vi "Current_Curve_Filtering.vi"() -> ()   [LabVIEW 2009]
uses:
  <vilib>/Analysis/3filter.llb/Butterworth Filter (DBL).vi
  Instance           3 31Saved   Current_vs_Length_2_log .vi
  Instance           2 31Saved   Current_vs_Length_2_log .vi
  <vilib>/Utility/file.llb/Write To Spreadsheet File (DBL).vi
  <vilib>/Utility/file.llb/Write To Spreadsheet File (I64).vi
  <vilib>/Analysis/NI_AALBase.lvlib
panel:
  out "residual":dbl=0.32609478757655186
  in  "Residual Cutoff Value":dbl=0.45
  out "XY Graph 3":cluster{dbl[], "Array":dbl[]}[](graph)
  in  "Save  2D Hist":bool
  out "G-Line":cluster{dbl[], i32[]}(graph)
  in  "Boolean":bool
  out "Cond. Max":dbl
  out "Cond. Min":dbl
  out "2D Histogram Max Values":cluster{sgl[], dbl[]}(graph)
  out "2D_G_Bins":dbl
  in  "PZT Sensitivty nm/V":dbl=3.89
  in  "Ramping Rate V/s":dbl=20.0
  out "Colormap 2":i32[][](graph)
  out "Current Bin2 (mV)":sgl=0.01
  out "Length Bin":sgl=0.015
  in  "log bins":i32=400
  out "XY Graph 2":cluster{dbl[], "Array":dbl[]}(graph)
  out "XY Graph":cluster{dbl[], "Array":dbl[]}(graph)
  out "Conductance (Go) 2":cluster{dbl, "SRat":dbl, "Filtered X":dbl[]}(graph)
  in  "Filter Freq":i32=9000
  in  "Units":bool
  in  "Bias Applied":dbl=0.1
  in  "Amplifier":dbl=1e-08
  in  "Copy Selected":bool
  in  "Subdirectory":string="Selected_Curves"
  out "String":string="Selection Criteria"
  in  "Step Height":i32=1
  in  "Decay":dbl=0.02
  in  "Max Counts":dbl=500000.0
  in  "Length %":i32=99
  in  "MIN":dbl=-2.0
  in  "MAX":dbl=0.9
  out "Curve Selected":bool
  out "shift value":dbl format="%.3f"
  in  "Zero calibrate":bool
  out "Linear Histogram":cluster{dbl, "Step":dbl, i32[]}(graph)
  out "Peak":cluster{dbl, "Step":dbl, i32[]}(graph)
  out "single":cluster{dbl, "Step":dbl, i32[]}(graph)
  out "writing to":path
  in  "TXT DIR":path=path "D:/Research/LabView/Processed_data"
  in  "Save TXT":bool
  out "Peak Histogram":cluster{dbl, "Step":dbl, i32[]}(graph)
  in  "Mode":bool=TRUE
  out "Total files":dbl
  in  "Current":u16
  in  "NEXT":bool
  in  "LAST":bool
  out "browsed":dbl
  out "selected":u16
  in  "add":bool
  in  "sub":bool
  in  "Peak Height":dbl=20.0 min=3.0 max=20.0 step=1.0
  in  "Peak width":i8=5 min=3 max=20 step=1
  in  "?":bool
  out "DL1520L-200mv":dbl[](array[numeric])=[1.0, 1.0, 1.0, 1.0, 1.0, 1.0, 1.0, 1.0, 1.0, 1.0, 1.0, 1.0, 1.0, 1.0, 1.0, 1.0, 1.0, 1.0, 1.0, 1.0, 1.0, 1.0, 1.0, 1.0, 1.0, 1.0, 1.0, 1.0, 1.0, 1.0, 1.0, 1.0, 1.0, 1.0, 1.0, 1.0, 1.0, 1.0, 1.0, 1.0, 1.0, 1.0, 1.0, 1.0, 1.0, 1.0, 1.0, 1.0, 1.0, 1.0, 1.0, 1.0, 1.0, 1.0, 1.0, 1.0, 1.0, 1.0, 1.0, 1.0, 1.0, 1.0, 1.0, 1.0, 1.0, 1.0, 1.0, 1.0, 1.0, 1.0, 1.0, 1.0, 1.0, 1.0, 1.0, 1.0, 1.0, 1.0, 1.0, 1.0, 1.0, 1.0, 1.0, 1.0, 1.0, 1.0, 1.0, 1.0, 1.0, 1.0, 1.0, 1.0, 1.0, 1.0, 1.0, 1.0, 1.0, 1.0, 1.0, 1.0, 1.0, 1.0, 1.0, 1.0, 1.0, 1.0, 1.0, 1.0, 1.0, 1.0, 1.0, 1.0, 1.0, 1.0, 1.0, 1.0, 1.0, 1.0, 1.0, 1.0, 1.0, 1.0, 1.0, 1.0, 1.0, 1.0518399477005005, 1.158460021018982, 0.8072500228881836, 1.076930046081543, 1.254330039024353, 0.9506000280380249, 1.0841000080108643, 0.7749999761581421, 1.0876799821853638, 1.0401999950408936, 1.1665300130844116, 1.0527399778366089, 0.8430899977684021, 1.1835500001907349, 1.0195900201797485, 1.0876799821853638, 1.0097299814224243, 0.8413000106811523, 0.9891300201416016, 1.0778299570083618, 1.100219964981079, 0.9317899942398071, 1.0894700288772583, 0.7767900228500366, 1.0661799907684326, 1.1916099786758423, 0.9022200107574463, 0.9631400108337402, 1.2498500347137451, 0.8654900193214417, 1.2104300260543823, 0.6486700177192688, 1.1190400123596191, 1.1217299699783325, 1.0097299814224243, 0.8081499934196472, 1.3242100477218628, 0.8063499927520752, 1.0751399993896484, 0.8905699849128723, 1.2713500261306763, 0.8583199977874756, 1.1504000425338745, 0.9237200021743774, 0.9694200158119202, 1.023169994354248, 1.017799973487854, 0.835919976234436, 0.9443299770355225, 1.2408900260925293, 0.8027700185775757, 1.0572199821472168, 1.1324800252914429, 1.07423996925354, 0.6997399926185608, 1.3197300434112549, 0.7803699970245361, 1.0267599821090698, 0.8511499762535095, 1.1512900590896606, 0.9559800028800964, 0.9909200072288513, 0.8009799718856812, 1.239989995956421, 1.0061500072479248, 0.936269998550415, 0.9577699899673462, 0.9774799942970276, 1.0751399993896484, 0.9640399813652039, 1.102910041809082, 0.8368200063705444, 0.946120023727417, 0.9828600287437439, 1.1208300590515137, 1.0527399778366089, 0.7418500185012817, 1.1943000555038452, 0.8395000100135803, 0.9676200151443481, 1.0410900115966797, 0.9936100244522095, 1.0043599605560303, 1.0195900201797485, 0.9201400279998779, 1.094849944114685, 0.8762400150299072, 0.9004300236701965, 1.0357199907302856, 1.1674200296401978, 0.9067000150680542, 1.0384000539779663, 0.8520500063896179, 1.1127699613571167, 0.9210399985313416, 0.9273099899291992, 0.8753399848937988, 1.0357199907302856, 1.179069995880127, 0.934469997882843, 1.0034600496292114, 1.1835500001907349, 0.7095900177955627, 0.9792699813842773, 1.1163500547409058, 0.8502600193023682, 1.1270999908447266, 1.0715500116348267, 0.8314399719238281, 1.155769944190979, 0.8771299719810486, 0.9335799813270569, 1.1199400424957275, 0.8350200057029724, 0.8681700229644775, 1.0831999778747559, 0.9299899935722351, 0.9532899856567383, 1.128000020980835, 0.8054599761962891, 1.0052499771118164, 1.128000020980835, 0.9138699769973755, 1.0142099857330322, 0.9057999849319458, 1.0939500331878662, 0.7526000142097473, 1.223870038986206, 0.7741000056266785, 1.023169994354248, 1.1781699657440186, 0.8332300186157227, 0.7955999970436096, 1.07423996925354, 1.0554300546646118, 0.9443299770355225, 0.9604600071907043, 1.1217299699783325, 0.9335799813270569, 0.9586700201034546, 0.8126299977302551, 1.0213799476623535, 0.9774799942970276, 1.0034600496292114, 0.997189998626709, 0.8511499762535095, 1.280310034751892, 0.857420027256012, 1.179960012435913, 0.8887799978256226, 0.8395000100135803, 0.8395000100135803, 1.2265499830245972, 0.8932600021362305, 0.9057999849319458, 1.0401999950408936, 0.8520500063896179, 1.2059500217437744, 1.0823099613189697, 0.6755499839782715, 1.1315799951553345, 0.9201400279998779, 1.0312399864196777, 0.8162099719047546, 1.2632900476455688, 0.976580023765564, 1.016010046005249, 0.9255099892616272, 1.1226199865341187, 0.7230299711227417, 1.3636300563812256, 0.7042199969291687, 1.1351699829101562, 0.9452300071716309, 1.0061500072479248, 0.9559800028800964, 1.062600016593933, 0.8466699719429016, 1.0581200122833252, 0.9479100108146667, 0.9909200072288513, 0.7741000056266785, 1.1736899614334106, 0.8045600056648254, 1.2032599449157715, 1.158460021018982, 0.8296499848365784, 1.0124200582504272, 0.9255099892616272, 0.9936100244522095, 1.097540020942688, 0.955079972743988, 1.0849900245666504, 0.8117300271987915, 1.0491600036621094, 1.062600016593933, 0.8224800229072571, 0.9658300280570984, 1.2722500562667847, 0.809939980506897, 1.1154600381851196, 0.8072500228881836, 1.017799973487854, 1.0384000539779663, 1.0652799606323242, 1.0321300029754639, 0.8466699719429016, 1.1136599779129028, 0.9479100108146667, 1.1736899614334106, 0.8654900193214417, 1.0491600036621094, 0.908490002155304, 1.0831999778747559, 0.8887799978256226, 1.417389988899231, 0.7920200228691101, 0.9299899935722351, 1.050950050354004, 0.9210399985313416, 1.2131099700927734, 1.0554300546646118, 0.9326800107955933, 1.0410900115966797, 1.0124200582504272, 0.7723100185394287, 1.14860999584198, 0.9183499813079834, 1.258810043334961, 1.1387499570846558, 0.7615600228309631, 1.0536400079727173, 1.0912699699401855, 1.1055999994277954, 0.9864400029182434, 1.102020025253296, 0.8395000100135803, 1.0518399477005005, 1.1647299528121948, 1.0536400079727173, 1.0903700590133667, 0.898639976978302, 1.0706599950790405, 0.8798199892044067, 1.2086299657821655, 1.2175899744033813, 0.9685199856758118, 0.9299899935722351, 1.2453700304031372, 0.9183499813079834, 1.0683399438858032, 1.1099599599838257, 0.8287299871444702, 1.1348299980163574, 1.1777299642562866, 1.002619981765747, 1.064460039138794, 0.7911900281906128, 1.0801000595092773, 1.0354299545288086, 1.1541199684143066, 1.0330699682235718, 0.8758800029754639, 1.143239974975586, 1.060479998588562, 1.069390058517456, 0.988099992275238, 0.8736900091171265, 0.9702600240707397, 1.0806699991226196, 1.105430006980896, 0.9094799757003784, 1.1135200262069702, 0.7833700180053711, 1.0633599758148193, 1.1603599786758423, 0.9031000137329102, 0.9701399803161621, 1.233780026435852, 0.8961600065231323, 1.1906499862670898, 0.6593499779701233, 1.1051499843597412, 1.1458200216293335, 0.9879999756813049, 0.8049200177192688, 1.3313599824905396, 0.8278599977493286, 1.0381699800491333, 0.9175699949264526, 1.2579900026321411, 0.8616999983787537, 1.143380045890808, 0.9292100071907043, 0.9623799920082092, 1.0555200576782227, 0.9838700294494629, 0.858959972858429, 0.9398900270462036, 1.2190099954605103, 0.8296499848365784, 1.0342299938201904, 1.13742995262146, 1.0622600317001343, 0.6929500102996826, 1.3546600341796875, 0.7598299980163574, 1.0298999547958374, 0.8505499958992004, 1.1496700048446655, 0.9482600092887878, 0.9879999756813049, 0.8200399875640869, 1.221750020980835, 0.992609977722168, 0.9523800015449524, 0.9264600276947021, 1.0212299823760986, 1.0299400091171265, 1.0182199478149414, 1.0560100078582764, 0.8834599852561951, 0.9059699773788452, 0.9895399808883667, 1.1484400033950806, 1.0384600162506104, 0.7316499948501587, 1.2115099430084229, 0.8419600129127502, 0.9686800241470337, 1.0195599794387817, 1.006790041923523, 1.0077199935913086, 0.9961599707603455, 0.9295700192451477, 1.091230034828186, 0.8798800110816956, 0.879580020904541, 1.0691100358963013, 1.1512999534606934, 0.9050300121307373, 1.054460048675537, 0.8385900259017944, 1.1123000383377075, 0.9119399785995483, 0.9419999718666077, 0.8851900100708008, 1.0197900533676147, 1.2030800580978394, 0.9083799719810486, 1.001520037651062, 1.2015999555587769, 0.6734499931335449, 1.0091999769210815, 1.102139949798584, 0.844539999961853, 1.1170300245285034, 1.064460039138794, 0.840470016002655, 1.149649977684021, 0.9002000093460083, 0.9479600191116333, 1.1135799884796143, 0.8381400108337402, 0.8478099703788757, 1.1067700386047363, 0.9128299951553345, 0.959659993648529, 1.1379300355911255, 0.7703099846839905, 1.0372799634933472, 1.107100009918213, 0.9234399795532227, 1.0169399976730347, 0.9108999967575073, 1.0801399946212769, 0.7652300000190735, 1.2206100225448608, 0.7879800200462341, 0.985759973526001, 1.2073700428009033, 0.8196899890899658, 0.804069995880127, 1.0743099451065063, 1.0461499691009521, 0.969980001449585, 0.9197400212287903, 1.1764299869537354, 0.89205002784729, 1.0055299997329712, 0.7935699820518494, 0.976859986782074, 1.006100058555603, 0.9770500063896179, 1.037160038948059, 0.8456100225448608, 1.2542500495910645, 0.8690800070762634, 1.1796799898147583, 0.880840003490448, 0.8596900105476379, 0.8223699927330017, 1.2430599927902222, 0.8662499785423279, 0.9478700160980225, 0.995389997959137, 0.9024500250816345, 1.200219988822937, 1.085710048675537, 0.6602299809455872, 1.1301900148391724, 0.9190300107002258, 1.029270052909851, 0.8400899767875671, 1.2397899627685547, 0.9429399967193604, 1.075279951095581, 0.8741999864578247, 1.184149980545044, 0.698360025882721, 1.3655699491500854, 0.7038400173187256, 1.114150047302246, 0.9856600165367126, 0.9702000021934509, 0.9700400233268738, 1.0714000463485718, 0.8154500126838684, 1.068910002708435, 0.9287599921226501, 0.9945600032806396, 0.7877600193023682, 1.1730799674987793, 0.8385400176048279, 1.1815299987792969, 1.1555500030517578, 0.8173999786376953, 0.9916300177574158, 0.9548199772834778, 0.9830399751663208, 1.1294000148773193, 0.9332299828529358, 1.129930019378662, 0.7542799711227417, 1.0674200057983398, 1.0660799741744995, 0.8366600275039673, 0.9412099719047546, 1.3048499822616577, 0.773169994354248, 1.1747000217437744, 0.7867599725723267, 1.0328500270843506, 1.008679986000061, 1.0926100015640259, 0.9909200072288513, 0.8855100274085999, 1.0829600095748901, 0.9591699838638306, 1.1888200044631958, 0.8604199886322021, 1.042580008506775, 0.8842300176620483, 1.092270016670227, 0.9145799875259399, 1.4063600301742554, 0.780019998550415, 0.9580699801445007, 1.0166599750518799, 0.9434900283813477, 1.209130048751831, 1.0414999723434448, 0.9523000121116638, 1.0370899438858032, 1.0564299821853638, 0.7244799733161926, 1.1851400136947632, 0.8989599943161011, 1.2469799518585205, 1.16989004611969, 0.7621200084686279, 1.055299997329712, 1.073009967803955, 1.1236900091171265, 1.0108699798583984, 1.057569980621338, 0.8584499955177307, 1.0296599864959717, 1.1820800304412842, 1.0370500087738037, 1.086899995803833, 0.9445199966430664, 1.0530200004577637, 0.8767600059509277, 1.1927000284194946, 1.2465300559997559, 0.9571999907493591, 0.9764000177383423, 1.195989966392517, 0.9126899838447571, 1.0990899801254272, 1.0919599533081055, 0.8234300017356873, 1.1401300430297852, 1.1347800493240356, 1.0098799467086792, 1.0518100261688232, 0.781499981880188, 1.1401300430297852, 1.0295100212097168, 1.1410200595855713, 1.0250500440597534, 0.8823099732398987, 1.1267499923706055, 1.0188000202178955, 1.0482399463653564, 1.0464600324630737, 0.8724899888038635, 0.9956099987030029, 1.0625200271606445, 1.0919599533081055, 0.9313700199127197, 1.0580600500106812, 0.78507000207901, 1.0464600324630737, 1.1642199754714966, 0.9599199891090393, 0.9465399980545044, 1.2418299913406372, 0.8894400000572205, 1.2088199853897095, 0.6503599882125854, 1.043779969215393, 1.1802799701690674, 0.9527900218963623, 0.8573300242424011, 1.3248000144958496, 0.8341299891471863, 1.031290054321289, 0.9090700149536133, 1.2614599466323853, 0.8055899739265442, 1.1285300254821777, 0.9866899847984314, 0.9536799788475037, 1.084820032119751, 0.9634900093078613, 0.8662499785423279, 0.9206699728965759, 1.192770004272461, 0.8448399901390076, 0.9982799887657166, 1.1829500198364258, 1.0455700159072876, 0.717270016670227, 1.3444299697875977, 0.7707899808883667, 1.0375399589538574, 0.8109400272369385, 1.1454800367355347, 0.9358299970626831, 0.9768700003623962, 0.8457300066947937, 1.255210041999817, 1.013450026512146, 0.9197800159454346, 0.9340500235557556, 1.0170199871063232, 0.9804400205612183, 1.0232599973678589, 1.0446699857711792, 0.9206699728965759, 0.9162099957466125, 0.9643800258636475, 1.1918699741363525, 1.0081000328063965, 0.7395700216293335, 1.1802799701690674, 0.8189700245857239, 0.9527900218963623, 1.0366400480270386, 1.0455700159072876, 1.0179100036621094, 1.0000699758529663, 0.9019299745559692, 1.1267499923706055, 0.8484100103378296, 0.8510800004005432, 1.0642999410629272, 1.1553000211715698, 0.9117500185966492, 1.09552001953125, 0.8368099927902222, 1.1178300380706787, 0.9028300046920776, 0.92781001329422, 0.8644700050354004, 1.0009599924087524, 1.1767100095748901, 0.9304800033569336, 1.0196900367736816, 1.2079299688339233, 0.690500020980835, 1.0321799516677856, 1.0839300155639648, 0.8260999917984009, 1.0883899927139282, 1.0616199970245361, 0.8430500030517578, 1.1829500198364258, 0.9206699728965759, 0.9179900288581848, 1.1651099920272827, 0.8082600235939026, 0.852869987487793, 1.0732200145721436, 0.8831999897956848, 0.9706299901008606, 1.1722500324249268, 0.7743600010871887, 1.0286200046539307, 1.09552001953125, 0.9679499864578247, 0.9938200116157532, 0.8760600090026855, 1.0544899702072144, 0.7440299987792969, 1.2873300313949585, 0.7922000288963318, 0.9938200116157532, 1.16867995262146, 0.830560028553009, 0.8484100103378296, 1.013450026512146, 1.0411100387573242, 0.9518899917602539, 0.9340500235557556, 1.2150700092315674, 0.8948000073432922, 1.0152299404144287, 0.7823899984359741, 0.9848999977111816, 1.0107699632644653, 0.9260200262069702, 1.0473500490188599, 0.8037999868392944, 1.3372900485992432, 0.8600000143051147, 1.192770004272461, 0.9019299745559692, 0.8270000219345093, 0.8314599990844727, 1.2284499406814575, 0.8368099927902222, 0.9153199791908264, 1.0268299579620361, 0.9206699728965759, 1.204360008239746, 1.1178300380706787, 0.6342999935150146, 1.1445900201797485, 0.9028300046920776, 0.9840099811553955, 0.835919976234436, 1.2712700366973877, 0.9857900142669678, 1.0491299629211426, 0.9090700149536133, 1.1740299463272095, 0.6922900080680847, 1.3515599966049194, 0.6717699766159058, 1.1097999811172485, 0.9902499914169312, 1.006309986114502, 0.9724100232124329, 1.0812499523162842, 0.8055899739265442, 1.067870020866394, 0.9295899868011475, 0.9857900142669678, 0.7511699795722961, 1.1704599857330322, 0.8912299871444702, 1.2061500549316406, 1.1294300556182861, 0.8385900259017944, 0.9795500040054321, 0.9643800258636475, 0.9857900142669678, 1.0642999410629272, 0.9304800033569336, 1.157080054283142, 0.7797099947929382, 1.09552001953125, 1.0660799741744995, 0.8189700245857239, 0.9492200016975403, 1.2784099578857422, 0.7707899808883667, 1.1722500324249268, 0.7725800275802612, 1.0892800092697144, 1.0107699632644653, 1.0892800092697144, 1.0081000328063965, 0.8501899838447571, 1.09552001953125, 0.9340500235557556, 1.1633299589157104, 0.8805199861526489, 1.0687600374221802, 0.8885499835014343, 1.1115800142288208, 0.9224500060081482, 1.3872499465942383, 0.7743600010871887, 0.9260200262069702, 0.9875800013542175, 0.9617099761962891, 1.2596700191497803, 1.0580600500106812, 0.9233499765396118, 1.0616199970245361, 1.0482399463653564, 0.7654399871826172, 1.1115800142288208, 0.9028300046920776, 1.2596700191497803, 1.2052600383758545, 0.7743600010871887, 1.0339699983596802, 1.0990899801254272, 1.104449987411499, 1.0339699983596802, 1.0188000202178955, 0.8323500156402588, 1.0651899576187134, 1.183840036392212, 1.0687600374221802, 1.0634100437164307, 0.9572499990463257, 1.0553799867630005, 0.8510800004005432, 1.166890025138855, 1.2543200254440308, 1.0027400255203247, 0.9777600169181824, 1.2338000535964966, 0.8787400126457214, 1.0004299879074097, 1.0473099946975708, 0.8730499744415283, 1.1065800189971924, 1.1543400287628174, 1.0278500318527222, 1.0384700298309326, 0.7819499969482422, 1.0747300386428833, 1.0570399761199951, 1.1286900043487549, 1.0402300357818604, 0.8774799704551697, 1.1746900081634521, 1.0322699546813965, 1.0375800132751465, 0.9995499849319458, 0.8394399881362915, 0.9862800240516663, 1.095960021018982, 1.0676599740982056, 0.9376299977302551, 1.0835800170898438, 0.8164399862289429, 1.0092799663543701, 1.1764600276947021, 0.9243599772453308, 0.9287800192832947, 1.2631399631500244, 0.8704000115394592, 1.204759955406189, 0.6474900245666504, 1.089769959449768, 1.1348799467086792, 0.979200005531311, 0.8385599851608276, 1.292330026626587, 0.8535900115966797, 1.0022000074386597, 0.9323199987411499, 1.257830023765564, 0.8182100057601929, 1.1693799495697021, 0.9279000163078308, 0.9508900046348572, 1.0641200542449951, 0.9836199879646301, 0.863319993019104, 0.9013599753379822, 1.2472200393676758, 0.784600019454956, 1.0535000562667847, 1.1454999446868896, 1.0526200532913208, 0.6864100098609924, 1.3498300313949585, 0.7739800214767456, 1.011929988861084, 0.9004799723625183, 1.1233799457550049, 0.9208199977874756, 0.9977800250053406, 0.7890200018882751, 1.2649099826812744, 0.9756600260734558, 0.9340900182723999, 0.979200005531311, 0.9482399821281433, 1.094190001487732, 0.9738900065422058, 1.065000057220459, 0.858020007610321, 0.8951699733734131, 1.0322699546813965, 1.1366499662399292, 1.0313899517059326, 0.7173699736595154, 1.207419991493225, 0.856249988079071, 0.9447000026702881, 1.0499600172042847, 0.980970025062561, 0.9898200035095215, 1.0048500299453735, 0.896049976348877, 1.1348799467086792, 0.8624399900436401, 0.890749990940094, 1.063230037689209, 1.1375399827957153, 0.9349700212478638, 0.9986600279808044, 0.8748199939727783, 1.089769959449768, 0.9517800211906433, 0.9155099987983704, 0.888979971408844, 1.0437699556350708, 1.1543400287628174, 0.9376299977302551, 0.9641600251197815, 1.2295299768447876, 0.6722599864006042, 0.9615100026130676, 1.141070008277893, 0.8385599851608276, 1.1313400268554688, 1.0561599731445312, 0.8350200057029724, 1.1693799495697021, 0.863319993019104, 0.9765499830245972, 1.098620057106018, 0.850059986114502, 0.8367900252342224, 1.124269962310791, 0.8969399929046631, 0.9632800221443176, 1.1171900033950806, 0.7881399989128113, 1.011929988861084, 1.1419600248336792, 0.8872100114822388, 1.0871200561523438, 0.8659800291061401, 1.095960021018982, 0.7952100038528442, 1.1605299711227417, 0.8102499842643738, 0.9641600251197815, 1.2153799533843994, 0.8102499842643738, 0.8111400008201599, 1.0756200551986694, 1.0296200513839722, 0.9898200035095215, 0.9137399792671204, 1.1985700130462646, 0.8836699724197388, 0.9915800094604492, 0.7996399998664856, 0.9632800221443176, 1.0340399742126465, 0.9986600279808044, 0.9933500289916992, 0.8765900135040283, 1.210070013999939, 0.9146299958229065, 1.1640700101852417, 0.8863199949264526, 0.8827800154685974, 0.8137900233268738, 1.2507599592208862, 0.8624399900436401, 0.938510000705719, 1.0384700298309326, 0.8456299901008606, 1.2259900569915771, 1.0331599712371826, 0.6828799843788147, 1.1870700120925903, 0.863319993019104, 1.0526200532913208, 0.8235200047492981, 1.2560700178146362, 0.9447000026702881, 1.065000057220459, 0.9225900173187256, 1.1366499662399292, 0.7359499931335449, 1.3002899885177612, 0.7456799745559692, 1.1472699642181396, 0.9606299996376038, 1.0048500299453735, 0.938510000705719, 1.091539978981018, 0.8049399852752686, 1.0818099975585938, 0.9323199987411499, 0.9800900220870972, 0.8208699822425842, 1.1295700073242188, 0.8739399909973145, 1.1499199867248535, 1.1861900091171265, 0.8093699812889099, 1.0004299879074097, 0.9924700260162354, 0.9349700212478638, 1.1384199857711792, 0.9588599801063538, 1.098620057106018, 0.815559983253479, 1.011929988861084, 1.1056900024414062, 0.8535900115966797, 0.929669976234436, 1.2994099855422974, 0.7775200009346008, 1.1897200345993042, 0.7757499814033508, 1.0375800132751465, 1.015470027923584, 1.1171900033950806, 0.9623900055885315, 0.8712900280952454, 1.1207300424575806, 0.9323199987411499, 1.239259958267212, 0.8288300037384033, 1.0597000122070312, 0.902239978313446, 1.065000057220459, 0.9358599781990051, 1.3834400177001953, 0.8014100193977356, 0.9853900074958801, 1.0022000074386597, 0.9668200016021729, 1.2286399602890015, 1.0526200532913208, 0.904009997844696, 1.0853500366210938, 1.0420000553131104, 0.7262200117111206, 1.1932599544525146, 0.9199399948120117, 1.2693300247192383, 1.1348799467086792, 0.8022900223731995, 1.0181200504302979, 1.122499942779541, 1.1127699613571167, 1.0145800113677979, 1.0667699575424194, 0.8332499861717224, 1.0579299926757812, 1.172029972076416, 1.0623500347137451, 1.0773899555206299, 0.9588599801063538, 1.0313899517059326, 0.9119700193405151, 1.205649971961975, 1.2675700187683105, 0.9323199987411499, 0.9712399840354919, 1.2436800003051758, 0.8810200095176697, 1.0145000219345093, 1.1491299867630005, 0.798229992389679, 1.130020022392273, 1.1474000215530396, 1.0066900253295898, 1.0310100317001343, 0.7556700110435486, 1.1222100257873535, 0.9745500087738037, 1.1830099821090698, 0.9910500049591064, 0.8894299864768982, 1.1022299528121948, 1.065750002861023, 1.0570600032806396, 0.9988700151443481, 0.8373100161552429, 0.9641299843788147, 1.0631400346755981, 1.0987600088119507, 0.902459979057312, 1.0900700092315674, 0.778249979019165, 1.0822499990463257, 1.130020022392273, 0.9007200002670288, 0.9276400208473206, 1.2246999740600586, 0.9007200002670288, 1.1908199787139893, 0.6219000220298767, 1.0961500406265259, 1.152609944343567, 0.9936599731445312, 0.7773799896240234, 1.297659993171692, 0.8468700051307678, 1.0344799757003784, 0.877269983291626, 1.2559700012207031, 0.8920300006866455, 1.1256799697875977, 0.9137499928474426, 0.9224299788475037, 1.0553300380706787, 0.9832299947738647, 0.8494700193405151, 0.9163500070571899, 1.2386000156402588, 0.781719982624054, 1.0327399969100952, 1.1647700071334839, 1.017109990119934, 0.7209200263023376, 1.3254499435424805, 0.7652199864387512, 1.0118999481201172, 0.823419988155365, 1.1482599973678589, 0.9502300024032593, 0.9832299947738647, 0.8138599991798401, 1.2116700410842896, 0.991919994354248, 0.931119978427887, 0.9537000060081482, 0.9693400263786316, 1.0666199922561646, 0.9884499907493591, 1.0466400384902954, 0.8928999900817871, 0.8824800252914429, 0.9910500049591064, 1.153480052947998, 1.0006099939346313, 0.7426400184631348, 1.1847399473190308, 0.8711900115013123, 0.9372000098228455, 1.0092899799346924, 1.0006099939346313, 0.9936599731445312, 0.9927899837493896, 0.9372000098228455, 1.0683499574661255, 0.8850799798965454, 0.8850799798965454, 1.0709600448608398, 1.143049955368042, 0.8824800252914429, 1.047510027885437, 0.8659800291061401, 1.0874600410461426, 0.9172199964523315, 0.9198300242424011, 0.9015899896621704, 1.0414299964904785, 1.173449993133545, 0.9215599894523621, 0.9606500267982483, 1.2134100198745728, 0.6549100279808044, 0.9728099703788757, 1.1395800113677979, 0.8164700269699097, 1.1639000177383423, 1.0145000219345093, 0.8633700013160706, 1.155210018157959, 0.8729199767112732, 0.9797599911689758, 1.072700023651123, 0.8659800291061401, 0.8355799913406372, 1.0961500406265259, 0.9120100140571594, 0.9450200200080872, 1.168239951133728, 0.738290011882782, 1.0579299926757812, 1.081380009651184, 0.9224299788475037, 1.0231900215148926, 0.9250400066375732, 1.0718300342559814, 0.7478500008583069, 1.230780005455017, 0.7756400108337402, 0.9806299805641174, 1.2194900512695312, 0.8112499713897705, 0.8225499987602234, 1.0466400384902954, 1.0631400346755981, 0.9571800231933594, 0.9180899858474731, 1.2047200202941895, 0.8790000081062317, 1.0075500011444092, 0.7843300104141235, 0.9623900055885315, 1.0275299549102783, 0.9632599949836731, 1.0483800172805786, 0.8242800235748291, 1.295050024986267, 0.8651099801063538, 1.2012499570846558, 0.8790000081062317, 0.8295000195503235, 0.8485999703407288, 1.1830099821090698, 0.9172199964523315, 0.9450200200080872, 0.9988700151443481, 0.8972399830818176, 1.1908199787139893, 1.09961998462677, 0.6722800135612488, 1.1265499591827393, 0.9207000136375427, 1.0362199544906616, 0.8668400049209595, 1.1943000555038452, 0.9927899837493896, 1.0370899438858032, 0.9250400066375732, 1.1639000177383423, 0.6887800097465515, 1.3680200576782227, 0.7209200263023376, 1.1152600049972534, 0.9962599873542786, 0.9867100119590759, 0.9597799777984619, 1.0970200300216675, 0.8208100199699402, 1.0492500066757202, 0.9502300024032593, 0.9815000295639038, 0.817330002784729, 1.1639000177383423, 0.8190699815750122, 1.216879963874817, 1.1474000215530396, 0.8642399907112122, 0.9597799777984619, 0.9754199981689453, 0.9945300221443176, 1.1169999837875366, 0.9597799777984619, 1.1057000160217285, 0.7851999998092651, 1.074429988861084, 1.0631400346755981, 0.8520799875259399, 0.9484900236129761, 1.3341399431228638, 0.763480007648468, 1.2012499570846558, 0.7834600210189819, 1.0448999404907227, 1.0266599655151367, 1.0865999460220337, 0.9710699915885925, 0.8833500146865845, 1.1196000576019287, 1.010159969329834, 1.18996000289917, 0.8685799837112427, 1.02839994430542, 0.9015899896621704, 1.111780047416687, 0.9302499890327454, 1.419260025024414, 0.7660899758338928, 0.991919994354248, 1.0318700075149536, 0.9545699954032898, 1.2099299430847168, 1.0518499612808228, 0.9519699811935425, 1.0527199506759644, 1.0614099502563477, 0.7660899758338928, 1.1569499969482422, 0.9641299843788147, 1.2377300262451172, 1.1882200241088867, 0.763480007648468, 1.0587999820709229, 1.111780047416687, 1.1378400325775146, 1.0344799757003784, 1.0527199506759644, 0.8963800072669983, 1.037950038909912, 1.210800051689148, 1.0145000219345093, 1.1126500368118286, 0.9623900055885315, 1.069219946861267, 0.9276400208473206, 1.153480052947998, 1.3150299787521362, 0.956309974193573, 0.9884499907493591, 1.2246999740600586, 0.9154800176620483, 1.0553300380706787, 1.0, 1.0, 1.0, 1.0, 1.0, 1.0, 1.0, 1.0, 1.0, 1.0, 1.0, 1.0, 1.0, 1.0, 1.0, 1.0, 1.0, 1.0, 1.0, 1.0, 1.0, 1.0, 1.0, 1.0, 1.0, 1.0, 1.0, 1.0, 1.0, 1.0, 1.0, 1.0, 1.0, 1.0, 1.0, 1.0, 1.0, 1.0, 1.0, 1.0, 1.0, 1.0, 1.0, 1.0, 1.0, 1.0, 1.0, 1.0, 1.0, 1.0, 1.0, 1.0, 1.0, 1.0, 1.0, 1.0, 1.0, 1.0, 1.0, 1.0, 1.0, 1.0, 1.0, 1.0, 1.0, 1.0, 1.0, 1.0, 1.0, 1.0, 1.0, 1.0, 1.0, 1.0, 1.0, 1.0, 1.0, 1.0, 1.0, 1.0, 1.0, 1.0, 1.0, 1.0, 1.0, 1.0, 1.0, 1.0, 1.0, 1.0, 1.0, 1.0, 1.0, 1.0, 1.0, 1.0, 1.0, 1.0, 1.0, 1.0, 1.0, 1.0, 1.0, 1.0, 1.0, 1.0, 1.0, 1.0, 1.0, 1.0, 1.0, 1.0, 1.0, 1.0, 1.0, 1.0, 1.0, 1.0, 1.0, 1.0, 1.0, 1.0, 1.0, 1.0] format="%.4f"
  in  "NIDL Correction":T1(ring)
  out "DL1520L-2V":dbl[](array[numeric])=[1.0, 1.0, 1.1071499586105347, 0.9460300207138062, 1.142799973487854, 1.0548499822616577, 0.6798099875450134, 1.1869399547576904, 0.9574499726295471, 1.0553699731826782, 0.9193099737167358, 1.0121500492095947, 0.8809400200843811, 0.8933200240135193, 1.2142599821090698, 0.9320200085639954, 0.867389976978302, 1.04121994972229, 0.8392800092697144, 1.3207199573516846, 0.8761799931526184, 0.9614599943161011, 0.8406999707221985, 1.3237199783325195, 0.842270016670227, 0.8019999861717224, 1.0565799474716187, 0.8988800048828125, 0.9938300251960754, 0.9866300225257874, 0.9458100199699402, 1.0645899772644043, 0.9812700152397156, 0.9915500283241272, 1.047860026359558, 0.7784900069236755, 0.9436100125312805, 1.1797200441360474, 0.9229199886322021, 0.8316299915313721, 1.06072998046875, 1.0812599658966064, 0.8902999758720398, 0.992579996585846, 0.983020007610321, 0.9313600063323975, 1.0070199966430664, 0.85794997215271, 1.0585600137710571, 0.8302099704742432, 1.0535399913787842, 1.0813499689102173, 1.0289100408554077, 0.7472900152206421, 0.977429986000061, 0.9230499863624573, 1.1730200052261353, 0.938759982585907, 0.6154199838638306, 1.0446100234985352, 1.1901600360870361, 0.8682100176811218, 0.9817299842834473, 0.950410008430481, 1.0137699842453003, 0.9678400158882141, 1.1657299995422363, 1.0292799472808838, 0.7897499799728394, 0.8259699940681458, 0.8726199865341187, 1.1850299835205078, 0.9300100207328796, 1.0324499607086182, 0.8647400140762329, 0.9773200154304504, 1.0006699562072754, 0.9293299913406372, 0.8785300254821777, 1.0564700365066528, 0.9852399826049805, 0.9670900106430054, 0.9886400103569031, 0.8383399844169617, 1.0759299993515015, 0.8722000122070312, 1.1963000297546387, 0.9250400066375732, 0.7123000025749207, 1.14274001121521, 1.097190022468567, 0.8719499707221985, 0.9584500193595886, 0.9225000143051147, 1.074280023574829, 1.0170899629592896, 0.756659984588623, 1.2385200262069702, 0.7658299803733826, 1.049090027809143, 0.8378199934959412, 1.1470099687576294, 0.8785899877548218, 0.9787899851799011, 1.00246000289917, 0.8198699951171875, 1.0823800563812256, 0.9904900193214417, 1.1441099643707275, 0.8393700122833252, 0.9125199913978577, 1.0177700519561768, 1.0600700378417969, 0.8316599726676941, 1.1464899778366089, 0.8072400093078613, 0.855400025844574, 1.0888500213623047, 1.0, 1.1690200567245483, 0.7053999900817871, 0.9819300174713135, 1.173799991607666, 0.8808599710464478, 1.0376299619674683, 0.883840024471283, 0.9901099801063538, 1.1312099695205688, 0.9692599773406982, 0.9967600107192993, 0.765720009803772, 1.2453299760818481, 0.8936399817466736, 1.043470025062561, 0.9276000261306763, 1.2058199644088745, 0.8945900201797485, 1.0330699682235718, 0.8693199753761292, 1.1636600494384766, 1.1312199831008911, 0.9562699794769287, 0.8316500186920166, 0.9096199870109558, 1.2192000150680542, 1.0195599794387817, 0.9311000108718872, 1.1465500593185425, 1.0913599729537964, 0.8537700176239014, 1.3184200525283813, 0.9644500017166138, 1.0194200277328491, 0.9502500295639038, 1.0557500123977661, 1.1233799457550049, 0.8309900164604187, 1.0903799533843994, 1.1363199949264526, 0.992169976234436, 1.0392800569534302, 1.0482699871063232, 0.9170600175857544, 1.1024999618530273, 1.0506600141525269, 1.0036300420761108, 1.1565699577331543, 0.7453500032424927, 1.1898800134658813, 0.8898800015449524, 1.207360029220581, 0.9647600054740906, 0.9409199953079224, 1.1513999700546265, 1.0830199718475342, 1.3117300271987915] format="%.5f"
  out "DL1520-2V":dbl[](array[numeric])=[0.9042699933052063, 0.8751500248908997, 1.1938999891281128, 0.8774200081825256, 1.1261299848556519, 1.0424100160598755, 0.8799999952316284, 0.9431099891662598, 1.1161799430847168, 0.9157999753952026, 1.1118199825286865, 1.0853400230407715, 0.983240008354187, 0.9828400015830994, 1.0612900257110596, 0.9332299828529358, 1.1189700365066528, 0.6911799907684326, 1.215109944343567, 0.921750009059906, 1.158869981765747, 0.8488900065422058, 1.0097500085830688, 1.0497299432754517, 0.8821499943733215, 1.0121699571609497, 1.2015700340270996, 0.8813199996948242, 0.9427800178527832, 0.9210500121116638, 1.036810040473938, 0.9211099743843079, 1.117069959640503, 0.9027000069618225, 1.030769944190979, 0.8944699764251709, 1.1112699508666992, 0.7450199723243713, 1.0670100450515747, 0.9704999923706055, 1.2049299478530884, 0.7958400249481201, 1.03410005569458, 0.8904100060462952, 0.8966599702835083, 1.0761699676513672, 0.784529983997345, 1.103909969329834, 0.9223999977111816, 1.0275700092315674, 0.914080023765564, 1.137220025062561, 0.8187599778175354, 0.9508200287818909, 1.1327999830245972, 0.8613799810409546, 1.0511300563812256, 1.0065900087356567, 0.9020299911499023, 1.0810799598693848, 1.08132004737854, 0.941789984703064, 0.8384000062942505, 0.845770001411438, 1.0647200345993042, 1.0405399799346924, 0.9768400192260742, 0.9739000201225281, 0.9725599884986877, 1.0460799932479858, 0.9323800206184387, 1.0303699970245361, 0.9656699895858765, 0.9442600011825562, 1.0794600248336792, 0.8691499829292297, 0.9040200114250183, 1.1154099702835083, 0.9336199760437012, 1.0413199663162231, 1.0063899755477905, 0.8839600086212158, 0.9992200136184692, 1.046839952468872, 0.9423099756240845, 1.0822499990463257, 0.8034200072288513, 1.0724799633026123, 0.8759899735450745, 1.0159300565719604, 1.0274300575256348, 0.9268100261688232, 1.0325599908828735, 0.990809977054596, 1.055459976196289, 1.0155099630355835, 0.7494500279426575, 1.001710057258606, 0.9849399924278259, 1.1800999641418457, 1.0796300172805786, 0.6667100191116333, 1.0151100158691406, 1.0528500080108643, 0.9521200060844421, 1.0733100175857544, 0.827530026435852, 1.0128200054168701, 1.029960036277771, 0.9591400027275085, 1.1652899980545044, 0.9207000136375427, 0.8044499754905701, 1.113610029220581, 0.7488800287246704, 1.0975799560546875, 1.1240400075912476, 0.9567199945449829, 1.0032000541687012, 1.06427001953125, 0.8525999784469604, 0.9700700044631958, 1.111050009727478, 0.9768099784851074, 1.0228500366210938, 0.9063699841499329, 1.069599986076355, 1.0788899660110474, 0.9706000089645386, 1.0519499778747559, 0.891700029373169, 0.9048900008201599, 1.134719967842102, 1.0879199504852295, 1.050879955291748, 0.9625999927520752, 1.0497900247573853, 0.9986199736595154, 1.01187002658844, 1.0264999866485596, 1.024459958076477, 0.994920015335083, 0.9977800250053406, 1.0359599590301514, 1.194599986076355, 0.8797000050544739, 1.15556001663208, 1.00246000289917, 0.9833899736404419, 1.1414400339126587, 1.0202800035476685, 0.9716600179672241, 1.1013599634170532, 1.0115200281143188, 1.2046600580215454, 1.0102699995040894, 0.9785400032997131, 1.097830057144165, 1.1012699604034424, 1.2504600286483765, 1.0140299797058105, 1.193850040435791, 0.9641199707984924, 1.0962599515914917, 1.2807300090789795, 0.9269800186157227] format="%.5f"
  out "X":dbl[](array[numeric])=[0.09600000455975533, 0.10000000474974513, 0.10400000493973494, 0.10800000512972474, 0.11200000531971455, 0.11600000550970435, 0.12000000569969416, 0.12400000588968396, 0.12800000607967377, 0.13200000626966357, 0.13600000645965338, 0.14000000664964318, 0.144000006839633, 0.1480000070296228, 0.1520000072196126, 0.1560000074096024, 0.1600000075995922, 0.16400000778958201, 0.16800000797957182, 0.17200000816956162, 0.17600000835955143, 0.18000000854954123, 0.18400000873953104, 0.18800000892952085, 0.19200000911951065, 0.19600000930950046, 0.20000000949949026, 0.20400000968948007, 0.20800000987946987, 0.21200001006945968, 0.21600001025944948, 0.2200000104494393, 0.2240000106394291, 0.2280000108294189, 0.2320000110194087, 0.2360000112093985, 0.2400000113993883, 0.24400001158937812, 0.24800001177936792, 0.25200001196935773, 0.25600001215934753, 0.26000001234933734, 0.26400001253932714, 0.26800001272931695, 0.27200001291930676, 0.27600001310929656, 0.28000001329928637, 0.28400001348927617, 0.288000013679266, 0.2920000138692558, 0.2960000140592456, 0.3000000142492354, 0.3040000144392252, 0.308000014629215, 0.3120000148192048, 0.3160000150091946, 0.3200000151991844, 0.3240000153891742, 0.32800001557916403, 0.33200001576915383, 0.33600001595914364, 0.34000001614913344, 0.34400001633912325, 0.34800001652911305, 0.35200001671910286, 0.35600001690909266, 0.36000001709908247, 0.3640000172890723, 0.3680000174790621, 0.3720000176690519, 0.3760000178590417, 0.3800000180490315, 0.3840000182390213, 0.3880000184290111, 0.3920000186190009, 0.3960000188089907, 0.4000000189989805, 0.4040000191889703, 0.40800001937896013, 0.41200001956894994, 0.41600001975893974, 0.42000001994892955, 0.42400002013891935, 0.42800002032890916, 0.43200002051889896, 0.43600002070888877, 0.4400000208988786, 0.4440000210888684, 0.4480000212788582, 0.452000021468848, 0.4560000216588378, 0.4600000218488276, 0.4640000220388174, 0.4680000222288072, 0.472000022418797, 0.4760000226087868, 0.4800000227987766, 0.48400002298876643, 0.48800002317875624, 0.49200002336874604, 0.49600002355873585, 0.5000000237487257, 0.5040000239387155, 0.5080000241287053, 0.5120000243186951, 0.5160000245086849, 0.5200000246986747, 0.5240000248886645, 0.5280000250786543, 0.5320000252686441, 0.5360000254586339, 0.5400000256486237, 0.5440000258386135, 0.5480000260286033, 0.5520000262185931, 0.5560000264085829, 0.5600000265985727, 0.5640000267885625, 0.5680000269785523, 0.5720000271685421, 0.576000027358532, 0.5800000275485218, 0.5840000277385116, 0.5880000279285014, 0.5920000281184912, 0.596000028308481, 0.6000000284984708, 0.6040000286884606, 0.6080000288784504, 0.6120000290684402, 0.61600002925843, 0.6200000294484198, 0.6240000296384096, 0.6280000298283994, 0.6320000300183892, 0.636000030208379, 0.6400000303983688, 0.6440000305883586, 0.6480000307783484, 0.6520000309683383, 0.6560000311583281, 0.6600000313483179, 0.6640000315383077, 0.6680000317282975, 0.6720000319182873, 0.6760000321082771, 0.6800000322982669, 0.6840000324882567, 0.6880000326782465, 0.6920000328682363, 0.6960000330582261, 0.7000000332482159, 0.7040000334382057, 0.7080000336281955, 0.7120000338181853, 0.7160000340081751, 0.7200000341981649, 0.7240000343881547, 0.7280000345781446, 0.7320000347681344, 0.7360000349581242, 0.740000035148114, 0.7440000353381038, 0.7480000355280936, 0.7520000357180834, 0.7560000359080732, 0.760000036098063, 0.7640000362880528, 0.7680000364780426, 0.7720000366680324, 0.7760000368580222, 0.780000037048012, 0.7840000372380018, 0.7880000374279916, 0.7920000376179814, 0.7960000378079712, 0.800000037997961, 0.8040000381879508, 0.8080000383779407, 0.8120000385679305, 0.8160000387579203, 0.8200000389479101, 0.8240000391378999, 0.8280000393278897, 0.8320000395178795, 0.8360000397078693, 0.8400000398978591, 0.8440000400878489, 0.8480000402778387, 0.8520000404678285, 0.8560000406578183, 0.8600000408478081, 0.8640000410377979, 0.8680000412277877, 0.8720000414177775, 0.8760000416077673, 0.8800000417977571, 0.884000041987747, 0.8880000421777368, 0.8920000423677266, 0.8960000425577164, 0.9000000427477062, 0.904000042937696, 0.9080000431276858, 0.9120000433176756, 0.9160000435076654, 0.9200000436976552, 0.924000043887645, 0.9280000440776348, 0.9320000442676246, 0.9360000444576144, 0.9400000446476042, 0.944000044837594, 0.9480000450275838, 0.9520000452175736, 0.9560000454075634, 0.9600000455975533, 0.9640000457875431, 0.9680000459775329, 0.9720000461675227, 0.9760000463575125, 0.9800000465475023, 0.9840000467374921, 0.9880000469274819, 0.9920000471174717, 0.9960000473074615, 1.0000000474974513, 1.004000047687441, 1.008000047877431, 1.0120000480674207, 1.0160000482574105, 1.0200000484474003, 1.0240000486373901, 1.02800004882738, 1.0320000490173697, 1.0360000492073596, 1.0400000493973494, 1.0440000495873392, 1.048000049777329, 1.0520000499673188, 1.0560000501573086, 1.0600000503472984, 1.0640000505372882, 1.068000050727278, 1.0720000509172678, 1.0760000511072576, 1.0800000512972474, 1.0840000514872372, 1.088000051677227, 1.0920000518672168, 1.0960000520572066, 1.1000000522471964, 1.1040000524371862, 1.108000052627176, 1.1120000528171659, 1.1160000530071557, 1.1200000531971455, 1.1240000533871353, 1.128000053577125, 1.1320000537671149, 1.1360000539571047, 1.1400000541470945, 1.1440000543370843, 1.148000054527074, 1.152000054717064, 1.1560000549070537, 1.1600000550970435, 1.1640000552870333, 1.1680000554770231, 1.172000055667013, 1.1760000558570027, 1.1800000560469925, 1.1840000562369823, 1.1880000564269722, 1.192000056616962, 1.1960000568069518, 1.2000000569969416, 1.2040000571869314, 1.2080000573769212, 1.212000057566911, 1.2160000577569008, 1.2200000579468906, 1.2240000581368804, 1.2280000583268702, 1.23200005851686, 1.2360000587068498, 1.2400000588968396, 1.2440000590868294, 1.2480000592768192, 1.252000059466809, 1.2560000596567988, 1.2600000598467886, 1.2640000600367785, 1.2680000602267683, 1.272000060416758, 1.2760000606067479, 1.2800000607967377, 1.2840000609867275, 1.2880000611767173, 1.292000061366707, 1.296000061556697, 1.3000000617466867, 1.3040000619366765, 1.3080000621266663, 1.3120000623166561, 1.316000062506646, 1.3200000626966357, 1.3240000628866255, 1.3280000630766153, 1.3320000632666051, 1.336000063456595, 1.3400000636465847, 1.3440000638365746, 1.3480000640265644, 1.3520000642165542, 1.356000064406544, 1.3600000645965338, 1.3640000647865236, 1.3680000649765134, 1.3720000651665032, 1.376000065356493, 1.3800000655464828, 1.3840000657364726, 1.3880000659264624, 1.3920000661164522, 1.396000066306442, 1.4000000664964318, 1.4040000666864216, 1.4080000668764114, 1.4120000670664012, 1.416000067256391, 1.4200000674463809, 1.4240000676363707, 1.4280000678263605, 1.4320000680163503, 1.43600006820634, 1.4400000683963299, 1.4440000685863197, 1.4480000687763095, 1.4520000689662993, 1.456000069156289, 1.460000069346279, 1.4640000695362687, 1.4680000697262585, 1.4720000699162483, 1.4760000701062381, 1.480000070296228, 1.4840000704862177, 1.4880000706762075, 1.4920000708661973, 1.4960000710561872, 1.500000071246177, 1.5040000714361668, 1.5080000716261566, 1.5120000718161464, 1.5160000720061362, 1.520000072196126, 1.5240000723861158, 1.5280000725761056, 1.5320000727660954, 1.5360000729560852, 1.540000073146075, 1.5440000733360648, 1.5480000735260546, 1.5520000737160444, 1.5560000739060342, 1.560000074096024, 1.5640000742860138, 1.5680000744760036, 1.5720000746659935, 1.5760000748559833, 1.580000075045973, 1.5840000752359629, 1.5880000754259527, 1.5920000756159425, 1.5960000758059323, 1.600000075995922, 1.604000076185912, 1.6080000763759017, 1.6120000765658915, 1.6160000767558813, 1.6200000769458711, 1.624000077135861, 1.6280000773258507, 1.6320000775158405, 1.6360000777058303, 1.6400000778958201, 1.64400007808581, 1.6480000782757998, 1.6520000784657896, 1.6560000786557794, 1.6600000788457692, 1.664000079035759, 1.6680000792257488, 1.6720000794157386, 1.6760000796057284, 1.6800000797957182, 1.684000079985708, 1.6880000801756978, 1.6920000803656876, 1.6960000805556774, 1.7000000807456672, 1.704000080935657, 1.7080000811256468, 1.7120000813156366, 1.7160000815056264, 1.7200000816956162, 1.724000081885606, 1.7280000820755959, 1.7320000822655857, 1.7360000824555755, 1.7400000826455653, 1.744000082835555, 1.7480000830255449, 1.7520000832155347, 1.7560000834055245, 1.7600000835955143, 1.764000083785504, 1.768000083975494, 1.7720000841654837, 1.7760000843554735, 1.7800000845454633, 1.7840000847354531, 1.788000084925443, 1.7920000851154327, 1.7960000853054225, 1.8000000854954123, 1.8040000856854022, 1.808000085875392, 1.8120000860653818, 1.8160000862553716, 1.8200000864453614, 1.8240000866353512, 1.828000086825341, 1.8320000870153308, 1.8360000872053206, 1.8400000873953104, 1.8440000875853002, 1.84800008777529, 1.8520000879652798, 1.8560000881552696, 1.8600000883452594, 1.8640000885352492, 1.868000088725239, 1.8720000889152288, 1.8760000891052186, 1.8800000892952085, 1.8840000894851983, 1.888000089675188, 1.8920000898651779, 1.8960000900551677, 1.9000000902451575, 1.9040000904351473, 1.908000090625137, 1.912000090815127, 1.9160000910051167, 1.9200000911951065, 1.9240000913850963, 1.9280000915750861, 1.932000091765076, 1.9360000919550657, 1.9400000921450555, 1.9440000923350453, 1.9480000925250351, 1.952000092715025, 1.9560000929050148, 1.9600000930950046, 1.9640000932849944, 1.9680000934749842, 1.972000093664974, 1.9760000938549638, 1.9800000940449536, 1.9840000942349434, 1.9880000944249332, 1.992000094614923, 1.9960000948049128, 2.0000000949949026, 2.0040000951848924, 2.008000095374882, 2.012000095564872, 2.016000095754862, 2.0200000959448516, 2.0240000961348414, 2.0280000963248312, 2.032000096514821, 2.036000096704811, 2.0400000968948007, 2.0440000970847905, 2.0480000972747803, 2.05200009746477, 2.05600009765476, 2.0600000978447497, 2.0640000980347395, 2.0680000982247293, 2.072000098414719, 2.076000098604709, 2.0800000987946987, 2.0840000989846885, 2.0880000991746783, 2.092000099364668, 2.096000099554658, 2.1000000997446477, 2.1040000999346375, 2.1080001001246274, 2.112000100314617, 2.116000100504607, 2.1200001006945968, 2.1240001008845866, 2.1280001010745764, 2.132000101264566, 2.136000101454556, 2.140000101644546, 2.1440001018345356, 2.1480001020245254, 2.152000102214515, 2.156000102404505, 2.160000102594495, 2.1640001027844846, 2.1680001029744744, 2.1720001031644642, 2.176000103354454, 2.180000103544444, 2.1840001037344337, 2.1880001039244235, 2.1920001041144133, 2.196000104304403, 2.200000104494393, 2.2040001046843827, 2.2080001048743725, 2.2120001050643623, 2.216000105254352, 2.220000105444342, 2.2240001056343317, 2.2280001058243215, 2.2320001060143113, 2.236000106204301, 2.240000106394291, 2.2440001065842807, 2.2480001067742705, 2.2520001069642603, 2.25600010715425, 2.26000010734424, 2.2640001075342298, 2.2680001077242196, 2.2720001079142094, 2.276000108104199, 2.280000108294189, 2.284000108484179, 2.2880001086741686, 2.2920001088641584, 2.296000109054148, 2.300000109244138, 2.304000109434128, 2.3080001096241176, 2.3120001098141074, 2.3160001100040972, 2.320000110194087, 2.324000110384077, 2.3280001105740666, 2.3320001107640564, 2.3360001109540462, 2.340000111144036, 2.344000111334026, 2.3480001115240157, 2.3520001117140055, 2.3560001119039953, 2.360000112093985, 2.364000112283975, 2.3680001124739647, 2.3720001126639545, 2.3760001128539443, 2.380000113043934, 2.384000113233924, 2.3880001134239137, 2.3920001136139035, 2.3960001138038933, 2.400000113993883, 2.404000114183873, 2.4080001143738627, 2.4120001145638525, 2.4160001147538424, 2.420000114943832, 2.424000115133822, 2.4280001153238118, 2.4320001155138016, 2.4360001157037914, 2.440000115893781, 2.444000116083771, 2.448000116273761, 2.4520001164637506, 2.4560001166537404, 2.46000011684373, 2.46400011703372, 2.46800011722371, 2.4720001174136996, 2.4760001176036894, 2.4800001177936792, 2.484000117983669, 2.488000118173659, 2.4920001183636487, 2.4960001185536385, 2.5000001187436283, 2.504000118933618, 2.508000119123608, 2.5120001193135977, 2.5160001195035875, 2.5200001196935773, 2.524000119883567, 2.528000120073557, 2.5320001202635467, 2.5360001204535365, 2.5400001206435263, 2.544000120833516, 2.548000121023506, 2.5520001212134957, 2.5560001214034855, 2.5600001215934753, 2.564000121783465, 2.568000121973455, 2.5720001221634448, 2.5760001223534346, 2.5800001225434244, 2.584000122733414, 2.588000122923404, 2.592000123113394, 2.5960001233033836, 2.6000001234933734, 2.604000123683363, 2.608000123873353, 2.612000124063343, 2.6160001242533326, 2.6200001244433224, 2.6240001246333122, 2.628000124823302, 2.632000125013292, 2.6360001252032816, 2.6400001253932714, 2.6440001255832613, 2.648000125773251, 2.652000125963241, 2.6560001261532307, 2.6600001263432205, 2.6640001265332103, 2.6680001267232, 2.67200012691319, 2.6760001271031797, 2.6800001272931695, 2.6840001274831593, 2.688000127673149, 2.692000127863139, 2.6960001280531287, 2.7000001282431185, 2.7040001284331083, 2.708000128623098, 2.712000128813088, 2.7160001290030777, 2.7200001291930676, 2.7240001293830574, 2.728000129573047, 2.732000129763037, 2.7360001299530268, 2.7400001301430166, 2.7440001303330064, 2.748000130522996, 2.752000130712986, 2.756000130902976, 2.7600001310929656, 2.7640001312829554, 2.768000131472945, 2.772000131662935, 2.776000131852925, 2.7800001320429146, 2.7840001322329044, 2.7880001324228942, 2.792000132612884, 2.796000132802874, 2.8000001329928637, 2.8040001331828535, 2.8080001333728433, 2.812000133562833, 2.816000133752823, 2.8200001339428127, 2.8240001341328025, 2.8280001343227923, 2.832000134512782, 2.836000134702772, 2.8400001348927617, 2.8440001350827515, 2.8480001352727413, 2.852000135462731, 2.856000135652721, 2.8600001358427107, 2.8640001360327005, 2.8680001362226903, 2.87200013641268, 2.87600013660267, 2.8800001367926598, 2.8840001369826496, 2.8880001371726394, 2.892000137362629, 2.896000137552619, 2.900000137742609, 2.9040001379325986, 2.9080001381225884, 2.912000138312578, 2.916000138502568, 2.920000138692558, 2.9240001388825476, 2.9280001390725374, 2.9320001392625272, 2.936000139452517, 2.940000139642507, 2.9440001398324966, 2.9480001400224864, 2.9520001402124763, 2.956000140402466, 2.960000140592456, 2.9640001407824457, 2.9680001409724355, 2.9720001411624253, 2.976000141352415, 2.980000141542405, 2.9840001417323947, 2.9880001419223845, 2.9920001421123743, 2.996000142302364, 3.000000142492354, 3.0040001426823437, 3.0080001428723335, 3.0120001430623233, 3.016000143252313, 3.020000143442303, 3.0240001436322927, 3.0280001438222826, 3.0320001440122724, 3.036000144202262, 3.040000144392252, 3.0440001445822418, 3.0480001447722316, 3.0520001449622214, 3.056000145152211, 3.060000145342201, 3.064000145532191, 3.0680001457221806, 3.0720001459121704, 3.07600014610216, 3.08000014629215, 3.08400014648214, 3.0880001466721296, 3.0920001468621194, 3.0960001470521092, 3.100000147242099, 3.104000147432089, 3.1080001476220787, 3.1120001478120685, 3.1160001480020583, 3.120000148192048, 3.124000148382038, 3.1280001485720277, 3.1320001487620175, 3.1360001489520073, 3.140000149141997, 3.144000149331987, 3.1480001495219767, 3.1520001497119665, 3.1560001499019563, 3.160000150091946, 3.164000150281936, 3.1680001504719257, 3.1720001506619155, 3.1760001508519053, 3.180000151041895, 3.184000151231885, 3.1880001514218748, 3.1920001516118646, 3.1960001518018544, 3.200000151991844, 3.204000152181834, 3.208000152371824, 3.2120001525618136, 3.2160001527518034, 3.220000152941793, 3.224000153131783, 3.228000153321773, 3.2320001535117626, 3.2360001537017524, 3.2400001538917422, 3.244000154081732, 3.248000154271722, 3.2520001544617116, 3.2560001546517015, 3.2600001548416913, 3.264000155031681, 3.268000155221671, 3.2720001554116607, 3.2760001556016505, 3.2800001557916403, 3.28400015598163, 3.28800015617162, 3.2920001563616097, 3.2960001565515995, 3.3000001567415893, 3.304000156931579, 3.308000157121569, 3.3120001573115587, 3.3160001575015485, 3.3200001576915383, 3.324000157881528, 3.328000158071518, 3.3320001582615077, 3.3360001584514976, 3.3400001586414874, 3.344000158831477, 3.348000159021467, 3.3520001592114568, 3.3560001594014466, 3.3600001595914364, 3.364000159781426, 3.368000159971416, 3.372000160161406, 3.3760001603513956, 3.3800001605413854, 3.384000160731375, 3.388000160921365, 3.392000161111355, 3.3960001613013446, 3.4000001614913344, 3.4040001616813242, 3.408000161871314, 3.412000162061304, 3.4160001622512937, 3.4200001624412835, 3.4240001626312733, 3.428000162821263, 3.432000163011253, 3.4360001632012427, 3.4400001633912325, 3.4440001635812223, 3.448000163771212, 3.452000163961202, 3.4560001641511917, 3.4600001643411815, 3.4640001645311713, 3.468000164721161, 3.472000164911151, 3.4760001651011407, 3.4800001652911305, 3.4840001654811203, 3.48800016567111, 3.4920001658611, 3.4960001660510898, 3.5000001662410796, 3.5040001664310694, 3.508000166621059, 3.512000166811049, 3.516000167001039, 3.5200001671910286, 3.5240001673810184, 3.528000167571008, 3.532000167760998, 3.536000167950988, 3.5400001681409776, 3.5440001683309674, 3.5480001685209572, 3.552000168710947, 3.556000168900937, 3.5600001690909266, 3.5640001692809165, 3.5680001694709063, 3.572000169660896, 3.576000169850886, 3.5800001700408757, 3.5840001702308655, 3.5880001704208553, 3.592000170610845, 3.596000170800835, 3.6000001709908247, 3.6040001711808145, 3.6080001713708043, 3.612000171560794, 3.616000171750784, 3.6200001719407737, 3.6240001721307635, 3.6280001723207533, 3.632000172510743, 3.636000172700733, 3.6400001728907228, 3.6440001730807126, 3.6480001732707024, 3.652000173460692, 3.656000173650682, 3.6600001738406718, 3.6640001740306616, 3.6680001742206514, 3.672000174410641, 3.676000174600631, 3.680000174790621, 3.6840001749806106, 3.6880001751706004, 3.69200017536059, 3.69600017555058, 3.70000017574057, 3.7040001759305596, 3.7080001761205494, 3.7120001763105392, 3.716000176500529, 3.720000176690519, 3.7240001768805087, 3.7280001770704985, 3.7320001772604883, 3.736000177450478, 3.740000177640468, 3.7440001778304577, 3.7480001780204475, 3.7520001782104373, 3.756000178400427, 3.760000178590417, 3.7640001787804067, 3.7680001789703965, 3.7720001791603863, 3.776000179350376, 3.780000179540366, 3.7840001797303557, 3.7880001799203455, 3.7920001801103354, 3.796000180300325, 3.800000180490315, 3.8040001806803048, 3.8080001808702946, 3.8120001810602844, 3.816000181250274, 3.820000181440264, 3.824000181630254, 3.8280001818202436, 3.8320001820102334, 3.836000182200223, 3.840000182390213, 3.844000182580203, 3.8480001827701926, 3.8520001829601824, 3.8560001831501722, 3.860000183340162, 3.864000183530152, 3.8680001837201416, 3.8720001839101315, 3.8760001841001213, 3.880000184290111, 3.884000184480101, 3.8880001846700907, 3.8920001848600805, 3.8960001850500703, 3.90000018524006, 3.90400018543005, 3.9080001856200397, 3.9120001858100295, 3.9160001860000193, 3.920000186190009, 3.924000186379999, 3.9280001865699887, 3.9320001867599785, 3.9360001869499683, 3.940000187139958, 3.944000187329948, 3.9480001875199378, 3.9520001877099276, 3.9560001878999174, 3.960000188089907, 3.964000188279897, 3.968000188469887, 3.9720001886598766, 3.9760001888498664, 3.980000189039856, 3.984000189229846, 3.988000189419836, 3.9920001896098256, 3.9960001897998154, 4.000000189989805, 4.004000190179795, 4.008000190369785, 4.012000190559775, 4.016000190749764, 4.020000190939754, 4.024000191129744, 4.028000191319734, 4.032000191509724, 4.0360001916997135, 4.040000191889703, 4.044000192079693, 4.048000192269683, 4.052000192459673, 4.0560001926496625, 4.060000192839652, 4.064000193029642, 4.068000193219632, 4.072000193409622, 4.0760001935996115, 4.080000193789601, 4.084000193979591, 4.088000194169581, 4.092000194359571, 4.0960001945495605, 4.10000019473955, 4.10400019492954, 4.10800019511953, 4.11200019530952, 4.11600019549951, 4.120000195689499, 4.124000195879489, 4.128000196069479, 4.132000196259469, 4.136000196449459, 4.140000196639448, 4.144000196829438, 4.148000197019428, 4.152000197209418, 4.156000197399408, 4.160000197589397, 4.164000197779387, 4.168000197969377, 4.172000198159367, 4.176000198349357, 4.1800001985393465, 4.184000198729336, 4.188000198919326, 4.192000199109316, 4.196000199299306, 4.2000001994892955, 4.204000199679285, 4.208000199869275, 4.212000200059265, 4.216000200249255, 4.2200002004392445, 4.224000200629234, 4.228000200819224, 4.232000201009214, 4.236000201199204, 4.2400002013891935, 4.244000201579183, 4.248000201769173, 4.252000201959163, 4.256000202149153, 4.260000202339143, 4.264000202529132, 4.268000202719122, 4.272000202909112, 4.276000203099102, 4.280000203289092, 4.284000203479081, 4.288000203669071, 4.292000203859061, 4.296000204049051, 4.300000204239041, 4.30400020442903, 4.30800020461902, 4.31200020480901, 4.316000204999, 4.32000020518899, 4.3240002053789794, 4.328000205568969, 4.332000205758959, 4.336000205948949, 4.340000206138939, 4.3440002063289285, 4.348000206518918, 4.352000206708908, 4.356000206898898, 4.360000207088888, 4.3640002072788775, 4.368000207468867, 4.372000207658857, 4.376000207848847, 4.380000208038837, 4.3840002082288265, 4.388000208418816, 4.392000208608806, 4.396000208798796, 4.400000208988786, 4.4040002091787755, 4.408000209368765, 4.412000209558755, 4.416000209748745, 4.420000209938735, 4.424000210128725, 4.428000210318714, 4.432000210508704, 4.436000210698694, 4.440000210888684, 4.444000211078674, 4.448000211268663, 4.452000211458653, 4.456000211648643, 4.460000211838633, 4.464000212028623, 4.468000212218612, 4.472000212408602, 4.476000212598592, 4.480000212788582, 4.484000212978572, 4.4880002131685615, 4.492000213358551, 4.496000213548541, 4.500000213738531, 4.504000213928521, 4.5080002141185105, 4.5120002143085, 4.51600021449849, 4.52000021468848, 4.52400021487847, 4.5280002150684595, 4.532000215258449, 4.536000215448439, 4.540000215638429, 4.544000215828419, 4.5480002160184085, 4.552000216208398, 4.556000216398388, 4.560000216588378, 4.564000216778368, 4.568000216968358, 4.572000217158347, 4.576000217348337, 4.580000217538327, 4.584000217728317, 4.588000217918307, 4.592000218108296, 4.596000218298286, 4.600000218488276, 4.604000218678266, 4.608000218868256, 4.612000219058245, 4.616000219248235, 4.620000219438225, 4.624000219628215, 4.628000219818205, 4.6320002200081944, 4.636000220198184, 4.640000220388174, 4.644000220578164, 4.648000220768154, 4.6520002209581435, 4.656000221148133, 4.660000221338123, 4.664000221528113, 4.668000221718103, 4.6720002219080925, 4.676000222098082, 4.680000222288072, 4.684000222478062, 4.688000222668052, 4.6920002228580415, 4.696000223048031, 4.700000223238021, 4.704000223428011, 4.708000223618001, 4.7120002238079906, 4.71600022399798, 4.72000022418797, 4.72400022437796, 4.72800022456795, 4.73200022475794, 4.736000224947929, 4.740000225137919, 4.744000225327909, 4.748000225517899, 4.752000225707889, 4.756000225897878, 4.760000226087868, 4.764000226277858, 4.768000226467848, 4.772000226657838, 4.776000226847827, 4.780000227037817, 4.784000227227807, 4.788000227417797, 4.792000227607787, 4.7960002277977765, 4.800000227987766, 4.804000228177756, 4.808000228367746, 4.812000228557736, 4.8160002287477255, 4.820000228937715, 4.824000229127705, 4.828000229317695, 4.832000229507685, 4.8360002296976745, 4.840000229887664, 4.844000230077654, 4.848000230267644, 4.852000230457634, 4.8560002306476235, 4.860000230837613, 4.864000231027603, 4.868000231217593, 4.872000231407583, 4.876000231597573, 4.880000231787562, 4.884000231977552, 4.888000232167542, 4.892000232357532, 4.896000232547522, 4.900000232737511, 4.904000232927501, 4.908000233117491, 4.912000233307481, 4.916000233497471, 4.92000023368746, 4.92400023387745, 4.92800023406744, 4.93200023425743, 4.93600023444742, 4.9400002346374094, 4.944000234827399, 4.948000235017389, 4.952000235207379, 4.956000235397369, 4.9600002355873585, 4.964000235777348, 4.968000235967338, 4.972000236157328, 4.976000236347318, 4.9800002365373075, 4.984000236727297, 4.988000236917287, 4.992000237107277, 4.996000237297267, 5.0000002374872565, 5.004000237677246, 5.008000237867236, 5.012000238057226, 5.016000238247216, 5.0200002384372056, 5.024000238627195, 5.028000238817185, 5.032000239007175, 5.036000239197165, 5.040000239387155, 5.044000239577144, 5.048000239767134, 5.052000239957124, 5.056000240147114, 5.060000240337104, 5.064000240527093, 5.068000240717083, 5.072000240907073, 5.076000241097063, 5.080000241287053, 5.084000241477042, 5.088000241667032, 5.092000241857022, 5.096000242047012, 5.100000242237002, 5.1040002424269915, 5.108000242616981, 5.112000242806971, 5.116000242996961, 5.120000243186951, 5.1240002433769405, 5.12800024356693, 5.13200024375692, 5.13600024394691, 5.1400002441369, 5.1440002443268895, 5.148000244516879, 5.152000244706869, 5.156000244896859, 5.160000245086849, 5.1640002452768385, 5.168000245466828, 5.172000245656818, 5.176000245846808, 5.180000246036798, 5.184000246226788, 5.188000246416777, 5.192000246606767, 5.196000246796757, 5.200000246986747, 5.204000247176737, 5.208000247366726, 5.212000247556716, 5.216000247746706, 5.220000247936696, 5.224000248126686, 5.228000248316675, 5.232000248506665, 5.236000248696655, 5.240000248886645, 5.244000249076635, 5.2480002492666245, 5.252000249456614, 5.256000249646604, 5.260000249836594, 5.264000250026584, 5.2680002502165735, 5.272000250406563, 5.276000250596553, 5.280000250786543, 5.284000250976533, 5.2880002511665225, 5.292000251356512, 5.296000251546502, 5.300000251736492, 5.304000251926482, 5.3080002521164715, 5.312000252306461, 5.316000252496451, 5.320000252686441, 5.324000252876431, 5.3280002530664206, 5.33200025325641, 5.3360002534464, 5.34000025363639, 5.34400025382638, 5.34800025401637, 5.352000254206359, 5.356000254396349, 5.360000254586339, 5.364000254776329, 5.368000254966319, 5.372000255156308, 5.376000255346298, 5.380000255536288, 5.384000255726278, 5.388000255916268, 5.392000256106257, 5.396000256296247, 5.400000256486237, 5.404000256676227, 5.408000256866217, 5.4120002570562065, 5.416000257246196, 5.420000257436186, 5.424000257626176, 5.428000257816166, 5.4320002580061555, 5.436000258196145, 5.440000258386135, 5.444000258576125, 5.448000258766115, 5.4520002589561045, 5.456000259146094, 5.460000259336084, 5.464000259526074, 5.468000259716064, 5.4720002599060535, 5.476000260096043, 5.480000260286033, 5.484000260476023, 5.488000260666013, 5.492000260856003, 5.496000261045992, 5.500000261235982, 5.504000261425972, 5.508000261615962, 5.512000261805952, 5.516000261995941, 5.520000262185931, 5.524000262375921, 5.528000262565911, 5.532000262755901, 5.53600026294589, 5.54000026313588, 5.54400026332587, 5.54800026351586, 5.55200026370585, 5.5560002638958395, 5.560000264085829, 5.564000264275819, 5.568000264465809, 5.572000264655799, 5.5760002648457885, 5.580000265035778, 5.584000265225768, 5.588000265415758, 5.592000265605748, 5.5960002657957375, 5.600000265985727, 5.604000266175717, 5.608000266365707, 5.612000266555697, 5.6160002667456865, 5.620000266935676, 5.624000267125666, 5.628000267315656, 5.632000267505646, 5.636000267695636, 5.640000267885625, 5.644000268075615, 5.648000268265605, 5.652000268455595, 5.656000268645585, 5.660000268835574, 5.664000269025564, 5.668000269215554, 5.672000269405544, 5.676000269595534, 5.680000269785523, 5.684000269975513, 5.688000270165503, 5.692000270355493, 5.696000270545483, 5.700000270735472, 5.704000270925462, 5.708000271115452, 5.712000271305442, 5.716000271495432, 5.7200002716854215, 5.724000271875411, 5.728000272065401, 5.732000272255391, 5.736000272445381, 5.7400002726353705, 5.74400027282536, 5.74800027301535, 5.75200027320534, 5.75600027339533, 5.7600002735853195, 5.764000273775309, 5.768000273965299, 5.772000274155289, 5.776000274345279, 5.7800002745352685, 5.784000274725258, 5.788000274915248, 5.792000275105238, 5.796000275295228, 5.800000275485218, 5.804000275675207, 5.808000275865197, 5.812000276055187, 5.816000276245177, 5.820000276435167, 5.824000276625156, 5.828000276815146, 5.832000277005136, 5.836000277195126, 5.840000277385116, 5.844000277575105, 5.848000277765095, 5.852000277955085, 5.856000278145075, 5.860000278335065, 5.8640002785250545, 5.868000278715044, 5.872000278905034, 5.876000279095024, 5.880000279285014, 5.8840002794750035, 5.888000279664993, 5.892000279854983, 5.896000280044973, 5.900000280234963, 5.9040002804249525, 5.908000280614942, 5.912000280804932, 5.916000280994922, 5.920000281184912, 5.9240002813749015, 5.928000281564891, 5.932000281754881, 5.936000281944871, 5.940000282134861, 5.944000282324851, 5.94800028251484, 5.95200028270483, 5.95600028289482, 5.96000028308481, 5.9640002832748, 5.968000283464789, 5.972000283654779, 5.976000283844769, 5.980000284034759, 5.984000284224749, 5.988000284414738, 5.992000284604728, 5.996000284794718, 6.000000284984708, 6.004000285174698, 6.008000285364687, 6.012000285554677, 6.016000285744667, 6.020000285934657, 6.024000286124647, 6.0280002863146365, 6.032000286504626, 6.036000286694616, 6.040000286884606, 6.044000287074596, 6.0480002872645855, 6.052000287454575, 6.056000287644565, 6.060000287834555, 6.064000288024545, 6.0680002882145345, 6.072000288404524, 6.076000288594514, 6.080000288784504, 6.084000288974494, 6.0880002891644835, 6.092000289354473, 6.096000289544463, 6.100000289734453, 6.104000289924443, 6.108000290114433, 6.112000290304422, 6.116000290494412, 6.120000290684402, 6.124000290874392, 6.128000291064382, 6.132000291254371, 6.136000291444361, 6.140000291634351, 6.144000291824341, 6.148000292014331, 6.15200029220432, 6.15600029239431, 6.1600002925843, 6.16400029277429, 6.16800029296428, 6.1720002931542695, 6.176000293344259, 6.180000293534249, 6.184000293724239, 6.188000293914229, 6.1920002941042185, 6.196000294294208, 6.200000294484198, 6.204000294674188, 6.208000294864178, 6.2120002950541675, 6.216000295244157, 6.220000295434147, 6.224000295624137, 6.228000295814127, 6.2320002960041165, 6.236000296194106, 6.240000296384096, 6.244000296574086, 6.248000296764076, 6.252000296954066, 6.256000297144055, 6.260000297334045, 6.264000297524035, 6.268000297714025, 6.272000297904015, 6.276000298094004, 6.280000298283994, 6.284000298473984, 6.288000298663974, 6.292000298853964, 6.296000299043953, 6.300000299233943, 6.304000299423933, 6.308000299613923, 6.312000299803913, 6.3160002999939024, 6.320000300183892, 6.324000300373882, 6.328000300563872, 6.332000300753862, 6.3360003009438515, 6.340000301133841, 6.344000301323831, 6.348000301513821, 6.352000301703811, 6.3560003018938005, 6.36000030208379, 6.36400030227378, 6.36800030246377, 6.37200030265376, 6.3760003028437495, 6.380000303033739, 6.384000303223729, 6.388000303413719, 6.392000303603709, 6.3960003037936985, 6.400000303983688, 6.404000304173678, 6.408000304363668, 6.412000304553658, 6.416000304743648, 6.420000304933637, 6.424000305123627, 6.428000305313617, 6.432000305503607, 6.436000305693597, 6.440000305883586, 6.444000306073576, 6.448000306263566, 6.452000306453556, 6.456000306643546, 6.460000306833535, 6.464000307023525, 6.468000307213515, 6.472000307403505, 6.476000307593495, 6.4800003077834845, 6.484000307973474, 6.488000308163464, 6.492000308353454, 6.496000308543444, 6.5000003087334335, 6.504000308923423, 6.508000309113413, 6.512000309303403, 6.516000309493393, 6.5200003096833825, 6.524000309873372, 6.528000310063362, 6.532000310253352, 6.536000310443342, 6.5400003106333315, 6.544000310823321, 6.548000311013311, 6.552000311203301, 6.556000311393291, 6.560000311583281, 6.56400031177327, 6.56800031196326, 6.57200031215325, 6.57600031234324, 6.58000031253323, 6.584000312723219, 6.588000312913209, 6.592000313103199, 6.596000313293189, 6.600000313483179, 6.604000313673168, 6.608000313863158, 6.612000314053148, 6.616000314243138, 6.620000314433128, 6.6240003146231174, 6.628000314813107, 6.632000315003097, 6.636000315193087, 6.640000315383077, 6.6440003155730665, 6.648000315763056, 6.652000315953046, 6.656000316143036, 6.660000316333026, 6.6640003165230155, 6.668000316713005, 6.672000316902995, 6.676000317092985, 6.680000317282975, 6.6840003174729645, 6.688000317662954, 6.692000317852944, 6.696000318042934, 6.700000318232924, 6.7040003184229136, 6.708000318612903, 6.712000318802893, 6.716000318992883, 6.720000319182873, 6.724000319372863, 6.728000319562852, 6.732000319752842, 6.736000319942832, 6.740000320132822, 6.744000320322812, 6.748000320512801, 6.752000320702791, 6.756000320892781, 6.760000321082771, 6.764000321272761, 6.76800032146275, 6.77200032165274, 6.77600032184273, 6.78000032203272, 6.78400032222271, 6.7880003224126995, 6.792000322602689, 6.796000322792679, 6.800000322982669, 6.804000323172659, 6.8080003233626485, 6.812000323552638, 6.816000323742628, 6.820000323932618, 6.824000324122608, 6.8280003243125975, 6.832000324502587, 6.836000324692577, 6.840000324882567, 6.844000325072557, 6.8480003252625465, 6.852000325452536, 6.856000325642526, 6.860000325832516, 6.864000326022506, 6.868000326212496, 6.872000326402485, 6.876000326592475, 6.880000326782465, 6.884000326972455, 6.888000327162445, 6.892000327352434, 6.896000327542424, 6.900000327732414, 6.904000327922404, 6.908000328112394, 6.912000328302383, 6.916000328492373, 6.920000328682363, 6.924000328872353, 6.928000329062343, 6.9320003292523324, 6.936000329442322, 6.940000329632312, 6.944000329822302, 6.948000330012292, 6.9520003302022815, 6.956000330392271, 6.960000330582261, 6.964000330772251, 6.968000330962241, 6.9720003311522305, 6.97600033134222, 6.98000033153221, 6.9840003317222, 6.98800033191219, 6.9920003321021795, 6.996000332292169, 7.000000332482159, 7.004000332672149, 7.008000332862139, 7.0120003330521286, 7.016000333242118, 7.020000333432108, 7.024000333622098, 7.028000333812088, 7.032000334002078, 7.036000334192067, 7.040000334382057, 7.044000334572047, 7.048000334762037, 7.052000334952027, 7.056000335142016, 7.060000335332006, 7.064000335521996, 7.068000335711986, 7.072000335901976, 7.076000336091965, 7.080000336281955, 7.084000336471945, 7.088000336661935, 7.092000336851925, 7.0960003370419145, 7.100000337231904, 7.104000337421894, 7.108000337611884, 7.112000337801874, 7.1160003379918635, 7.120000338181853, 7.124000338371843, 7.128000338561833, 7.132000338751823, 7.1360003389418125, 7.140000339131802, 7.144000339321792, 7.148000339511782, 7.152000339701772, 7.1560003398917615, 7.160000340081751, 7.164000340271741, 7.168000340461731, 7.172000340651721, 7.176000340841711, 7.1800003410317, 7.18400034122169, 7.18800034141168, 7.19200034160167, 7.19600034179166, 7.200000341981649, 7.204000342171639, 7.208000342361629, 7.212000342551619, 7.216000342741609, 7.220000342931598, 7.224000343121588, 7.228000343311578, 7.232000343501568, 7.236000343691558, 7.2400003438815475, 7.244000344071537, 7.248000344261527, 7.252000344451517, 7.256000344641507, 7.2600003448314965, 7.264000345021486, 7.268000345211476, 7.272000345401466, 7.276000345591456, 7.2800003457814455, 7.284000345971435, 7.288000346161425, 7.292000346351415, 7.296000346541405, 7.3000003467313945, 7.304000346921384, 7.308000347111374, 7.312000347301364, 7.316000347491354, 7.3200003476813436, 7.324000347871333, 7.328000348061323, 7.332000348251313, 7.336000348441303, 7.340000348631293, 7.344000348821282, 7.348000349011272, 7.352000349201262, 7.356000349391252, 7.360000349581242, 7.364000349771231, 7.368000349961221, 7.372000350151211, 7.376000350341201, 7.380000350531191, 7.38400035072118, 7.38800035091117, 7.39200035110116, 7.39600035129115, 7.40000035148114, 7.4040003516711295, 7.408000351861119, 7.412000352051109, 7.416000352241099, 7.420000352431089, 7.4240003526210785, 7.428000352811068, 7.432000353001058, 7.436000353191048, 7.440000353381038, 7.4440003535710275, 7.448000353761017, 7.452000353951007, 7.456000354140997, 7.460000354330987, 7.4640003545209765, 7.468000354710966, 7.472000354900956, 7.476000355090946, 7.480000355280936, 7.484000355470926, 7.488000355660915, 7.492000355850905, 7.496000356040895, 7.500000356230885, 7.504000356420875, 7.508000356610864, 7.512000356800854, 7.516000356990844, 7.520000357180834, 7.524000357370824, 7.528000357560813, 7.532000357750803, 7.536000357940793, 7.540000358130783, 7.544000358320773, 7.5480003585107625, 7.552000358700752, 7.556000358890742, 7.560000359080732, 7.564000359270722, 7.5680003594607115, 7.572000359650701, 7.576000359840691, 7.580000360030681, 7.584000360220671, 7.5880003604106605, 7.59200036060065, 7.59600036079064, 7.60000036098063, 7.60400036117062, 7.6080003613606095, 7.612000361550599, 7.616000361740589, 7.620000361930579, 7.624000362120569, 7.628000362310559, 7.632000362500548, 7.636000362690538, 7.640000362880528, 7.644000363070518, 7.648000363260508, 7.652000363450497, 7.656000363640487, 7.660000363830477, 7.664000364020467, 7.668000364210457, 7.672000364400446, 7.676000364590436, 7.680000364780426, 7.684000364970416, 7.688000365160406, 7.692000365350395, 7.696000365540385, 7.700000365730375, 7.704000365920365, 7.708000366110355, 7.7120003663003445, 7.716000366490334, 7.720000366680324, 7.724000366870314, 7.728000367060304, 7.7320003672502935, 7.736000367440283, 7.740000367630273, 7.744000367820263, 7.748000368010253, 7.7520003682002425, 7.756000368390232, 7.760000368580222, 7.764000368770212, 7.768000368960202, 7.7720003691501915, 7.776000369340181, 7.780000369530171, 7.784000369720161, 7.788000369910151, 7.792000370100141, 7.79600037029013, 7.80000037048012, 7.80400037067011, 7.8080003708601, 7.81200037105009, 7.816000371240079, 7.820000371430069, 7.824000371620059, 7.828000371810049, 7.832000372000039, 7.836000372190028, 7.840000372380018, 7.844000372570008, 7.848000372759998, 7.852000372949988, 7.8560003731399775, 7.860000373329967, 7.864000373519957, 7.868000373709947, 7.872000373899937, 7.8760003740899265, 7.880000374279916, 7.884000374469906, 7.888000374659896, 7.892000374849886, 7.8960003750398755, 7.900000375229865, 7.904000375419855, 7.908000375609845, 7.912000375799835, 7.9160003759898245, 7.920000376179814, 7.924000376369804, 7.928000376559794, 7.932000376749784, 7.936000376939774, 7.940000377129763, 7.944000377319753, 7.948000377509743, 7.952000377699733, 7.956000377889723, 7.960000378079712, 7.964000378269702, 7.968000378459692, 7.972000378649682, 7.976000378839672, 7.980000379029661, 7.984000379219651, 7.988000379409641, 7.992000379599631, 7.996000379789621, 8.00000037997961, 8.0040003801696, 8.00800038035959, 8.01200038054958, 8.01600038073957, 8.02000038092956, 8.02400038111955, 8.028000381309539, 8.032000381499529, 8.036000381689519, 8.040000381879508, 8.044000382069498, 8.048000382259488, 8.052000382449478, 8.056000382639468, 8.060000382829458, 8.064000383019447, 8.068000383209437, 8.072000383399427, 8.076000383589417, 8.080000383779407, 8.084000383969396, 8.088000384159386, 8.092000384349376, 8.096000384539366, 8.100000384729356, 8.104000384919345, 8.108000385109335, 8.112000385299325, 8.116000385489315, 8.120000385679305, 8.124000385869294, 8.128000386059284, 8.132000386249274, 8.136000386439264, 8.140000386629254, 8.144000386819243, 8.148000387009233, 8.152000387199223, 8.156000387389213, 8.160000387579203, 8.164000387769192, 8.168000387959182, 8.172000388149172, 8.176000388339162, 8.180000388529152, 8.184000388719141, 8.188000388909131, 8.192000389099121, 8.196000389289111, 8.2000003894791, 8.20400038966909, 8.20800038985908, 8.21200039004907, 8.21600039023906, 8.22000039042905, 8.22400039061904, 8.22800039080903, 8.23200039099902, 8.236000391189009, 8.240000391378999, 8.244000391568989, 8.248000391758978, 8.252000391948968, 8.256000392138958, 8.260000392328948, 8.264000392518938, 8.268000392708927, 8.272000392898917, 8.276000393088907, 8.280000393278897, 8.284000393468887, 8.288000393658876, 8.292000393848866, 8.296000394038856, 8.300000394228846, 8.304000394418836, 8.308000394608825, 8.312000394798815, 8.316000394988805, 8.320000395178795, 8.324000395368785, 8.328000395558774, 8.332000395748764, 8.336000395938754, 8.340000396128744, 8.344000396318734, 8.348000396508723, 8.352000396698713, 8.356000396888703, 8.360000397078693, 8.364000397268683, 8.368000397458673, 8.372000397648662, 8.376000397838652, 8.380000398028642, 8.384000398218632, 8.388000398408622, 8.392000398598611, 8.396000398788601, 8.400000398978591, 8.40400039916858, 8.40800039935857, 8.41200039954856, 8.41600039973855, 8.42000039992854, 8.42400040011853, 8.42800040030852, 8.43200040049851, 8.4360004006885, 8.440000400878489, 8.444000401068479, 8.448000401258469, 8.452000401448458, 8.456000401638448, 8.460000401828438, 8.464000402018428, 8.468000402208418, 8.472000402398407, 8.476000402588397, 8.480000402778387, 8.484000402968377, 8.488000403158367, 8.492000403348356, 8.496000403538346, 8.500000403728336, 8.504000403918326, 8.508000404108316, 8.512000404298306, 8.516000404488295, 8.520000404678285, 8.524000404868275, 8.528000405058265, 8.532000405248255, 8.536000405438244, 8.540000405628234, 8.544000405818224, 8.548000406008214, 8.552000406198204, 8.556000406388193, 8.560000406578183, 8.564000406768173, 8.568000406958163, 8.572000407148153, 8.576000407338142, 8.580000407528132, 8.584000407718122, 8.588000407908112, 8.592000408098102, 8.596000408288091, 8.600000408478081, 8.604000408668071, 8.60800040885806, 8.61200040904805, 8.61600040923804, 8.62000040942803, 8.62400040961802, 8.62800040980801, 8.632000409998, 8.63600041018799, 8.64000041037798, 8.644000410567969, 8.648000410757959, 8.652000410947949, 8.656000411137938, 8.660000411327928, 8.664000411517918, 8.668000411707908, 8.672000411897898, 8.676000412087888, 8.680000412277877, 8.684000412467867, 8.688000412657857, 8.692000412847847, 8.696000413037837, 8.700000413227826, 8.704000413417816, 8.708000413607806, 8.712000413797796, 8.716000413987786, 8.720000414177775, 8.724000414367765, 8.728000414557755, 8.732000414747745, 8.736000414937735, 8.740000415127724, 8.744000415317714, 8.748000415507704, 8.752000415697694, 8.756000415887684, 8.760000416077673, 8.764000416267663, 8.768000416457653, 8.772000416647643, 8.776000416837633, 8.780000417027622, 8.784000417217612, 8.788000417407602, 8.792000417597592, 8.796000417787582, 8.800000417977571, 8.804000418167561, 8.808000418357551, 8.812000418547541, 8.81600041873753, 8.82000041892752, 8.82400041911751, 8.8280004193075, 8.83200041949749, 8.83600041968748, 8.84000041987747, 8.84400042006746, 8.84800042025745, 8.852000420447439, 8.856000420637429, 8.860000420827419, 8.864000421017408, 8.868000421207398, 8.872000421397388, 8.876000421587378, 8.880000421777368, 8.884000421967357, 8.888000422157347, 8.892000422347337, 8.896000422537327, 8.900000422727317, 8.904000422917306, 8.908000423107296, 8.912000423297286, 8.916000423487276, 8.920000423677266, 8.924000423867255, 8.928000424057245, 8.932000424247235, 8.936000424437225, 8.940000424627215, 8.944000424817204, 8.948000425007194, 8.952000425197184, 8.956000425387174, 8.960000425577164, 8.964000425767154, 8.968000425957143, 8.972000426147133, 8.976000426337123, 8.980000426527113, 8.984000426717103, 8.988000426907092, 8.992000427097082, 8.996000427287072, 9.000000427477062, 9.004000427667052, 9.008000427857041, 9.012000428047031, 9.016000428237021, 9.02000042842701, 9.024000428617, 9.02800042880699, 9.03200042899698, 9.03600042918697, 9.04000042937696, 9.04400042956695, 9.04800042975694, 9.05200042994693, 9.056000430136919, 9.060000430326909, 9.064000430516899, 9.068000430706888, 9.072000430896878, 9.076000431086868, 9.080000431276858, 9.084000431466848, 9.088000431656837, 9.092000431846827, 9.096000432036817, 9.100000432226807, 9.104000432416797, 9.108000432606786, 9.112000432796776, 9.116000432986766, 9.120000433176756, 9.124000433366746, 9.128000433556736, 9.132000433746725, 9.136000433936715, 9.140000434126705, 9.144000434316695, 9.148000434506685, 9.152000434696674, 9.156000434886664, 9.160000435076654, 9.164000435266644, 9.168000435456634, 9.172000435646623, 9.176000435836613, 9.180000436026603, 9.184000436216593, 9.188000436406583, 9.192000436596572, 9.196000436786562, 9.200000436976552, 9.204000437166542, 9.208000437356532, 9.212000437546521, 9.216000437736511, 9.220000437926501, 9.22400043811649, 9.22800043830648, 9.23200043849647, 9.23600043868646, 9.24000043887645, 9.24400043906644, 9.24800043925643, 9.25200043944642, 9.25600043963641, 9.260000439826399, 9.264000440016389, 9.268000440206379, 9.272000440396369, 9.276000440586358, 9.280000440776348, 9.284000440966338, 9.288000441156328, 9.292000441346318, 9.296000441536307, 9.300000441726297, 9.304000441916287, 9.308000442106277, 9.312000442296267, 9.316000442486256, 9.320000442676246, 9.324000442866236, 9.328000443056226, 9.332000443246216, 9.336000443436205, 9.340000443626195, 9.344000443816185, 9.348000444006175, 9.352000444196165, 9.356000444386154, 9.360000444576144, 9.364000444766134, 9.368000444956124, 9.372000445146114, 9.376000445336103, 9.380000445526093, 9.384000445716083, 9.388000445906073, 9.392000446096063, 9.396000446286052, 9.400000446476042, 9.404000446666032, 9.408000446856022, 9.412000447046012, 9.416000447236001, 9.420000447425991, 9.424000447615981, 9.428000447805971, 9.43200044799596, 9.43600044818595, 9.44000044837594, 9.44400044856593, 9.44800044875592, 9.45200044894591, 9.4560004491359, 9.46000044932589, 9.46400044951588, 9.468000449705869, 9.472000449895859, 9.476000450085849, 9.480000450275838, 9.484000450465828, 9.488000450655818, 9.492000450845808, 9.496000451035798, 9.500000451225787, 9.504000451415777, 9.508000451605767, 9.512000451795757, 9.516000451985747, 9.520000452175736, 9.524000452365726, 9.528000452555716, 9.532000452745706, 9.536000452935696, 9.540000453125685, 9.544000453315675, 9.548000453505665, 9.552000453695655, 9.556000453885645, 9.560000454075634, 9.564000454265624, 9.568000454455614, 9.572000454645604, 9.576000454835594, 9.580000455025584, 9.584000455215573, 9.588000455405563, 9.592000455595553, 9.596000455785543, 9.600000455975533, 9.604000456165522, 9.608000456355512, 9.612000456545502, 9.616000456735492, 9.620000456925482, 9.624000457115471, 9.628000457305461, 9.632000457495451, 9.63600045768544, 9.64000045787543, 9.64400045806542, 9.64800045825541, 9.6520004584454, 9.65600045863539, 9.66000045882538, 9.66400045901537, 9.66800045920536, 9.672000459395349, 9.676000459585339, 9.680000459775329, 9.684000459965318, 9.688000460155308, 9.692000460345298, 9.696000460535288, 9.700000460725278, 9.704000460915267, 9.708000461105257, 9.712000461295247, 9.716000461485237, 9.720000461675227, 9.724000461865216, 9.728000462055206, 9.732000462245196, 9.736000462435186, 9.740000462625176, 9.744000462815166, 9.748000463005155, 9.752000463195145, 9.756000463385135, 9.760000463575125, 9.764000463765115, 9.768000463955104, 9.772000464145094, 9.776000464335084, 9.780000464525074, 9.784000464715064, 9.788000464905053, 9.792000465095043, 9.796000465285033, 9.800000465475023, 9.804000465665013, 9.808000465855002, 9.812000466044992, 9.816000466234982, 9.820000466424972, 9.824000466614962, 9.828000466804951, 9.832000466994941, 9.836000467184931, 9.84000046737492, 9.84400046756491, 9.8480004677549, 9.85200046794489, 9.85600046813488, 9.86000046832487, 9.86400046851486, 9.86800046870485, 9.87200046889484, 9.876000469084829, 9.880000469274819, 9.884000469464809, 9.888000469654799, 9.892000469844788, 9.896000470034778, 9.900000470224768, 9.904000470414758, 9.908000470604748, 9.912000470794737, 9.916000470984727, 9.920000471174717, 9.924000471364707, 9.928000471554697, 9.932000471744686, 9.936000471934676, 9.940000472124666, 9.944000472314656, 9.948000472504646, 9.952000472694635, 9.956000472884625, 9.960000473074615, 9.964000473264605, 9.968000473454595, 9.972000473644584, 9.976000473834574, 9.980000474024564, 9.984000474214554, 9.988000474404544, 9.992000474594533, 9.996000474784523, 10.000000474974513, 10.004000475164503, 10.008000475354493, 10.012000475544482, 10.016000475734472, 10.020000475924462, 10.024000476114452, 10.028000476304442, 10.032000476494431, 10.036000476684421, 10.040000476874411, 10.044000477064401, 10.04800047725439, 10.05200047744438, 10.05600047763437, 10.06000047782436, 10.06400047801435, 10.06800047820434, 10.07200047839433, 10.07600047858432, 10.08000047877431, 10.084000478964299, 10.088000479154289, 10.092000479344279, 10.096000479534268, 10.100000479724258, 10.104000479914248, 10.108000480104238, 10.112000480294228, 10.116000480484217, 10.120000480674207, 10.124000480864197, 10.128000481054187, 10.132000481244177, 10.136000481434166, 10.140000481624156, 10.144000481814146, 10.148000482004136, 10.152000482194126, 10.156000482384115, 10.160000482574105, 10.164000482764095, 10.168000482954085, 10.172000483144075, 10.176000483334064, 10.180000483524054, 10.184000483714044, 10.188000483904034, 10.192000484094024, 10.196000484284014, 10.200000484474003, 10.204000484663993, 10.208000484853983, 10.212000485043973, 10.216000485233963, 10.220000485423952, 10.224000485613942, 10.228000485803932, 10.232000485993922, 10.236000486183912, 10.240000486373901, 10.244000486563891, 10.248000486753881, 10.25200048694387, 10.25600048713386, 10.26000048732385, 10.26400048751384, 10.26800048770383, 10.27200048789382, 10.27600048808381, 10.2800004882738, 10.28400048846379, 10.288000488653779, 10.292000488843769, 10.296000489033759, 10.300000489223748, 10.304000489413738, 10.308000489603728, 10.312000489793718, 10.316000489983708, 10.320000490173697, 10.324000490363687, 10.328000490553677, 10.332000490743667, 10.336000490933657, 10.340000491123646, 10.344000491313636, 10.348000491503626, 10.352000491693616, 10.356000491883606, 10.360000492073596, 10.364000492263585, 10.368000492453575, 10.372000492643565, 10.376000492833555, 10.380000493023545, 10.384000493213534, 10.388000493403524, 10.392000493593514, 10.396000493783504, 10.400000493973494, 10.404000494163483, 10.408000494353473, 10.412000494543463, 10.416000494733453, 10.420000494923443, 10.424000495113432, 10.428000495303422, 10.432000495493412, 10.436000495683402, 10.440000495873392, 10.444000496063381, 10.448000496253371, 10.452000496443361, 10.45600049663335, 10.46000049682334, 10.46400049701333, 10.46800049720332, 10.47200049739331, 10.4760004975833, 10.48000049777329, 10.48400049796328, 10.48800049815327, 10.492000498343259, 10.496000498533249, 10.500000498723239, 10.504000498913229, 10.508000499103218, 10.512000499293208, 10.516000499483198, 10.520000499673188, 10.524000499863178, 10.528000500053167, 10.532000500243157, 10.536000500433147, 10.540000500623137, 10.544000500813127, 10.548000501003116, 10.552000501193106, 10.556000501383096, 10.560000501573086, 10.564000501763076, 10.568000501953065, 10.572000502143055, 10.576000502333045, 10.580000502523035, 10.584000502713025, 10.588000502903014, 10.592000503093004, 10.596000503282994, 10.600000503472984, 10.604000503662974, 10.608000503852963, 10.612000504042953, 10.616000504232943, 10.620000504422933, 10.624000504612923, 10.628000504802912, 10.632000504992902, 10.636000505182892, 10.640000505372882, 10.644000505562872, 10.648000505752861, 10.652000505942851, 10.656000506132841, 10.660000506322831, 10.66400050651282, 10.66800050670281, 10.6720005068928, 10.67600050708279, 10.68000050727278, 10.68400050746277, 10.68800050765276, 10.69200050784275, 10.69600050803274, 10.700000508222729, 10.704000508412719, 10.708000508602709, 10.712000508792698, 10.716000508982688, 10.720000509172678, 10.724000509362668, 10.728000509552658, 10.732000509742647, 10.736000509932637, 10.740000510122627, 10.744000510312617, 10.748000510502607, 10.752000510692596, 10.756000510882586, 10.760000511072576, 10.764000511262566, 10.768000511452556, 10.772000511642545, 10.776000511832535, 10.780000512022525, 10.784000512212515, 10.788000512402505, 10.792000512592494, 10.796000512782484, 10.800000512972474, 10.804000513162464, 10.808000513352454, 10.812000513542444, 10.816000513732433, 10.820000513922423, 10.824000514112413, 10.828000514302403, 10.832000514492393, 10.836000514682382, 10.840000514872372, 10.844000515062362, 10.848000515252352, 10.852000515442342, 10.856000515632331, 10.860000515822321, 10.864000516012311, 10.8680005162023, 10.87200051639229, 10.87600051658228, 10.88000051677227, 10.88400051696226, 10.88800051715225, 10.89200051734224, 10.89600051753223, 10.90000051772222, 10.904000517912209, 10.908000518102199, 10.912000518292189, 10.916000518482178, 10.920000518672168, 10.924000518862158, 10.928000519052148, 10.932000519242138, 10.936000519432127, 10.940000519622117, 10.944000519812107, 10.948000520002097, 10.952000520192087, 10.956000520382077, 10.960000520572066, 10.964000520762056, 10.968000520952046, 10.972000521142036, 10.976000521332026, 10.980000521522015, 10.984000521712005, 10.988000521901995, 10.992000522091985, 10.996000522281975, 11.000000522471964, 11.004000522661954, 11.008000522851944, 11.012000523041934, 11.016000523231924, 11.020000523421913, 11.024000523611903, 11.028000523801893, 11.032000523991883, 11.036000524181873, 11.040000524371862, 11.044000524561852, 11.048000524751842, 11.052000524941832, 11.056000525131822, 11.060000525321811, 11.064000525511801, 11.068000525701791, 11.07200052589178, 11.07600052608177, 11.08000052627176, 11.08400052646175, 11.08800052665174, 11.09200052684173, 11.09600052703172, 11.10000052722171, 11.1040005274117, 11.108000527601689, 11.112000527791679, 11.116000527981669, 11.120000528171659, 11.124000528361648, 11.128000528551638, 11.132000528741628, 11.136000528931618, 11.140000529121608, 11.144000529311597, 11.148000529501587, 11.152000529691577, 11.156000529881567, 11.160000530071557, 11.164000530261546, 11.168000530451536, 11.172000530641526, 11.176000530831516, 11.180000531021506, 11.184000531211495, 11.188000531401485, 11.192000531591475, 11.196000531781465, 11.200000531971455, 11.204000532161444, 11.208000532351434, 11.212000532541424, 11.216000532731414, 11.220000532921404, 11.224000533111393, 11.228000533301383, 11.232000533491373, 11.236000533681363, 11.240000533871353, 11.244000534061342, 11.248000534251332, 11.252000534441322, 11.256000534631312, 11.260000534821302, 11.264000535011292, 11.268000535201281, 11.272000535391271, 11.276000535581261, 11.28000053577125, 11.28400053596124, 11.28800053615123, 11.29200053634122, 11.29600053653121, 11.3000005367212, 11.30400053691119, 11.30800053710118, 11.31200053729117, 11.316000537481159, 11.320000537671149, 11.324000537861139, 11.328000538051128, 11.332000538241118, 11.336000538431108, 11.340000538621098, 11.344000538811088, 11.348000539001077, 11.352000539191067, 11.356000539381057, 11.360000539571047, 11.364000539761037, 11.368000539951026, 11.372000540141016, 11.376000540331006, 11.380000540520996, 11.384000540710986, 11.388000540900975, 11.392000541090965, 11.396000541280955, 11.400000541470945, 11.404000541660935, 11.408000541850924, 11.412000542040914, 11.416000542230904, 11.420000542420894, 11.424000542610884, 11.428000542800874, 11.432000542990863, 11.436000543180853, 11.440000543370843, 11.444000543560833, 11.448000543750823, 11.452000543940812, 11.456000544130802, 11.460000544320792, 11.464000544510782, 11.468000544700772, 11.472000544890761, 11.476000545080751, 11.480000545270741, 11.48400054546073, 11.48800054565072, 11.49200054584071, 11.4960005460307, 11.50000054622069, 11.50400054641068, 11.50800054660067, 11.51200054679066, 11.51600054698065, 11.520000547170639, 11.524000547360629, 11.528000547550619, 11.532000547740608, 11.536000547930598, 11.540000548120588, 11.544000548310578, 11.548000548500568, 11.552000548690557, 11.556000548880547, 11.560000549070537, 11.564000549260527, 11.568000549450517, 11.572000549640507, 11.576000549830496, 11.580000550020486, 11.584000550210476, 11.588000550400466, 11.592000550590456, 11.596000550780445, 11.600000550970435, 11.604000551160425, 11.608000551350415, 11.612000551540405, 11.616000551730394, 11.620000551920384, 11.624000552110374, 11.628000552300364, 11.632000552490354, 11.636000552680343, 11.640000552870333, 11.644000553060323, 11.648000553250313, 11.652000553440303, 11.656000553630292, 11.660000553820282, 11.664000554010272, 11.668000554200262, 11.672000554390252, 11.676000554580241, 11.680000554770231, 11.684000554960221, 11.68800055515021, 11.6920005553402, 11.69600055553019, 11.70000055572018, 11.70400055591017, 11.70800055610016, 11.71200055629015, 11.71600055648014, 11.72000055667013, 11.724000556860119, 11.728000557050109, 11.732000557240099, 11.736000557430089, 11.740000557620078, 11.744000557810068, 11.748000558000058, 11.752000558190048, 11.756000558380038, 11.760000558570027, 11.764000558760017, 11.768000558950007, 11.772000559139997, 11.776000559329987, 11.780000559519976, 11.784000559709966, 11.788000559899956, 11.792000560089946, 11.796000560279936, 11.800000560469925, 11.804000560659915, 11.808000560849905, 11.812000561039895, 11.816000561229885, 11.820000561419874, 11.824000561609864, 11.828000561799854, 11.832000561989844, 11.836000562179834, 11.840000562369823, 11.844000562559813, 11.848000562749803, 11.852000562939793, 11.856000563129783, 11.860000563319772, 11.864000563509762, 11.868000563699752, 11.872000563889742, 11.876000564079732, 11.880000564269722, 11.884000564459711, 11.888000564649701, 11.892000564839691, 11.89600056502968, 11.90000056521967, 11.90400056540966, 11.90800056559965, 11.91200056578964, 11.91600056597963, 11.92000056616962, 11.92400056635961, 11.9280005665496, 11.932000566739589, 11.936000566929579, 11.940000567119569, 11.944000567309558, 11.948000567499548, 11.952000567689538, 11.956000567879528, 11.960000568069518, 11.964000568259507, 11.968000568449497, 11.972000568639487, 11.976000568829477, 11.980000569019467, 11.984000569209456, 11.988000569399446, 11.992000569589436, 11.996000569779426, 12.000000569969416, 12.004000570159405, 12.008000570349395, 12.012000570539385, 12.016000570729375, 12.020000570919365, 12.024000571109354, 12.028000571299344, 12.032000571489334, 12.036000571679324, 12.040000571869314, 12.044000572059304, 12.048000572249293, 12.052000572439283, 12.056000572629273, 12.060000572819263, 12.064000573009253, 12.068000573199242, 12.072000573389232, 12.076000573579222, 12.080000573769212, 12.084000573959202, 12.088000574149191, 12.092000574339181, 12.096000574529171, 12.10000057471916, 12.10400057490915, 12.10800057509914, 12.11200057528913, 12.11600057547912, 12.12000057566911, 12.1240005758591, 12.12800057604909, 12.13200057623908, 12.136000576429069, 12.140000576619059, 12.144000576809049, 12.148000576999038, 12.152000577189028, 12.156000577379018, 12.160000577569008, 12.164000577758998, 12.168000577948987, 12.172000578138977, 12.176000578328967, 12.180000578518957, 12.184000578708947, 12.188000578898937, 12.192000579088926, 12.196000579278916, 12.200000579468906, 12.204000579658896, 12.208000579848886, 12.212000580038875, 12.216000580228865, 12.220000580418855, 12.224000580608845, 12.228000580798835, 12.232000580988824, 12.236000581178814, 12.240000581368804, 12.244000581558794, 12.248000581748784, 12.252000581938773, 12.256000582128763, 12.260000582318753, 12.264000582508743, 12.268000582698733, 12.272000582888722, 12.276000583078712, 12.280000583268702, 12.284000583458692, 12.288000583648682, 12.292000583838671, 12.296000584028661, 12.300000584218651, 12.30400058440864, 12.30800058459863, 12.31200058478862, 12.31600058497861, 12.3200005851686, 12.32400058535859, 12.32800058554858, 12.33200058573857, 12.33600058592856, 12.340000586118549, 12.344000586308539, 12.348000586498529, 12.352000586688519, 12.356000586878508, 12.360000587068498, 12.364000587258488, 12.368000587448478, 12.372000587638468, 12.376000587828457, 12.380000588018447, 12.384000588208437, 12.388000588398427, 12.392000588588417, 12.396000588778406, 12.400000588968396, 12.404000589158386, 12.408000589348376, 12.412000589538366, 12.416000589728355, 12.420000589918345, 12.424000590108335, 12.428000590298325, 12.432000590488315, 12.436000590678304, 12.440000590868294, 12.444000591058284, 12.448000591248274, 12.452000591438264, 12.456000591628253, 12.460000591818243, 12.464000592008233, 12.468000592198223, 12.472000592388213, 12.476000592578202, 12.480000592768192, 12.484000592958182, 12.488000593148172, 12.492000593338162, 12.496000593528152, 12.500000593718141, 12.504000593908131, 12.508000594098121, 12.51200059428811, 12.5160005944781, 12.52000059466809, 12.52400059485808, 12.52800059504807, 12.53200059523806, 12.53600059542805, 12.54000059561804, 12.54400059580803, 12.548000595998019, 12.552000596188009, 12.556000596377999, 12.560000596567988, 12.564000596757978, 12.568000596947968, 12.572000597137958, 12.576000597327948, 12.580000597517937, 12.584000597707927, 12.588000597897917, 12.592000598087907, 12.596000598277897, 12.600000598467886, 12.604000598657876, 12.608000598847866, 12.612000599037856, 12.616000599227846, 12.620000599417835, 12.624000599607825, 12.628000599797815, 12.632000599987805, 12.636000600177795, 12.640000600367785, 12.644000600557774, 12.648000600747764, 12.652000600937754, 12.656000601127744, 12.660000601317734, 12.664000601507723, 12.668000601697713, 12.672000601887703, 12.676000602077693, 12.680000602267683, 12.684000602457672, 12.688000602647662, 12.692000602837652, 12.696000603027642, 12.700000603217632, 12.704000603407621, 12.708000603597611, 12.712000603787601, 12.71600060397759, 12.72000060416758, 12.72400060435757, 12.72800060454756, 12.73200060473755, 12.73600060492754, 12.74000060511753, 12.74400060530752, 12.74800060549751, 12.752000605687499, 12.756000605877489, 12.760000606067479, 12.764000606257468, 12.768000606447458, 12.772000606637448, 12.776000606827438, 12.780000607017428, 12.784000607207417, 12.788000607397407, 12.792000607587397, 12.796000607777387, 12.800000607967377, 12.804000608157367, 12.808000608347356, 12.812000608537346, 12.816000608727336, 12.820000608917326, 12.824000609107316, 12.828000609297305, 12.832000609487295, 12.836000609677285, 12.840000609867275, 12.844000610057265, 12.848000610247254, 12.852000610437244, 12.856000610627234, 12.860000610817224, 12.864000611007214, 12.868000611197203, 12.872000611387193, 12.876000611577183, 12.880000611767173, 12.884000611957163, 12.888000612147152, 12.892000612337142, 12.896000612527132, 12.900000612717122, 12.904000612907112, 12.908000613097101, 12.912000613287091, 12.916000613477081, 12.92000061366707, 12.92400061385706, 12.92800061404705, 12.93200061423704, 12.93600061442703, 12.94000061461702, 12.94400061480701, 12.948000614997, 12.95200061518699, 12.95600061537698, 12.960000615566969, 12.964000615756959, 12.968000615946949, 12.972000616136938, 12.976000616326928, 12.980000616516918, 12.984000616706908, 12.988000616896898, 12.992000617086887, 12.996000617276877, 13.000000617466867, 13.004000617656857, 13.008000617846847, 13.012000618036836, 13.016000618226826, 13.020000618416816, 13.024000618606806, 13.028000618796796, 13.032000618986785, 13.036000619176775, 13.040000619366765, 13.044000619556755, 13.048000619746745, 13.052000619936734, 13.056000620126724, 13.060000620316714, 13.064000620506704, 13.068000620696694, 13.072000620886683, 13.076000621076673, 13.080000621266663, 13.084000621456653, 13.088000621646643, 13.092000621836632, 13.096000622026622, 13.100000622216612, 13.104000622406602, 13.108000622596592, 13.112000622786582, 13.116000622976571, 13.120000623166561, 13.124000623356551, 13.12800062354654, 13.13200062373653, 13.13600062392652, 13.14000062411651, 13.1440006243065, 13.14800062449649, 13.15200062468648, 13.15600062487647, 13.16000062506646, 13.164000625256449, 13.168000625446439, 13.172000625636429, 13.176000625826418, 13.180000626016408, 13.184000626206398, 13.188000626396388, 13.192000626586378, 13.196000626776367, 13.200000626966357, 13.204000627156347, 13.208000627346337, 13.212000627536327, 13.216000627726316, 13.220000627916306, 13.224000628106296, 13.228000628296286, 13.232000628486276, 13.236000628676265, 13.240000628866255, 13.244000629056245, 13.248000629246235, 13.252000629436225, 13.256000629626215, 13.260000629816204, 13.264000630006194, 13.268000630196184, 13.272000630386174, 13.276000630576164, 13.280000630766153, 13.284000630956143, 13.288000631146133, 13.292000631336123, 13.296000631526113, 13.300000631716102, 13.304000631906092, 13.308000632096082, 13.312000632286072, 13.316000632476062, 13.320000632666051, 13.324000632856041, 13.328000633046031, 13.33200063323602, 13.33600063342601, 13.340000633616, 13.34400063380599, 13.34800063399598, 13.35200063418597, 13.35600063437596, 13.36000063456595, 13.36400063475594, 13.368000634945929, 13.372000635135919, 13.376000635325909, 13.380000635515898, 13.384000635705888, 13.388000635895878, 13.392000636085868, 13.396000636275858, 13.400000636465847, 13.404000636655837, 13.408000636845827, 13.412000637035817, 13.416000637225807, 13.420000637415797, 13.424000637605786, 13.428000637795776, 13.432000637985766, 13.436000638175756, 13.440000638365746, 13.444000638555735, 13.448000638745725, 13.452000638935715, 13.456000639125705, 13.460000639315695, 13.464000639505684, 13.468000639695674, 13.472000639885664, 13.476000640075654, 13.480000640265644, 13.484000640455633, 13.488000640645623, 13.492000640835613, 13.496000641025603, 13.500000641215593, 13.504000641405582, 13.508000641595572, 13.512000641785562, 13.516000641975552, 13.520000642165542, 13.524000642355531, 13.528000642545521, 13.532000642735511, 13.5360006429255, 13.54000064311549, 13.54400064330548, 13.54800064349547, 13.55200064368546, 13.55600064387545, 13.56000064406544, 13.56400064425543, 13.56800064444542, 13.57200064463541, 13.576000644825399, 13.580000645015389, 13.584000645205379, 13.588000645395368, 13.592000645585358, 13.596000645775348, 13.600000645965338] format="%.2f"
  in  "FilePattern to read":path=path "*.acq"
  in  "Stastical Parameters":T2={"Min-Count"=0.0, "Max-Count"=10.0, "Step"=0.003} {"Step" format="%.4f"; "Max-Count" format="%.3f"; "Min-Count" format="%.3f"}
  out "File":path=path "C:/0/00285B.acq"
  out "Conductance (Go)":cluster{dbl, "SRat":dbl, "Filtered X":dbl[]}(graph)
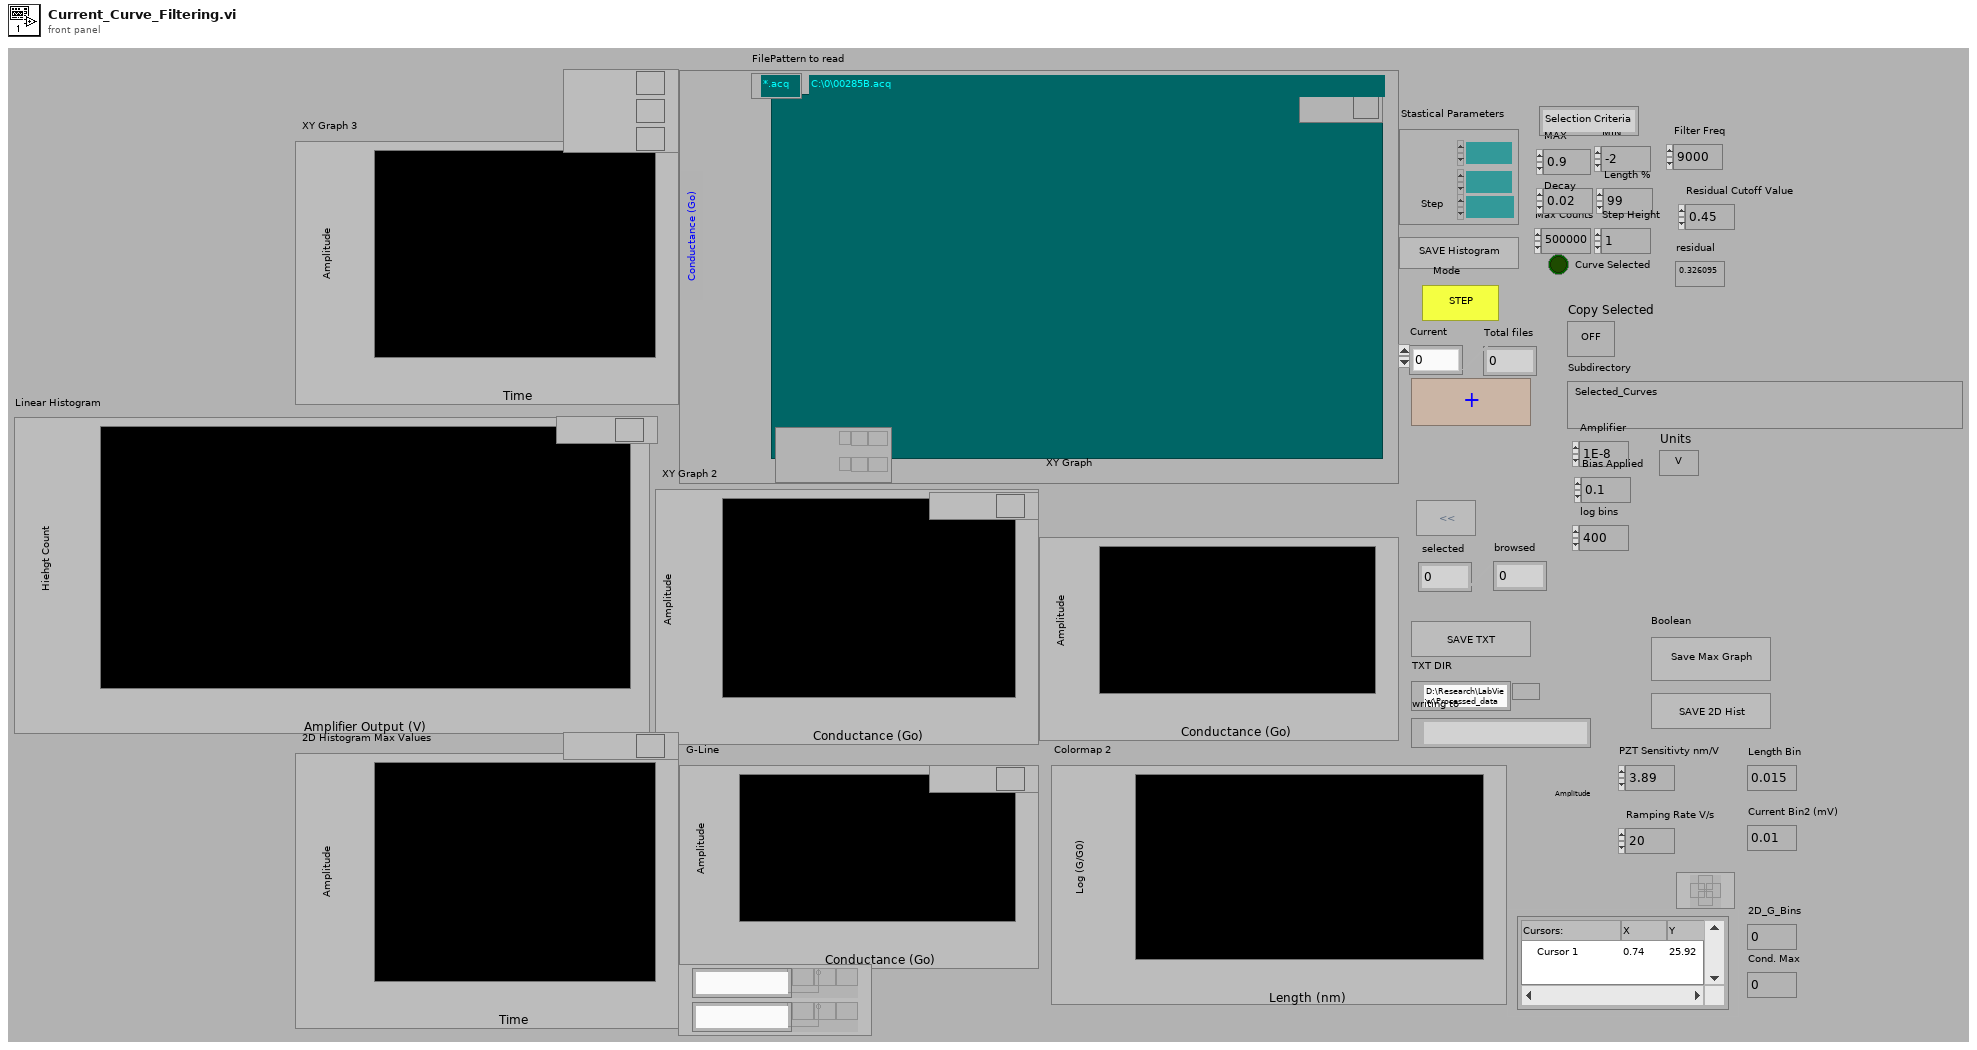
[diagram p1: front panel]
types:
  T1 = enum16{"No Correction", "DL1520-2V", "DL1520L-2V", "DL1520L-200mV"}
  T2 = cluster{"Min-Count":sgl, "Max-Count":sgl, "Step":sgl}
  T3 = cluster{"WArr":dbl[], "VDiv":dbl, "VOff":dbl, "SRat":dbl}
  T4 = cluster{"Max-Count":sgl, dbl, "Step":dbl, dbl, dbl, dbl}
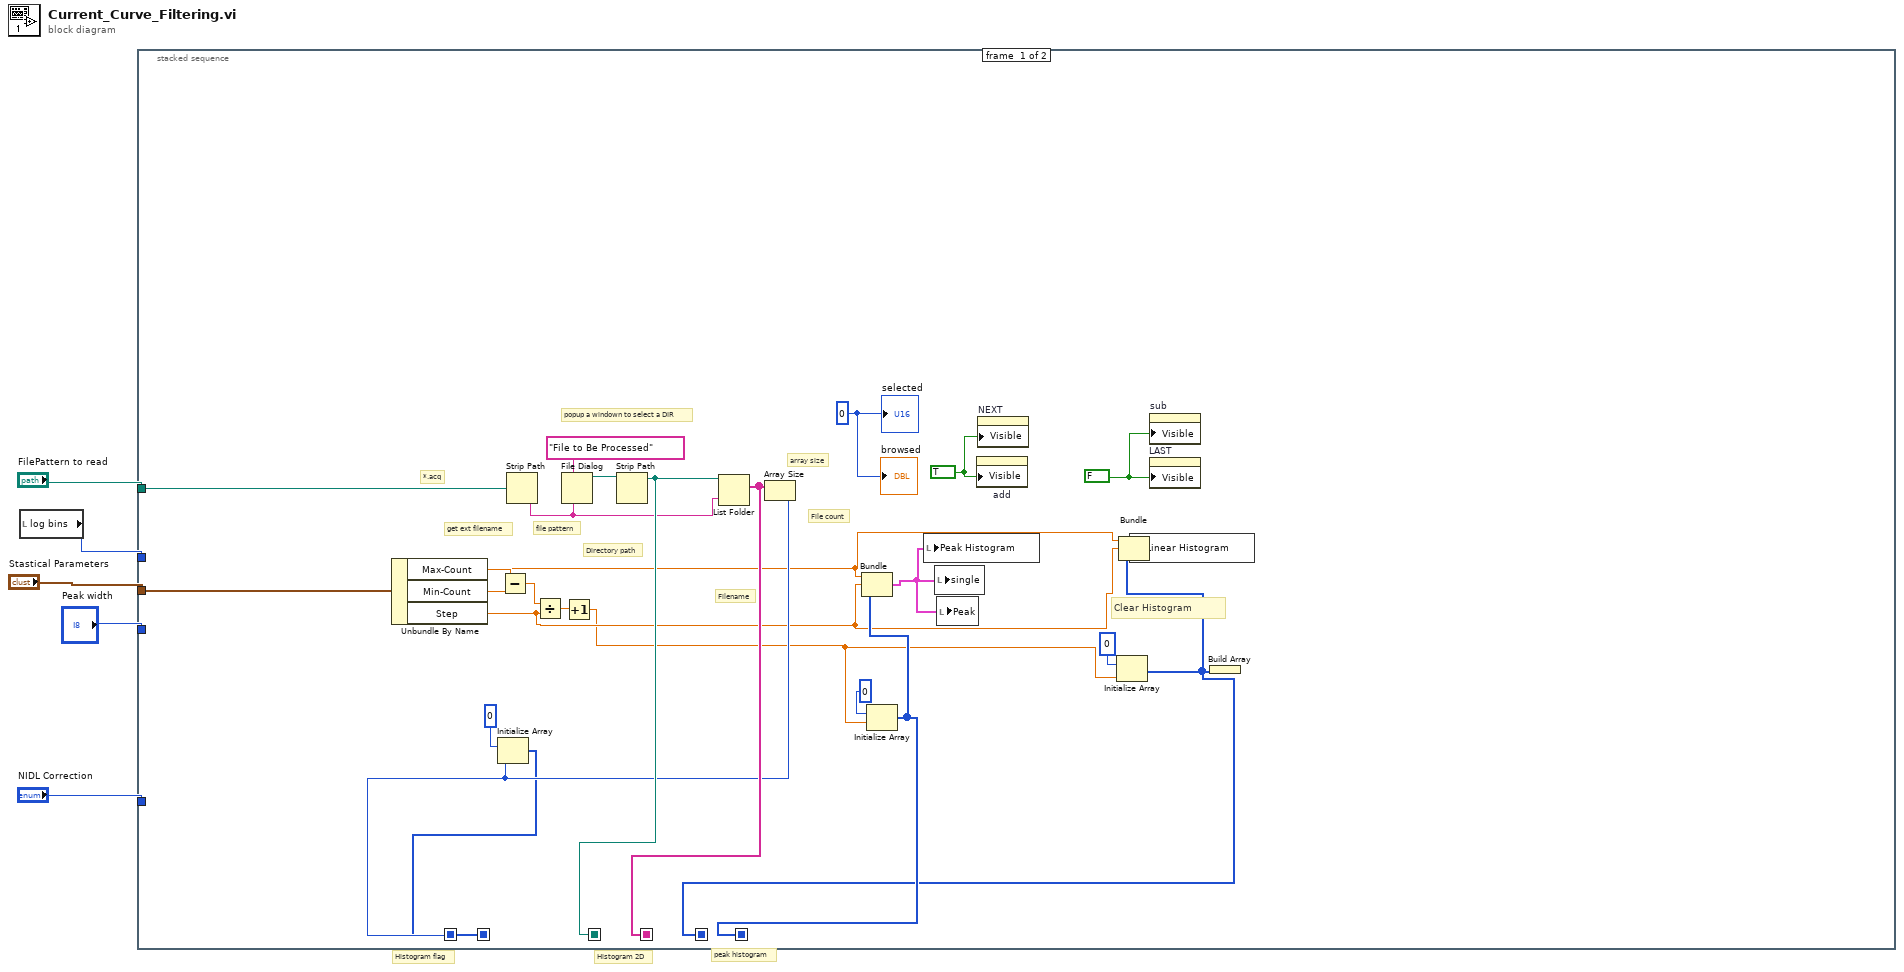
[diagram p0: block diagram]
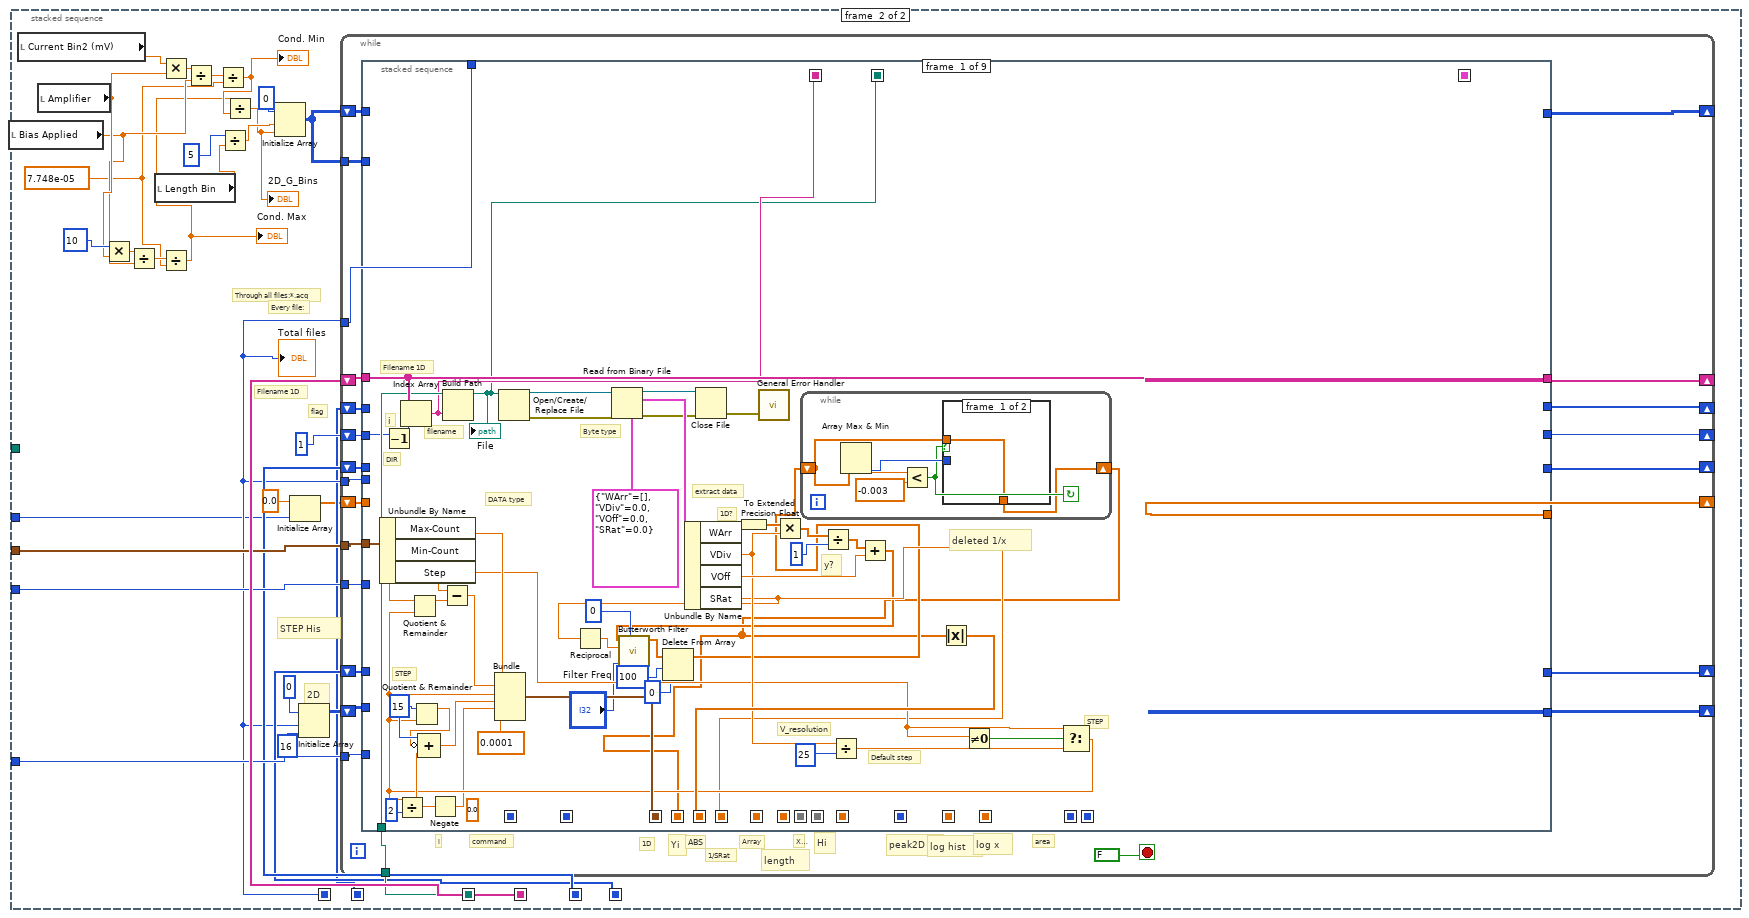
[diagram p2: hidden frame]
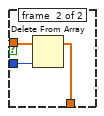
[diagram p3: hidden frame]
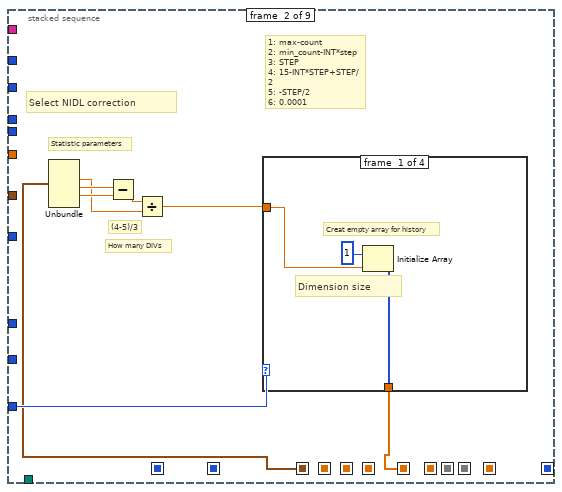
[diagram p4: hidden frame]
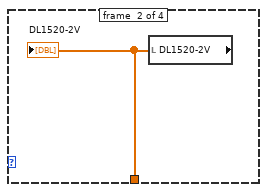
[diagram p5: hidden frame]
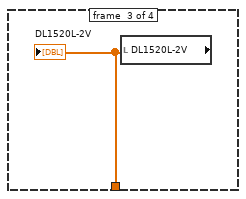
[diagram p6: hidden frame]
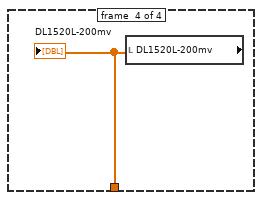
[diagram p7: hidden frame]
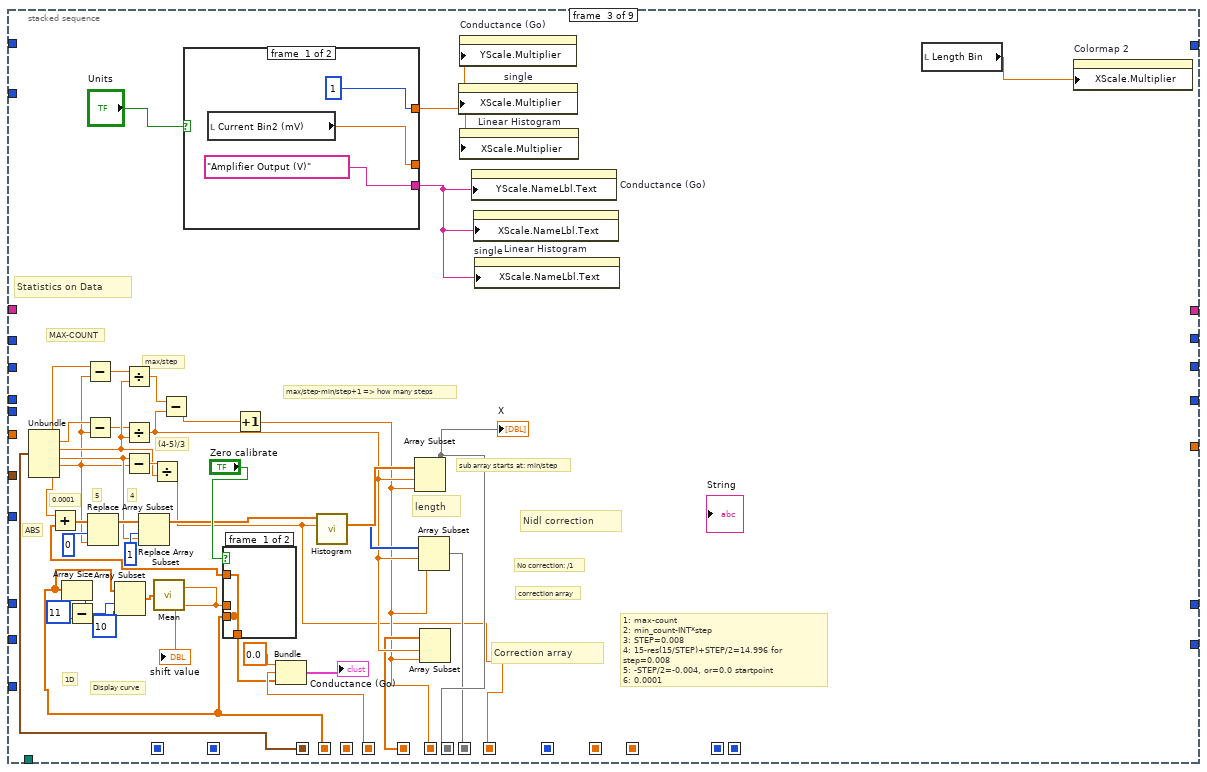
[diagram p8: hidden frame]
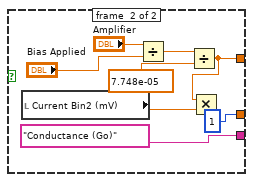
[diagram p9: hidden frame]
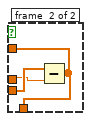
[diagram p10: hidden frame]
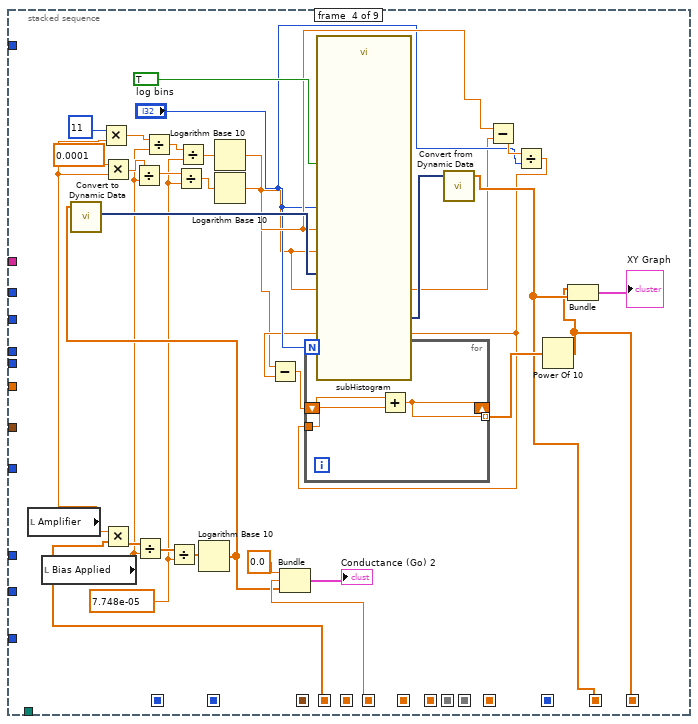
[diagram p11: hidden frame]
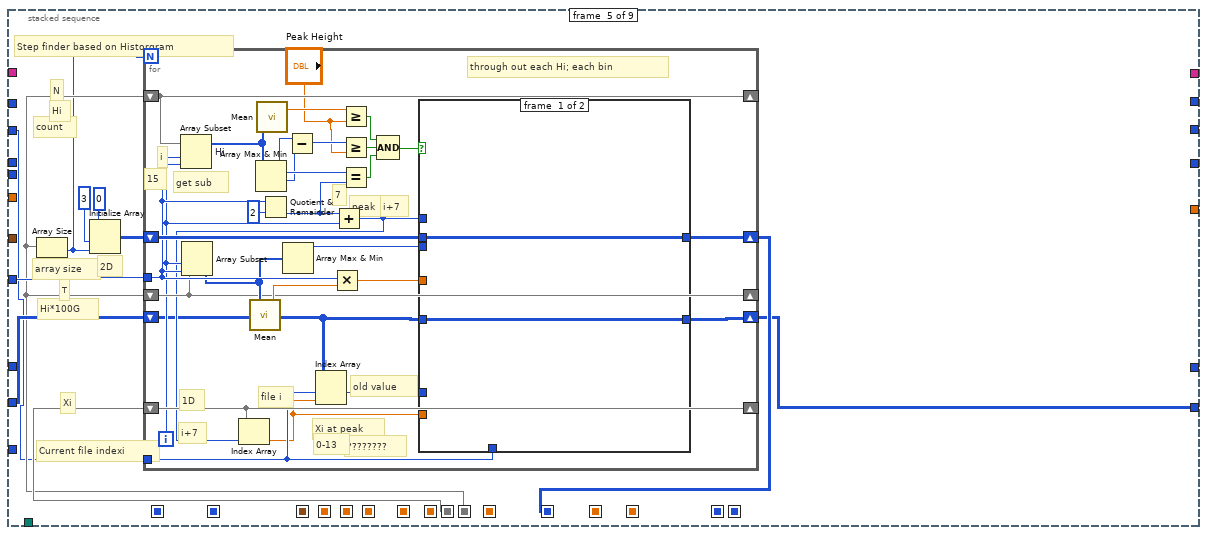
[diagram p12: hidden frame]
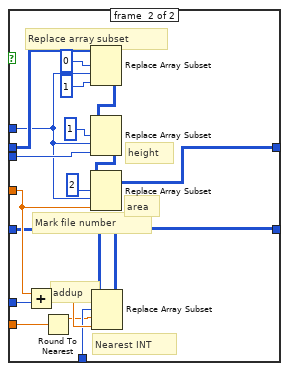
[diagram p13: hidden frame]
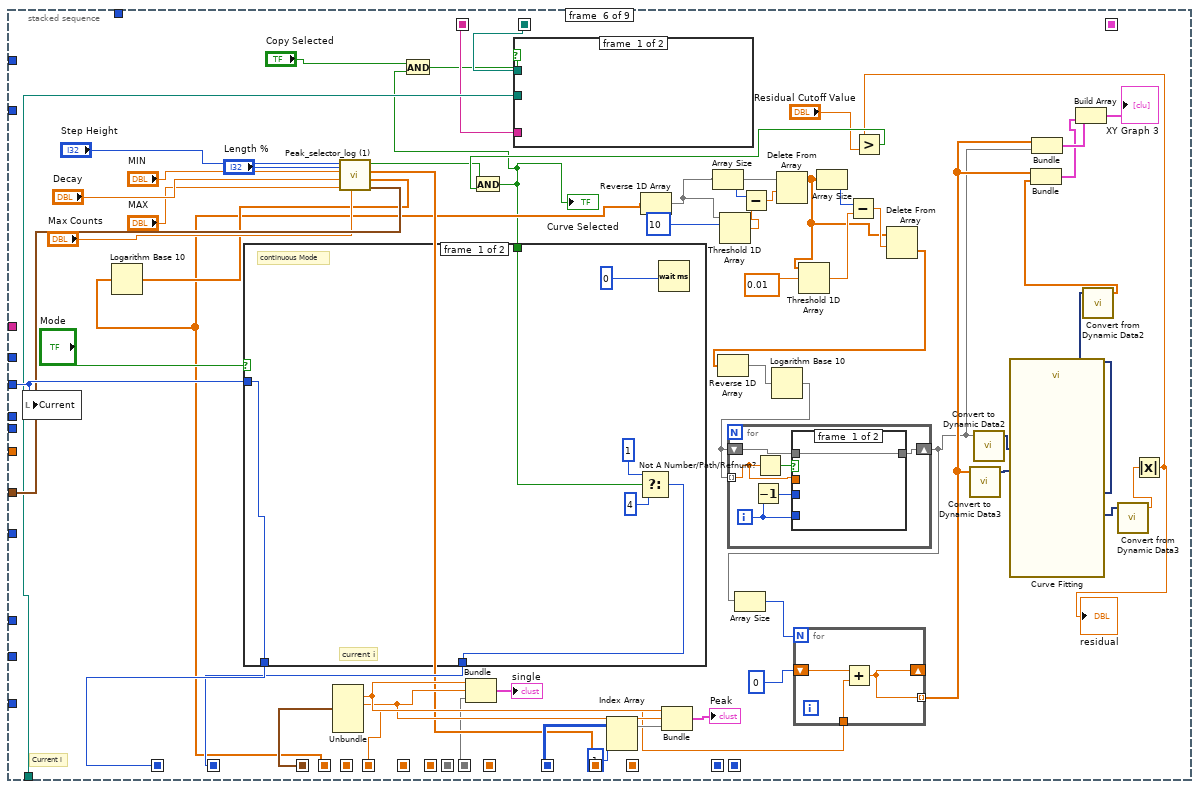
[diagram p14: hidden frame]
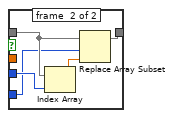
[diagram p15: hidden frame]
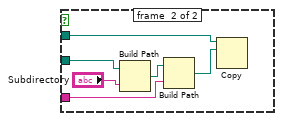
[diagram p16: hidden frame]
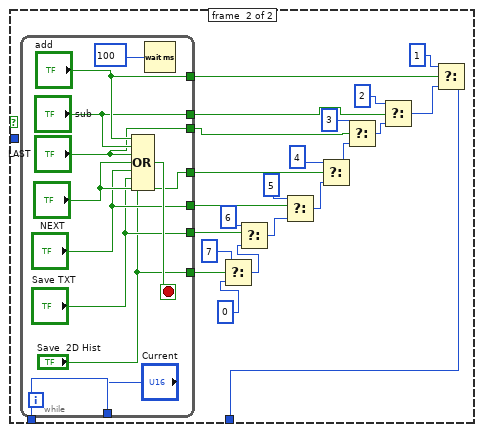
[diagram p17: hidden frame]
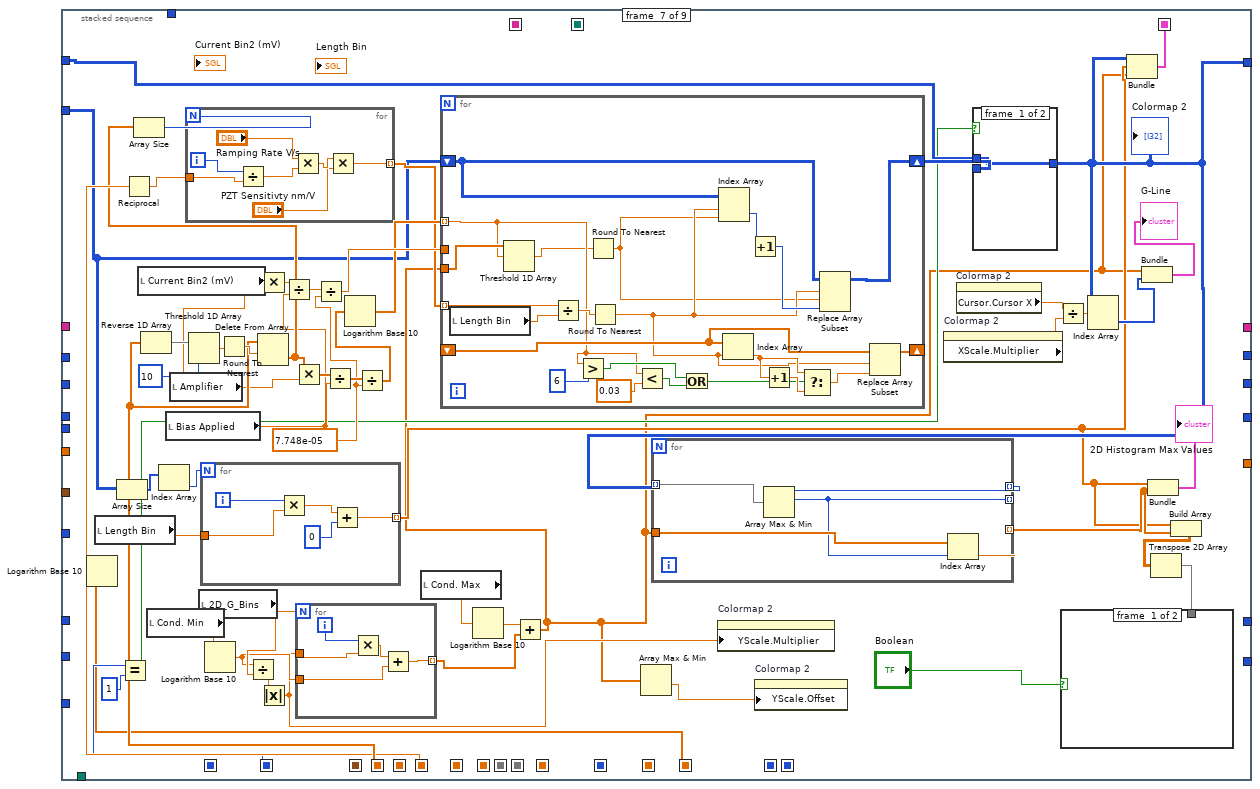
[diagram p18: hidden frame]
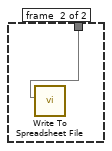
[diagram p19: hidden frame]
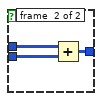
[diagram p20: hidden frame]
diagram:
  # "peak histogram"
  # "Histogram 2D"
  # "Histogram flag"
  n1 = local read "log bins"() -> (w1:i32)
  n2 = stacked-sequence {
    seq-local: [w18 _] -> [_ w52]
    seq-local: [w30 _] -> [_ w63]
    seq-local: [w29 _] -> [_ w61]
    seq-local: [w6 _] -> [_ w55]
    seq-local: [w13 _] -> [_ w54]
    seq-local: [w16 _] -> [_ w51]
    tunnel: "FilePattern to read" -> [w26 _]
    tunnel: "Stastical Parameters" -> [w24 w62]
    tunnel: "Peak width" -> [_ w57]
    tunnel: "NIDL Correction" -> [_ w56]
    tunnel: w1 -> [_ w48]
    frame #0 {
      w15 = TRUE
      w14 = FALSE
      w19 = 0
      # "Clear Histogram"
      # "File count"
      # "Filename"
      # "popup a windown to select a DIR"
      # "get ext filename"
      # "*.acq"
      # "file pattern"
      # "Directory path"
      # "array size"
      n3 = Unbundle By Name(w24) -> ("Max-Count"=w21:sgl, "Min-Count"=w11:sgl, "Step"=w10:sgl)
      n4 = Subtract(x=w21, y=w11) -> (x-y=w23:sgl)
      n5 = Strip Path(path=w26) -> (name=w25:string)  [unwired: 1 out]
      n6 = Divide(x=w23, y=w10) -> (x/y=w22:sgl)
      n7 = File Dialog(6:w25, 7:"File to Be Processed") -> (3:w28:path)  [unwired: 5 in, 3 out]
      n8 = Increment(x=w22) -> (x+1=w8:sgl)
      n9 = Strip Path(path=w28) -> (stripped path=w29:path)  [unwired: 1 out]
      n10 = List Folder(path=w29, pattern=w25) -> (filenames=w30:string[])  [unwired: 2 in, 3 out]
      n11 = Array Size(array=w30) -> (size(s)=w18:i32)
      n12 = Initialize Array(0, w18) -> (w16:i32[])
      n13 = Initialize Array(0, w8) -> (w13:i32[])
      n14 = Bundle("Min-Count"=w11, "Step"=w10, w13) -> (w12:cluster{"Min-Count":sgl, "Step":sgl, i32[]})  [unwired: 1 in]
      n15 = local write "Peak Histogram"(w12) -> ()
      n16 = local write "single"(w12) -> ()
      n17 = local write "Peak"(w12) -> ()
      n18 = property on="add" class="Boolean"("Visible"=w15) -> ()  [unwired: 2 in, 2 out]
      n19 = property on="NEXT" class="Boolean"("Visible"=w15) -> ()  [unwired: 2 in, 2 out]
      n20 = Initialize Array(0, w8) -> (w6:i32[])
      n21 = Bundle("Min-Count"=w11, "Step"=w10, w6) -> (w9:cluster{"Min-Count":sgl, "Step":sgl, i32[]})  [unwired: 1 in]
      n22 = local write "Linear Histogram"(w9) -> ()
      n23 = property on="sub" class="Boolean"("Visible"=w14) -> ()  [unwired: 2 in, 2 out]
      n24 = property on="LAST" class="Boolean"("Visible"=w14) -> ()  [unwired: 2 in, 2 out]
      n25 = Build Array(w6) -> ()  [unwired: 1 out]
      "selected" <- w19
      "browsed" <- w19
    }
    frame #1 {
      w35 = 7.748e-05
      # "flag"
      # "Every file:"
      # "STEP His"
      # "2D"
      # "Filename 1D"
      # "Through all files:*.acq"
      n26 = local read "Bias Applied"() -> (w36:dbl)
      n27 = local read "Current Bin2 (mV)"() -> (w42:sgl)
      n28 = local read "Amplifier"() -> (w37:dbl)
      n29 = Multiply(x=10, y=w37) -> (x*y=w40:dbl)
      n30 = Divide(x=w40, y=w36) -> (x/y=w39:dbl)
      n31 = local read "Length Bin"() -> (w45:sgl)
      n32 = Multiply(x=w42, y=w37) -> (x*y=w44:dbl)
      n33 = Divide(x=w39, y=w35) -> (x/y=w31:dbl)
      "Cond. Max" <- w31
      n34 = Divide(x=w44, y=w36) -> (x/y=w43:dbl)
      n35 = Divide(x=w43, y=w35) -> (x/y=w33:dbl)
      "Cond. Min" <- w33
      n36 = Divide(x=5, y=w45) -> (x/y=w34:sgl)
      n37 = Divide(x=w31, y=w33) -> (x/y=w32:dbl)
      "2D_G_Bins" <- w32
      n38 = Initialize Array(0, w34, w32) -> (w46:i32[][])
      n39 = Initialize Array(0.0, w48) -> (w50:dbl[])
      n40 = Initialize Array(0, w52, 16) -> (w59:i32[][])
      n41 = while {
        shift-right: [w86] -> _
        shift-left: w63 -> [w87]
        tunnel: w62 -> [w85]
        tunnel: w61 -> [w84]
        tunnel: w57 -> [w83]
        shift-right: [w81] -> _
        shift-left: w59 -> [w82]
        tunnel: w56 -> [w80]
        shift-right: [w72] -> _
        shift-left: w55 -> [w79]
        tunnel: w52 -> [w78]
        shift-right: [w71] -> _
        shift-left: w54 -> [w77]
        tunnel: w52 -> [w69]
        shift-right: [w74] -> _
        shift-left: 1 -> [w75]
        shift-right: [w70] -> _
        shift-left: w51 -> [w73]
        shift-right: [w67] -> _
        shift-left: w50 -> [w68]
        shift-right: [w65] -> _
        shift-left: w46 -> [w66]
        tunnel: w46 -> [w64]
        stop <- FALSE stop-if-true
        # "log x"
        # "log hist"
        # "Yi"
        # "i"
        # "command"
        # "area"
        # "peak2D"
        # "length"
        # "Hi"
        # "Xi"
        # "Array"
        # "1/SRat"
        # "ABS"
        # "1D"
        n42 = stacked-sequence {
          seq-local: [w97 _ _ _ _ _ _ _ _] -> [_ _ w183 w247 _ w345 w477 w558 _]
          seq-local: [w121 _ _ _ _ _ _ _ _] -> [_ _ _ _ _ _ _ _ _]
          seq-local: [_ _ _ _ w261 _ _ _ _] -> [_ _ _ _ _ w365 _ w554 _]
          seq-local: [_ _ w194 _ _ _ _ _ _] -> [_ _ _ _ w256 _ _ _ _]
          seq-local: [_ _ w177 _ _ _ _ _ _] -> [_ _ _ _ w255 w348 _ w545 _]
          seq-local: [w88 _ _ _ _ _ _ _ _] -> [_ _ w168 w246 _ w338 w480 w559 _]
          seq-local: [_ w154 _ _ _ _ _ _ _] -> [_ _ w188 _ _ _ _ _ _]
          seq-local: [w113 _ _ _ _ _ _ _ _] -> [_ w150 w187 _ _ w367 _ w551 _]
          seq-local: [_ _ w184 _ _ _ _ _ _] -> [_ _ _ _ _ _ _ _ _]
          seq-local: [_ _ _ _ _ w373 _ _ _] -> [_ _ _ _ _ _ _ w560 _]
          seq-local: [_ _ _ _ _ w371 _ _ _] -> [_ _ _ _ _ _ w468 w564 _]
          seq-local: [_ _ _ _ _ _ _ w553 _] -> [_ _ _ _ _ _ _ _ w710]
          seq-local: [_ _ _ _ _ _ _ w552 _] -> [_ _ _ _ _ _ _ _ w716]
          seq-local: [_ _ w165 _ _ _ _ _ _] -> [_ _ _ _ _ _ _ _ _]
          seq-local: [w99 _ _ _ _ _ _ _ _] -> [_ _ _ _ _ w353 _ _ _]
          seq-local: [w98 _ _ _ _ _ _ _ _] -> [_ _ _ _ _ w354 _ _ _]
          seq-local: [_ _ _ w221 _ _ _ _ _] -> [_ _ _ _ _ w349 _ w543 _]
          seq-local: [_ _ _ w220 _ _ _ _ _] -> [_ _ _ _ _ _ w441 w541 _]
          seq-local: [_ _ _ _ _ _ w434 _ _] -> [_ _ _ _ _ _ _ w537 _]
          tunnel: w87 -> [w126 _ _ _ _ _ _ w557 _]
          tunnel: [w126 _ _ _ _ _ _ _ _] -> w86
          tunnel: w85 -> [w120 _ _ _ _ w360 _ _ _]
          tunnel: w84 -> [w125 _ _ _ _ w355 _ _ _]
          tunnel: w83 -> [_ _ _ _ w259 _ _ _ _]
          tunnel: w82 -> [_ _ _ _ w258 _ _ _ _]
          tunnel: [_ _ _ _ w257 _ _ _ _] -> w81
          tunnel: w80 -> [_ w153 _ _ _ _ _ _ _]
          tunnel: w79 -> [_ _ _ _ _ _ _ w563 _]
          tunnel: w78 -> [_ _ _ _ _ _ _ _ _]
          tunnel: w77 -> [_ _ _ _ _ _ _ w562 _]
          tunnel: w75 -> [w102 _ _ _ w253 w370 _ _ _]
          tunnel: w69 -> [_ _ _ _ _ _ _ w556 w709]
          tunnel: [_ _ _ _ _ _ _ _ w711] -> w74
          tunnel: w73 -> [_ _ _ _ _ _ _ w561 _]
          tunnel: [_ _ _ _ _ _ _ w550 _] -> w72
          tunnel: [_ _ _ _ _ _ _ w549 _] -> w71
          tunnel: [_ _ _ _ _ _ _ w552 _] -> w70
          tunnel: [_ _ _ _ _ _ _ w540 _] -> w67
          tunnel: w68 -> [_ _ _ _ _ _ _ w542 _]
          tunnel: w66 -> [_ _ _ _ _ _ w481 _ _]
          tunnel: [_ _ _ _ _ _ w437 _ _] -> w65
          tunnel: w64 -> [_ _ _ _ _ _ w460 _ _]
          frame #0 {
            (unwired) 0.0
            w118 = 15
            # "deleted 1/x"
            # "y?"
            # "Default step"
            # "V_resolution"
            # "STEP"
            # "STEP"
            # "1D?"
            # "extract data"
            # "DATA type"
            # "Byte type"
            # "DIR"
            # "filename"
            # "i"
            # "Filename 1D"
            n43 = Unbundle By Name(w120) -> ("Max-Count"=w119:sgl, "Min-Count"=w109:sgl, "Step"=w106:sgl)
            n44 = Decrement(x=w102) -> (x-1=w101:i32)
            n45 = Index Array(array=w126, index=w101) -> (element=w99:string)
            n46 = Build Path(base path=w125, name or relative path=w99) -> (appended path=w98:path)
            "File" <- w98
            n47 = Open/Create/Replace File(file path (use dialog)=w98) -> (refnum out=w129:refnum<file>, error out=w128:errorcluster)  [unwired: 5 in, 1 out]
            n48 = Read from Binary File(5:T3 {"WArr"=[], "VDiv"=0.0, "VOff"=0.0, "SRat"=0.0}, 8:w128, 11:w129) -> (0:w124:errorcluster, 2:w127:T3, 3:w123:refnum<file>)  [unwired: 3 in, 1 out]
            n49 = Unbundle By Name(w127) -> ("WArr"=w131:dbl[], "VDiv"=w110:dbl, "VOff"=w130:dbl, "SRat"=w97:dbl)
            n50 = Reciprocal(x=w97) -> (1/x=w96:dbl)
            n51 = Close File(refnum=w123, error in=w124) -> (error out=w122:errorcluster)  [unwired: 1 out]
            n52 = To Extended Precision Float(1:w131) -> (0:w135:ext[])
            n53 = call <vilib>:"General Error Handler.vi"("error in (no error)"=w122) -> ()  [unwired: 10 in, 5 out]
            n54 = Multiply(x=w135, y=w110) -> (x*y=w134:ext[])
            n55 = Divide(x=w134, y=1) -> (x/y=w132:ext[])
            n56 = Divide(x=w110, y=25) -> (x/y=w105:dbl)
            n57 = Add(x=w132, y=w130) -> (x+y=w91:ext[])
            n58 = call-poly <vilib>:"Butterworth Filter.vi"("filter type"=0, "low cutoff freq: fl"="Filter Freq", "sampling freq: fs"=w96, "X"=w91) -> ("Filtered X"=w94:dbl[])  [unwired: 4 in, 1 out]
            n59 = Delete From Array(array=w94, length=100, index=0) -> (array with subset deleted=w90:dbl[])  [unwired: 1 out]
            n60 = while {
              shift-right: [w137] -> w88
              shift-left: w90 -> [w138]
              stop <- w139 continue-if-true
              n61 = Array Max & Min(array=w138) -> (min value=w141:dbl, min index (indices)=w140:i32)  [unwired: 2 out]
              n62 = Less?(x=w141, y=-0.003) -> (x < y?=w139:bool)
              n63 = case shown="True" w139 {
                tunnel: w140 -> [_ w146]
                tunnel: w138 -> [w143 w145]
                tunnel: [w143 w144] -> w137
                frame #0 {
                }
                frame #1 {
                  n64 = Delete From Array(array=w145, index=w146) -> (array with subset deleted=w144:dbl[])  [unwired: 1 in, 1 out]
                }
              }
            }
            n65 = Absolute Value(x=w88) -> (abs(x)=w121:dbl[])
            n66 = Not Equal To 0?(x=w106) -> (x != 0?=w104:bool)
            n67 = Select(t=w106, s=w104, f=w105) -> (s? t:f=w103:dbl)
            n68 = Divide(x=w103, y=2) -> (x/y=w116:dbl)
            n69 = Quotient & Remainder(x=w109, y=w103) -> (x-y*floor(x/y)=w108:dbl)  [unwired: 1 out]
            n70 = Quotient & Remainder(x=w118, y=w103) -> (x-y*floor(x/y)=w117:dbl)  [unwired: 1 out]
            n71 = Compound Arithmetic op=ADD(w118, invert w117, w116) -> (w114:dbl)
            n72 = Negate(x=w116) -> (-x=w100:dbl)
            n73 = Subtract(x=w109, y=w108) -> (x-y=w107:dbl)
            n74 = Bundle("Max-Count"=w119, w107, "Step"=w103, w114, w100, 0.0001) -> (w113:T4)  [unwired: 1 in]
          }
          frame #1 {
            # "How many DIVs"
            # "(4-5)/3"
            # "1: max-count\n2: min_count-INT*step\n3: STEP\n4: 15-INT*STEP+STEP/2\n5: -STEP/2\n6: 0.0001"
            # "Statistic parameters"
            # "Select NIDL correction"
            n75 = Unbundle(w150) -> ("Step"=w147:dbl, w149:dbl, w148:dbl)  [unwired: 3 out]
            n76 = Subtract(x=w149, y=w148) -> (x-y=w152:dbl)
            n77 = Divide(x=w152, y=w147) -> (x/y=w151:dbl)
            n78 = case shown="\"No Correction\"" w153 {
              tunnel: [w156 w158 w159 w160] -> w154
              tunnel: w151 -> [w155 _ _ _]
              frame #0 {
                # "Dimension size"
                # "Creat empty array for history"
                n79 = Initialize Array(1, w155) -> (w156:i32[])
              }
              frame #1 {
                n80 = local read "DL1520-2V"() -> (w158:dbl[])
                "DL1520-2V" <- w158
              }
              frame #2 {
                n81 = local read "DL1520L-2V"() -> (w159:dbl[])
                "DL1520L-2V" <- w159
              }
              frame #3 {
                n82 = local read "DL1520L-200mv"() -> (w160:dbl[])
                "DL1520L-200mv" <- w160
              }
            }
          }
          frame #2 {
            # "Correction array"
            # "correction array"
            # "No correction: /1"
            # "Nidl correction"
            # "sub array starts at: min/step"
            # "4"
            # "5"
            # "length"
            # "Display curve"
            # "0.0001"
            # "max/step-min/step+1 => how many steps"
            # "max/step"
            # "(4-5)/3"
            # "1: max-count\n2: min_count-INT*step\n3: STEP=0.008\n4: 15-res(15/STEP)+STEP/2=14.996 for step=0.008\n5: -STEP/2=-0.004, or=0.0 startpoint\n6: 0.0001"
            # "MAX-COUNT"
            # "1D"
            # "ABS"
            # "Statistics on Data"
            n83 = Unbundle(w187) -> ("Max-Count"=w180:sgl, w182:dbl, "Step"=w185:dbl, w198:dbl, w179:dbl, w186:dbl)
            n84 = Array Size(array=w168) -> (size(s)=w175:i32)
            n85 = Subtract(x=w175, y=11) -> (x-y=w176:i32)
            n86 = Subtract(x=w180, y=w179) -> (x-y=w178:dbl)
            n87 = Subtract(x=w182, y=w179) -> (x-y=w181:dbl)
            n88 = Array Subset(array=w168, index=w176, length=10) -> (w172:dbl[])
            n89 = Divide(x=w178, y=w185) -> (x/y=w196:dbl)
            n90 = Divide(x=w181, y=w185) -> (x/y=w192:dbl)
            n91 = Subtract(x=w198, y=w179) -> (x-y=w197:dbl)
            n92 = Divide(x=w197, y=w185) -> (x/y=w165:dbl)
            n93 = call <vilib>:"Mean.vi"("X"=w172) -> ("mean"=w170:dbl)  [unwired: 1 out]
            "shift value" <- w170
            n94 = Subtract(x=w196, y=w192) -> (x-y=w191:dbl)
            n95 = case shown="True" "Units" {
              tunnel: [1 w208] -> w162
              tunnel: ["Amplifier Output (V)" "Conductance (Go)"] -> w163
              tunnel: [w203 1] -> _
              frame #0 {
                n96 = local read "Current Bin2 (mV)"() -> (w203:sgl)
              }
              frame #1 {
                n97 = local read "Current Bin2 (mV)"() -> (w207:sgl)
                n98 = Divide(x="Amplifier", y="Bias Applied") -> (x/y=w211:dbl)
                n99 = Divide(x=w211, y=7.748e-05) -> (x/y=w208:dbl)
                n100 = Multiply(x=w208, y=w207) -> ()  [unwired: 1 out]
              }
            }
            n101 = case shown="True" "Zero calibrate" {
              tunnel: w168 -> [w214 w217]
              tunnel: [w214 w215] -> w169
              tunnel: w170 -> [_ w216]
              tunnel: [w214 w215] -> w167
              frame #0 {
              }
              frame #1 {
                n102 = Subtract(x=w217, y=w216) -> (x-y=w215:dbl[])
              }
            }
            n103 = Add(x=w186, y=w167) -> (x+y=w190:dbl[])
            n104 = Replace Array Subset(array=w190, new element=w179, index=0) -> (w202:dbl[])
            n105 = Replace Array Subset(array=w202, new element=w198, index=1) -> (w166:dbl[])
            n106 = Increment(x=w191) -> (x+1=w184:dbl)
            n107 = Bundle(0.0, "SRat"=w183, "Filtered X"=w169) -> (→"Conductance (Go)":cluster{dbl, "SRat":dbl, "Filtered X":dbl[]})  [unwired: 1 in]
            n108 = call <vilib>:"Histogram.vi"("intervals"=w165, "X"=w166) -> ("X Values"=w200:dbl[], "Histogram: h(x)"=w193:i32[])  [unwired: 6 in, 2 out]
            n109 = Array Subset(array=w200, index=w192, length=w184) -> (w194:dbl[])
            "X" <- w194
            n110 = Array Subset(array=w193, index=w192, length=w184) -> (w177:i32[])
            n111 = Array Subset(array=w188, index=w192, length=w184) -> ()  [unwired: 1 out]
            n112 = property on="single" class="WFGraph (strict)"("XScale.Multiplier"=w162) -> ()  [unwired: 2 in, 2 out]
            n113 = property on="Conductance (Go)" class="WFGraph (strict)"("YScale.Multiplier"=w162) -> ()  [unwired: 2 in, 2 out]
            n114 = property on="Linear Histogram" class="WFGraph (strict)"("XScale.Multiplier"=w162) -> ()  [unwired: 2 in, 2 out]
            n115 = property on="Conductance (Go)" class="WFGraph (strict)"("YScale.NameLbl.Text"=w163) -> ()  [unwired: 2 in, 2 out]
            n116 = property on="Linear Histogram" class="WFGraph (strict)"("XScale.NameLbl.Text"=w163) -> ()  [unwired: 2 in, 2 out]
            n117 = property on="single" class="WFGraph (strict)"("XScale.NameLbl.Text"=w163) -> ()  [unwired: 2 in, 2 out]
            n118 = local read "Length Bin"() -> (w161:sgl)
            n119 = property on="Colormap 2" class="IntGraph (strict)"("XScale.Multiplier"=w161) -> ()  [unwired: 2 in, 2 out]
          }
          frame #3 {
            w229 = 7.748e-05
            n120 = local read "Amplifier"() -> (w233:dbl)
            n121 = local read "Bias Applied"() -> (w231:dbl)
            n122 = Multiply(x=11, y=w233) -> (x*y=w236:dbl)
            n123 = Multiply(x=0.0001, y=w233) -> (x*y=w232:dbl)
            n124 = Multiply(x=w233, y=w246) -> (x*y=w245:dbl[])
            n125 = Divide(x=w232, y=w231) -> (x/y=w230:dbl)
            n126 = Divide(x=w245, y=w231) -> (x/y=w244:dbl[])
            n127 = Divide(x=w236, y=w231) -> (x/y=w235:dbl)
            n128 = Divide(x=w244, y=w229) -> (x/y=w243:dbl[])
            n129 = Divide(x=w230, y=w229) -> (x/y=w226:dbl)
            n130 = Divide(x=w235, y=w229) -> (x/y=w228:dbl)
            n131 = Logarithm Base 10(1:w243) -> (0:w241:dbl[])
            n132 = call "Convert to Dynamic Data"("Array"=w241) -> ("Dynamic Data Type"=w239:dynamicdata)  [unwired: 3 in]
            n133 = Logarithm Base 10(1:w228) -> (0:w227:dbl)
            n134 = Logarithm Base 10(1:w226) -> (0:w218:dbl)
            n135 = Bundle(0.0, "SRat"=w247, w241) -> (→"Conductance (Go) 2":cluster{dbl, "SRat":dbl, dbl[]})  [unwired: 1 in]
            n136 = call <vilib>:"subHistogram.vi"("Reset"=TRUE, "Number of Bins"="log bins", "Maximum Value"=w227, "Minimum Value"=w218, "Input"=w239) -> ("Histogram"=w240:dynamicdata)  [unwired: 5 in, 1 out]
            n137 = call "Convert from Dynamic Data"("Dynamic Data Type"=w240) -> ("Array"=w221:dbl[])  [unwired: 3 in]
            n138 = Subtract(x=w227, y=w218) -> (x-y=w242:dbl)
            n139 = Divide(x=w242, y="log bins") -> (x/y=w219:dbl)
            n140 = Subtract(x=w218, y=w219) -> (x-y=w223:dbl)
            n141 = for {
              N: "log bins" -> [_]
              tunnel: w219 -> [w252]
              tunnel: [w250] -> w222 mode=indexing
              shift-right: [w250] -> _
              shift-left: w223 -> [w251]
              n142 = Add(x=w251, y=w252) -> (x+y=w250:dbl)
            }
            n143 = Power Of 10(x=w222) -> (10^x=w220:dbl[])
            n144 = Bundle(w220, "Array"=w221) -> (→"XY Graph":cluster{dbl[], "Array":dbl[]})  [unwired: 1 in]
          }
          frame #4 {
            # "Current file indexi"
            # "count"
            # "2D"
            # "array size"
            # "Hi*100G"
            # "Hi"
            # "N"
            # "T"
            # "Xi"
            # "Step finder based on Historgram"
            n145 = Array Size(array=w255) -> (size(s)=w254:i32)
            n146 = Initialize Array(0, 3, w254) -> (w262:i32[][])
            n147 = for {
              N: w254 -> [_]
              shift-right: [w283] -> _
              shift-left: w255 -> [w283]
              shift-right: [w287] -> w261
              shift-left: w262 -> [w288]
              tunnel: w259 -> [w273]
              shift-right: [w277] -> _
              shift-left: w256 -> [w277]
              tunnel: w253 -> [w276]
              shift-right: [w278] -> w257
              shift-left: w258 -> [w265]
              shift-right: [w269] -> _
              shift-left: w255 -> [w269]
              i -> [w268]
              # "????????"
              # "0-13"
              # "old value"
              # "file i"
              # "Xi at peak"
              # "1D"
              # "peak"
              # "i+7"
              # "i+7"
              # "7"
              # "15"
              # "i"
              # "get sub"
              # "through out each Hi; each bin"
              n148 = Array Subset "Hi"(array=w283, index=w268, length=w273) -> (w284:i32[])
              n149 = Array Subset(array=w269, index=w268, length=w273) -> (w271:i32[])
              n150 = call <vilib>:"Mean.vi"("X"=w271) -> ("mean"=w272:dbl)  [unwired: 1 out]
              n151 = Array Max & Min(array=w284) -> (max value=w282:i32, max index (indices)=w293:i32, min value=w281:i32)  [unwired: 1 out]
              n152 = call <vilib>:"Mean.vi"("X"=w284) -> ("mean"=w274:dbl)  [unwired: 1 out]
              n153 = Quotient & Remainder(x=w273, y=2) -> (floor(x/y)=w291:i32)  [unwired: 1 out]
              n154 = Array Max & Min(array=w271) -> (max value=w270:i32)  [unwired: 3 out]
              n155 = Subtract(x=w282, y=w281) -> (x-y=w280:i32)
              n156 = Multiply(x=w273, y=w272) -> (x*y=w275:dbl)
              n157 = Add(x=w291, y=w268) -> (x+y=w267:i32)
              n158 = Index Array(array=w277, index=w267) -> (element=w266:dbl)
              n159 = Index Array(array=w265, index (row)=w276, index (col)=w266) -> (element=w279:i32)
              n160 = Greater Or Equal?(x=w274, y="Peak Height") -> (x >= y?=w290:bool)
              n161 = Greater Or Equal?(x=w280, y="Peak Height") -> (x >= y?=w286:bool)
              n162 = Equal?(x=w293, y=w291) -> (x = y?=w285:bool)
              n163 = Compound Arithmetic op=AND(w290, w286, w285) -> (w289:bool)
              n164 = case shown="True" w289 {
                tunnel: w267 -> [_ w296]
                tunnel: w288 -> [w295 w312]
                tunnel: w275 -> [_ w304]
                tunnel: [w295 w309] -> w287
                tunnel: w279 -> [_ w305]
                tunnel: w276 -> [_ w300]
                tunnel: w266 -> [_ w298]
                tunnel: w265 -> [w294 w302]
                tunnel: [w294 w301] -> w278
                tunnel: w270 -> [_ w299]
                frame #0 {
                }
                frame #1 {
                  # "Nearest INT"
                  # "addup"
                  # "Mark file number"
                  # "area"
                  # "height"
                  # "Replace array subset"
                  n165 = Add(x=w304, y=w305) -> (x+y=w303:dbl)
                  n166 = Round To Nearest(number=w298) -> (nearest integer value=w297:dbl)
                  n167 = Replace Array Subset(array=w312, new element=1, index (row)=0, index (col)=w296) -> (w311:i32[][])
                  n168 = Replace Array Subset(array=w311, new element=w299, index (row)=1, index (col)=w296) -> (w310:i32[][])
                  n169 = Replace Array Subset(array=w310, new element=w304, index (row)=2, index (col)=w296) -> (w309:i32[][])
                  n170 = Replace Array Subset(array=w302, new element=w303, index (row)=w300, index (col)=w297) -> (w301:i32[][])
                }
              }
            }
          }
          frame #5 {
            # "Current i"
            n171 = local write "Current"(w370) -> ()
            n172 = Logarithm Base 10(1:w338) -> (0:w343:dbl[])
            n173 = Unbundle(w367) -> (w359:dbl, "Step"=w358:dbl)  [unwired: 4 out]
            n174 = call "Peak_selector_log (1).vi"("Stasticl Parameters"=w360, "Array"=w343, "Array 2"=w349, "Hysteresis Spike"="Max Counts", "Length %"="Length %", "MAX"="MAX", "Cut Amount"="Decay", "MIN"="MIN", "Step Height"="Step Height") -> ("Boolean"=w317:bool)
            n175 = Bundle(w359, "Step"=w358, w348) -> (→"single":cluster{dbl, "Step":dbl, i32[]})  [unwired: 1 in]
            n176 = Index Array(array=w365, index (row)=1) -> (element=w364:i32[])  [unwired: 1 in]
            n177 = Reverse 1D Array(array=w338) -> (reversed array=w337:dbl[])
            n178 = Bundle(w359, "Step"=w358, w364) -> (→"Peak":cluster{dbl, "Step":dbl, i32[]})  [unwired: 1 in]
            n179 = Array Size(array=w337) -> (size(s)=w336:i32)
            n180 = Threshold 1D Array(2:10, 3:w337) -> (0:w335:dbl)  [unwired: 1 in]
            n181 = Subtract(x=w336, y=w335) -> (x-y=w334:dbl)
            n182 = Delete From Array(array=w337, length=w334) -> (array with subset deleted=w321:dbl[])  [unwired: 1 in, 1 out]
            n183 = Threshold 1D Array(2:0.01, 3:w321) -> (0:w331:dbl)  [unwired: 1 in]
            n184 = Array Size(array=w321) -> (size(s)=w332:i32)
            n185 = Subtract(x=w332, y=w331) -> (x-y=w330:dbl)
            n186 = Delete From Array(array=w321, length=w330) -> (deleted portion=w320:dbl[])  [unwired: 1 in, 1 out]
            n187 = Reverse 1D Array(array=w320) -> (reversed array=w319:dbl[])
            n188 = Logarithm Base 10(1:w319) -> (0:w318:dbl[])
            n189 = for {
              tunnel: w318 -> [w376] mode=indexing
              shift-right: [w375] -> w314
              shift-left: w318 -> [w379]
              i -> [w374]
              n190 = Decrement(x=w374) -> (x-1=w378:i32)
              n191 = Not A Number/Path/Refnum?(number/path/refnum=w376) -> (NaN/Path/Refnum?=w377:bool)
              n192 = case shown="True" w377 {
                tunnel: w379 -> [w380 w383]
                tunnel: w378 -> [_ w385]
                tunnel: w376 -> [_ _]
                tunnel: [w380 w382] -> w375
                tunnel: w374 -> [_ w381]
                frame #0 {
                }
                frame #1 {
                  n193 = Index Array(array=w383, index=w385) -> (element=w384:dbl)
                  n194 = Replace Array Subset(array=w383, new element=w384, index=w381) -> (w382:dbl[])
                }
              }
            }
            n195 = Array Size(array=w314) -> (size(s)=w347:i32)
            n196 = for {
              N: w347 -> [_]
              tunnel: w345 -> [w387]
              shift-right: [w386] -> _
              shift-left: 0 -> [w388]
              tunnel: [w386] -> w315 mode=indexing
              n197 = Add(x=w388, y=w387) -> (x+y=w386:dbl)
            }
            n198 = call "Convert to Dynamic Data3"("Array"=w315) -> ("Dynamic Data Type"=w328:dynamicdata)  [unwired: 3 in]
            n199 = call "Convert to Dynamic Data2"("Array"=w314) -> ("Dynamic Data Type"=w329:dynamicdata)  [unwired: 3 in]
            n200 = call "Curve Fitting"("Locations"=w328, "Signals"=w329) -> ("residual"=w325:dynamicdata, "best fit"=w327:dynamicdata)  [unwired: 4 in, 4 out]
            n201 = Bundle(w315, w314) -> (w342:cluster{dbl[], dbl[]})  [unwired: 1 in]
            n202 = call "Convert from Dynamic Data2"("Dynamic Data Type"=w327) -> ("Array"=w323:dbl[])  [unwired: 3 in]
            n203 = Bundle(w315, "Array"=w323) -> (w322:cluster{dbl[], "Array":dbl[]})  [unwired: 1 in]
            n204 = Build Array(w342, w322) -> (→"XY Graph 3":cluster{dbl[], "Array":dbl[]}[])
            n205 = call "Convert from Dynamic Data3"("Dynamic Data Type"=w325) -> ("Scalar"=w326:dbl)  [unwired: 3 in]
            n206 = Absolute Value(x=w326) -> (abs(x)=w324:dbl)
            "residual" <- w324
            n207 = Greater?(x=w324, y="Residual Cutoff Value") -> (0:w340:bool)
            n208 = And(x=w317, y=w340) -> (x .and. y?=w316:bool)
            "Curve Selected" <- w316
            n209 = case shown="True" "Mode" {
              tunnel: [w400 w423] -> w373
              tunnel: [w397 w405] -> w371
              tunnel: w370 -> [w400 _]
              tunnel: w316 -> [w395 _]
              frame #0 {
                # "current i"
                # "continuous Mode"
                n210 = Select(t=1, s=w395, f=4) -> (s? t:f=w397:i32)
                n211 = Wait (ms)(milliseconds to wait=0) -> ()  [unwired: 1 out]
              }
              frame #1 {
                n212 = while {
                  tunnel: ["add"] -> w422
                  tunnel: ["Current"] -> w423
                  tunnel: ["sub"] -> w412
                  tunnel: ["LAST"] -> w411
                  tunnel: ["NEXT"] -> w414
                  tunnel: ["?"] -> w417
                  tunnel: ["Save TXT"] -> w420
                  tunnel: ["Save  2D Hist"] -> w404
                  stop <- w432 stop-if-true
                  n213 = Compound Arithmetic op=OR("add", "sub", "LAST", "NEXT", "?", "Save TXT", "Save  2D Hist") -> (w432:bool)
                  n214 = Wait (ms)(milliseconds to wait=100) -> ()  [unwired: 1 out]
                }
                n215 = Select(t=7, s=w404, f=0) -> (s? t:f=w401:i32)
                n216 = Select(t=6, s=w420, f=w401) -> (s? t:f=w419:i32)
                n217 = Select(t=5, s=w417, f=w419) -> (s? t:f=w416:i32)
                n218 = Select(t=4, s=w414, f=w416) -> (s? t:f=w410:i32)
                n219 = Select(t=3, s=w411, f=w410) -> (s? t:f=w409:i32)
                n220 = Select(t=2, s=w412, f=w409) -> (s? t:f=w408:i32)
                n221 = Select(t=1, s=w422, f=w408) -> (s? t:f=w405:i32)
              }
            }
            n222 = And(x="Copy Selected", y=w316) -> (x .and. y?=w352:bool)
            n223 = case shown="True" w352 {
              tunnel: w355 -> [_ w394]
              tunnel: w353 -> [_ w392]
              tunnel: w354 -> [_ w390]
              frame #0 {
              }
              frame #1 {
                n224 = Build Path(base path=w394, name or relative path="Subdirectory") -> (appended path=w393:path)
                n225 = Build Path(base path=w393, name or relative path=w392) -> (appended path=w389:path)
                n226 = Copy(10:w389, 11:w390) -> ()  [unwired: 3 in, 3 out]
              }
            }
          }
          frame #6 {
            w471 = 7.748e-05
            n227 = Logarithm Base 10(1:w441) -> ()  [unwired: 1 out]
            n228 = local read "Length Bin"() -> (w452:sgl)
            n229 = Array Size(array=w460) -> (size(s)=w459:i32[])
            n230 = Equal?(x=w468, y=1) -> (x = y?=w466:bool)
            n231 = Reciprocal(x=w477) -> (1/x=w461:dbl)
            n232 = local read "Current Bin2 (mV)"() -> (w475:sgl)
            n233 = Reverse 1D Array(array=w480) -> (reversed array=w484:dbl[])
            n234 = local read "Cond. Min"() -> (w457:dbl)
            n235 = Index Array(array=w459) -> (element=w458:i32)  [unwired: 1 in]
            n236 = local read "Bias Applied"() -> (w472:dbl)
            n237 = local read "Amplifier"() -> (w474:dbl)
            n238 = Threshold 1D Array(2:10, 3:w484) -> (0:w486:dbl)  [unwired: 1 in]
            n239 = local read "2D_G_Bins"() -> (w456:dbl)
            n240 = for {
              N: w458 -> [_]
              tunnel: [w495] -> w436 mode=indexing
              tunnel: w452 -> [w498]
              i -> [w494]
              n241 = Multiply(x=w494, y=w498) -> (x*y=w497:sgl)
              n242 = Add(x=w497, y=0) -> (x+y=w495:sgl)
            }
            n243 = Logarithm Base 10(1:w457) -> (0:w455:dbl)
            n244 = Round To Nearest(number=w486) -> (nearest integer value=w485:dbl)
            n245 = Divide(x=w455, y=w456) -> (x/y=w450:dbl)
            n246 = Delete From Array(array=w480, length=w485) -> (deleted portion=w476:dbl[])  [unwired: 1 in, 1 out]
            n247 = Array Size(array=w476) -> (size(s)=w483:i32)
            n248 = for {
              N: w483 -> [_]
              tunnel: [w531] -> w462 mode=indexing
              tunnel: w461 -> [w530]
              i -> [w536]
              n249 = Divide(x=w536, y=w530) -> (x/y=w535:dbl)
              n250 = Multiply(x="Ramping Rate V/s", y=w535) -> (x*y=w533:dbl)
              n251 = Multiply(x=w533, y="PZT Sensitivty nm/V") -> (x*y=w531:dbl)
            }
            n252 = Multiply(x=w475, y=w474) -> (x*y=w473:dbl)
            n253 = Absolute Value(x=w450) -> (abs(x)=w449:dbl)
            n254 = Divide(x=w473, y=w472) -> (x/y=w470:dbl)
            n255 = Multiply(x=w476, y=w474) -> (x*y=w479:dbl[])
            n256 = for {
              N: w456 -> [_]
              tunnel: [w491] -> w451 mode=indexing
              tunnel: w455 -> [w490]
              tunnel: w449 -> [w489]
              i -> [w493]
              n257 = Multiply(x=w493, y=w489) -> (x*y=w492:dbl)
              n258 = Add(x=w492, y=w490) -> (x+y=w491:dbl)
            }
            n259 = Divide(x=w470, y=w471) -> (x/y=w469:dbl)
            n260 = Divide(x=w479, y=w472) -> (x/y=w478:dbl[])
            n261 = Divide(x=w478, y=w471) -> (x/y=w465:dbl[])
            n262 = Logarithm Base 10(1:w465) -> (0:w464:dbl[])
            n263 = local read "Cond. Max"() -> (w454:dbl)
            n264 = Logarithm Base 10(1:w454) -> (0:w453:dbl)
            n265 = Add(x=w453, y=w451) -> (x+y=w435:dbl[])
            n266 = for {
              tunnel: w464 -> [w511] mode=indexing
              tunnel: w462 -> [w528] mode=indexing
              shift-right: [w525] -> w482
              shift-left: w460 -> [w526]
              shift-right: [w521] -> _
              shift-left: _ -> [w522]
              tunnel: w469 -> [_]
              tunnel: w435 -> [w512]
              n267 = local read "Length Bin"() -> (w523:sgl)
              n268 = Threshold 1D Array(2:w511, 3:w512) -> (0:w510:dbl)  [unwired: 1 in]
              n269 = Divide(x=w528, y=w523) -> (x/y=w524:dbl)
              n270 = Greater?(x=w511, y=6) -> (0:w515:bool)
              n271 = Round To Nearest(number=w510) -> (nearest integer value=w508:dbl)
              n272 = Round To Nearest(number=w524) -> (nearest integer value=w509:dbl)
              n273 = Less?(x=w511, y=0.03) -> (x < y?=w514:bool)
              n274 = Or(x=w515, y=w514) -> (x .or. y?=w513:bool)
              n275 = Index Array(array=w526, index (row)=w509, index (col)=w508) -> (element=w529:i32)
              n276 = Index Array(array=w522, index=w509) -> (element=w518:dbl)
              n277 = Increment(x=w529) -> (x+1=w527:i32)
              n278 = Increment(x=w518) -> (x+1=w519:dbl)
              n279 = Select(t=w518, s=w513, f=w519) -> (s? t:f=w517:dbl)
              n280 = Replace Array Subset(array=w526, new element=w527, index (row)=w509, index (col)=w508) -> (w525:i32[][])
              n281 = Replace Array Subset(array=w522, new element=w517, index=w509) -> (w521:dbl[])
            }
            n282 = Array Max & Min(array=w435) -> (min value=w448:dbl)  [unwired: 3 out]
            n283 = property on="Colormap 2" class="IntGraph (strict)"("YScale.Multiplier"=w449) -> ()  [unwired: 2 in, 2 out]
            n284 = property on="Colormap 2" class="IntGraph (strict)"("YScale.Offset"=w448) -> ()  [unwired: 2 in, 2 out]
            n285 = property on="Colormap 2" class="IntGraph (strict)"() -> ("XScale.Multiplier"=w442:dbl)  [unwired: 2 in, 2 out]
            n286 = property on="Colormap 2" class="IntGraph (strict)"() -> ("Cursor.Cursor X"=w443:dbl)  [unwired: 2 in, 2 out]
            n287 = case shown="True" w466 {
              tunnel: [w504 w507] -> w437
              tunnel: w482 -> [_ w506]
              tunnel: w481 -> [w504 w505]
              frame #0 {
              }
              frame #1 {
                n288 = Add(x=w505, y=w506) -> (x+y=w507:i32[][])
              }
            }
            "Colormap 2" <- w437
            n289 = for {
              tunnel: w437 -> [w500] mode=indexing
              tunnel: [w503] -> _ mode=indexing
              tunnel: [w501] -> _ mode=indexing
              tunnel: w435 -> [w502]
              tunnel: [w499] -> w447 mode=indexing
              n290 = Array Max & Min(array=w500) -> (max value=w503:i32, max index (indices)=w501:i32)  [unwired: 2 out]
              n291 = Index Array(array=w502, index=w501) -> (element=w499:dbl)
            }
            n292 = Divide(x=w443, y=w442) -> (x/y=w439:dbl)
            n293 = Index Array(array=w437, index (row)=w439) -> (element=w440:i32[])  [unwired: 1 in]
            n294 = Bundle(w437, w436, w435) -> (w434:cluster{i32[][], sgl[], dbl[]})  [unwired: 1 in]
            n295 = Bundle(w435, w440) -> (→"G-Line":cluster{dbl[], i32[]})  [unwired: 1 in]
            n296 = Bundle(w436, w447) -> (→"2D Histogram Max Values":cluster{sgl[], dbl[]})  [unwired: 1 in]
            n297 = Build Array(w436, w447) -> (w445:dbl[][])
            n298 = Transpose 2D Array(2D array=w445) -> (transposed array=w444:dbl[][])
            n299 = case shown="True" "Boolean" {
              tunnel: w444 -> [_ w488]
              frame #0 {
              }
              frame #1 {
                n300 = call-poly <vilib>:"Write To Spreadsheet File.vi"("2D data"=w488) -> ()  [unwired: 7 in, 1 out]
              }
            }
          }
          frame #7 {
            # "i"
            # "current i"
            # "command (1-6)"
            n301 = Index Array(array=w554, index (row)=1) -> (element=w544:i32[])  [unwired: 1 in]
            n302 = case shown="5" w564 {
              tunnel: w563 -> [w567 w585 w618 w625 w631 w644 w664 w687]
              tunnel: [w567 w583 w617 w625 w631 w644 w664 w687] -> w550
              tunnel: w562 -> [w566 w582 w619 w624 w630 w650 w663 w685]
              tunnel: [w566 w581 w620 w624 w630 w650 w663 w685] -> w549
              tunnel: w545 -> [_ w584 w608 _ _ _ _ _]
              tunnel: w561 -> [w569 w576 w615 w626 w632 w652 w662 w689]
              tunnel: w560 -> [w568 w577 w612 w623 w629 w651 w665 w688]
              tunnel: [w569 w580 w614 w626 w632 w652 w662 w689] -> w552
              tunnel: [w568 w578 w612 w622 w628 w651 w665 w688] -> w553
              tunnel: w559 -> [_ _ _ _ _ _ w676 _]
              tunnel: w558 -> [_ _ _ _ _ _ w678 _]
              tunnel: w557 -> [_ _ _ _ _ _ w673 _]
              tunnel: w556 -> [_ _ _ _ _ _ _ _]
              tunnel: w544 -> [_ w579 w613 _ _ _ _ _]
              tunnel: [w565 w572 w606 w621 w627 w633 w660 w686] -> w540
              tunnel: w543 -> [_ w571 w605 _ _ _ _ _]
              tunnel: w542 -> [w565 w570 w607 w621 w627 w633 w660 w686]
              tunnel: w541 -> [_ _ _ _ _ w642 _ _]
              tunnel: w537 -> [_ _ _ _ _ _ _ w684]
              frame #0 {
                # "default: nothing"
              }
              frame #1 {
                # "add"
                n303 = Increment(x=w577) -> (x+1=w578:i32)
                n304 = Decrement(x=w577) -> (x-1=w575:i32)
                n305 = Index Array(array=w576, index=w575) -> (element=w574:i32)
                n306 = Equal To 0?(x=w574) -> (x = 0?=w573:bool)
                n307 = case shown="False" w573 {
                  tunnel: w585 -> [w588 w604]
                  tunnel: w584 -> [_ w593]
                  tunnel: [w588 w603] -> w583
                  tunnel: w582 -> [w587 w602]
                  tunnel: [w587 w601] -> w581
                  tunnel: [w589 w599] -> w580
                  tunnel: w579 -> [_ w598]
                  tunnel: w576 -> [w589 w595]
                  tunnel: w575 -> [_ w594]
                  tunnel: [w586 w592] -> w572
                  tunnel: w571 -> [_ w591]
                  tunnel: w570 -> [w586 w590]
                  frame #0 {
                  }
                  frame #1 {
                    n308 = Replace Array Subset(array=w595, new element=1, index=w594) -> (w599:i32[])
                    n309 = local read "selected"() -> (w597:u16)
                    n310 = Add(x=w604, y=w593) -> (x+y=w603:i32[])
                    n311 = Add(x=w590, y=w591) -> (x+y=w592:dbl[])
                    n312 = Increment(x=w597) -> (x+1=w596:u16)
                    n313 = local write "selected"(w596) -> ()
                    n314 = Add(x=w602, y=w598) -> (x+y=w601:i32[])
                  }
                }
              }
              frame #2 {
                # "sub"
                # "Total Histogram"
                # "flag"
                n315 = local read "selected"() -> (w610:u16)
                n316 = Decrement(x=w610) -> (x-1=w609:u16)
                n317 = Decrement(x=w612) -> (x-1=w611:i32)
                n318 = local write "selected"(w609) -> ()
                n319 = Replace Array Subset(array=w615, new element=0, index=w611) -> (w614:i32[])
                n320 = Subtract(x=w607, y=w605) -> (x-y=w606:dbl[])
                n321 = Subtract(x=w618, y=w608) -> (x-y=w617:i32[])
                n322 = Subtract(x=w619, y=w613) -> (x-y=w620:i32[])
              }
              frame #3 {
                # "last curve"
                n323 = Decrement(x=w623) -> (x-1=w622:i32)
              }
              frame #4 {
                # "NEXT curve"
                n324 = Increment(x=w629) -> (x+1=w628:i32)
              }
              frame #5 {
                (unwired) 1
                (unwired) 1
                w638 = "%.5e"
                (unwired) 0
                # "SAVE Histogram"
                n325 = local read "Linear Histogram"() -> (w646:cluster{dbl, "Step":dbl, i32[]})
                n326 = Unbundle(w646) -> (w655:dbl, "Step"=w654:dbl)  [unwired: 1 out]
                n327 = File Dialog(6:"*.txt", 9:"log_histogram.txt", 11:path "") -> (3:w634:path)  [unwired: 4 in, 3 out]
                n328 = File Dialog(6:"*.txt", 9:"histogram.txt", 11:path "") -> (3:w639:path)  [unwired: 4 in, 3 out]
                n329 = Build Array(w642, w633) -> (w641:dbl[][])
                n330 = Array Size(array=w644) -> (size(s)=w656:i32)
                n331 = for {
                  N: w656 -> [_]
                  shift-right: [w659] -> _
                  shift-left: w655 -> [w658]
                  tunnel: [w658] -> w645 mode=indexing
                  tunnel: w654 -> [w657]
                  n332 = Add(x=w658, y=w657) -> (x+y=w659:dbl)
                }
                n333 = Build Array(w645, w644) -> (w643:dbl[][])
                n334 = Transpose 2D Array(2D array=w643) -> (transposed array=w653:dbl[][])
                n335 = Transpose 2D Array(2D array=w641) -> (transposed array=w640:dbl[][])
                n336 = call-poly <vilib>:"Write To Spreadsheet File.vi"("format (%.3f)"=w638, "2D data"=w653, "file path (dialog if empty)"=w639) -> ()  [unwired: 5 in, 1 out]
                n337 = call-poly <vilib>:"Write To Spreadsheet File.vi"("format (%.3f)"=w638, "2D data"=w640, "file path (dialog if empty)"=w634) -> ()  [unwired: 5 in, 1 out]
              }
              frame #6 {
                # "data"
                # "SAVE TXT file"
                n338 = Decrement(x=w665) -> (x-1=w672:i32)
                n339 = Array Size(array=w676) -> (size(s)=w680:i32)
                n340 = Index Array(array=w673, index=w672) -> (element=w670:string)
                n341 = for {
                  N: w680 -> [_]
                  shift-right: [w683] -> _
                  shift-left: 0 -> [w682]
                  tunnel: [w682] -> w677 mode=indexing
                  tunnel: w678 -> [w681]
                  n342 = Add(x=w682, y=w681) -> (x+y=w683:dbl)
                }
                n343 = Search and Replace String(input string=w670, search string="acq", replace string="txt") -> (result string=w667:string)  [unwired: 5 in, 3 out]
                n344 = Build Array(w677, w676) -> (w675:dbl[][])
                n345 = Build Path(base path="TXT DIR", name or relative path=w667) -> (appended path=w666:path)
                "writing to" <- w666
                n346 = Transpose 2D Array(2D array=w675) -> (transposed array=w674:dbl[][])
                n347 = call-poly <vilib>:"Write To Spreadsheet File.vi"("format (%.3f)"="%.4e", "2D data"=w674, "file path (dialog if empty)"=w666) -> ()  [unwired: 5 in, 1 out]
              }
              frame #7 {
                n348 = Unbundle(w684) -> (w703:i32[][], w707:sgl[], w706:dbl[])
                n349 = Build Array (concatenate)(w706, w703) -> (w702:dbl[][])
                n350 = Transpose 2D Array(2D array=w702) -> (transposed array=w704:dbl[][])
                n351 = File Dialog(6:"*.txt", 9:"2D_hist_xy.txt", 11:path "") -> (0:w701:errorcluster, 3:w697:path)  [unwired: 4 in, 2 out]
                n352 = File Dialog(6:"*.txt", 9:"2D_hist.txt", 11:path "") -> (0:w695:errorcluster, 3:w691:path)  [unwired: 4 in, 2 out]
                n353 = Unbundle(w701) -> ()  [unwired: 3 out]
                n354 = Build Array (concatenate)(w707, w704) -> (w705:dbl[][])
                n355 = Unbundle(w695) -> ()  [unwired: 3 out]
                n356 = call-poly <vilib>:"Write To Spreadsheet File.vi"("format (%.3f)"="%.5f", "2D data"=w705, "file path (dialog if empty)"=w697) -> ()  [unwired: 5 in, 1 out]
                n357 = call-poly <vilib>:"Write To Spreadsheet File.vi"("format (%d)"="%.5f", "2D data"=w703, "file path (dialog if empty)"=w691) -> ()  [unwired: 5 in, 1 out]
              }
            }
            n358 = Unbundle(w551) -> (w547:dbl, "Step"=w546:dbl)  [unwired: 4 out]
            n359 = Bundle(w541, w540) -> (→"XY Graph 2":cluster{dbl[], dbl[]})  [unwired: 1 in]
            n360 = Bundle(w547, "Step"=w546, w550) -> (→"Linear Histogram":cluster{dbl, "Step":dbl, i32[]})  [unwired: 1 in]
            n361 = Bundle(w547, "Step"=w546, w549) -> (→"Peak Histogram":cluster{dbl, "Step":dbl, i32[]})  [unwired: 1 in]
          }
          frame #8 {
            w717 = 1
            # ">=lower limit"
            # "Upper limit overflow"
            # "In range?"
            n362 = Less Or Equal?(x=w710, y=w709) -> (x <= y?=w719:bool)
            n363 = Select(t=w710, s=w719, f=w709) -> (s? t:f=w718:i32)
            n364 = Greater Or Equal?(x=w718, y=w717) -> (x >= y?=w713:bool)
            n365 = case shown="False" w713 {
              frame #0 {
                n366 = property on="LAST" class="Bool"("Visible"=FALSE) -> ()  [unwired: 2 in, 2 out]
              }
              frame #1 {
                n367 = property on="LAST" class="Bool"("Visible"=TRUE) -> ()  [unwired: 2 in, 2 out]
              }
            }
            n368 = Select(t=w718, s=w713, f=w717) -> (s? t:f=w711:i32)
            n369 = case shown="False" w719 {
              frame #0 {
                n370 = property on="NEXT" class="Boolean"("Visible"=FALSE) -> ()  [unwired: 2 in, 2 out]
              }
              frame #1 {
                n371 = property on="NEXT" class="Boolean"("Visible"=TRUE) -> ()  [unwired: 2 in, 2 out]
              }
            }
            n372 = Decrement(x=w711) -> (x-1=w712:i32)
            n373 = Index Array(array=w716, index=w712) -> (element=w715:i32)
            n374 = Equal To 0?(x=w715) -> (x = 0?=w714:bool)
            n375 = Greater?(x=w710, y=w709) -> (0:w708:bool)
            n376 = local read "browsed"() -> (w721:dbl)
            n377 = case shown="True" w714 {
              frame #0 {
                # "sub"
                # "add"
                n378 = property on="add" class="Boolean"("Visible"=FALSE) -> ()  [unwired: 2 in, 2 out]
                n379 = property on="sub" class="Boolean"("Visible"=TRUE) -> ()  [unwired: 2 in, 2 out]
              }
              frame #1 {
                # "add"
                # "sub"
                n380 = property on="add" class="Boolean"("Visible"=TRUE) -> ()  [unwired: 2 in, 2 out]
                n381 = property on="sub" class="Boolean"("Visible"=FALSE) -> ()  [unwired: 2 in, 2 out]
              }
            }
            n382 = case shown="True" w708 {
              frame #0 {
              }
              frame #1 {
                # "CHANGE MODE TO STEP"
                n383 = local write "Mode"(TRUE) -> ()
              }
            }
            n384 = Increment(x=w721) -> (x+1=w720:dbl)
            n385 = local write "browsed"(w720) -> ()
          }
        }
      }
      "Total files" <- w52
    }
  }
